vi "WS102x FPGA Multi DUT Reliability Ver2.0.vi"() -> ()   [LabVIEW 2017]
uses:
  Type Def/Test Sequences.ctl
  WS_VCAP Driver 039/Source/WSVCAP Shell/Type Defs/WSVCAP SHL FPGA Enum.ctl
  <vilib>/userdefined/High Color/nirio_resource_hc.ctl
  WS_VCAP Driver 039/Source/WSVCAP Shell/Type Defs/WSVCAP SHL I2C DUT Mask Mode Enum.ctl
  <vilib>/Utility/error.llb/whitespace.ctl
  <vilib>/Utility/file.llb/Read Delimited Spreadsheet (DBL).vi
panel:
  out "Die Y":string[](array[string])
  out "Die X":string[](array[string])
  in  "Main":T1(tab)
  in  "Clock Rate Meas(Hz)":dbl=1000000.0 format="%.1p Hz"
  in  "CAPDAC Value":u8=128 format="0x%02x"
  in  "DUT Mask Mode (All)":T2=enum."All"
  in  "SN Brd B":string[](array[string])=["1", "2", "3", "4", "5", "6", "7", "8", "9", "10", "11", "12", "13", "14", "15", "16", "17", "18", "19", "20", "21", "22", "23", "24", "25", "26", "27", "28", "29", "30", "31", "32"]
  in  "SN Brd A":string[](array[string])=["1", "2", "3", "4", "5", "6", "7", "8", "9", "10", "11", "12", "13", "14", "15", "16", "17", "18", "19", "20", "21", "22", "23", "24", "25", "26", "27", "28", "29", "30", "31", "32"]
  in  "Info Brd B":T3={"Lot #"="1K3CB", "Wafer #"="9", "Board"="B", "Comment"="CYC 25C 44V", "File Name"="CYC_1K3CB_9_WO_25C_44V_25DC_Brd2B_190417_1", "Data File Path Control"=path "C:/WS102x 32 DUT Data"}
  in  "Info Brd A":T3={"Lot #"="3127C", "Wafer #"="11", "Board"="A", "Comment"="CYC 25C 44V", "File Name"="CYC_3127C_11_BC-C_25C_44V_8KHz_50DC_Brd7A_201215_1", "Data File Path Control"=path "C:/WS102x 32 DUT Data"}
  in  "Test Program":string="WS102x FPGA Multi DUT Reliability Ver2.0"
  in  "Calibration AD":bool
  in  "Initialize ADI":bool
  in  "Data Brd B?":bool
  in  "Data Brd A?":bool=TRUE
  in  "Setup Test":T4(tab)
  in  "Manual Command":string
  in  "Verify Beams":bool
  in  "Manual Setting":i32(ring) items=["CP OFF", "CP ON", "OTP OFF", "CP 24V", "CP 26V", "CP 28V", "CP 30V", "CP 31V", "CP 32V", "CP 33V", "CP 34V", "CP 35V", "CP 36V", "CP 37V", "CP 38V", "CP 39V", "CP 40V", "CP 41V", "CP 42V", "CP 43V", "CP 44V", "CP 45V", "CP 46V", "CP 47V", "CP 48V", "CP 49V", "CP 50V", "CP 51V", "CP 52V", "CP 53V", "CP 54V", "CP 56V", "CP 58V", "CP 60V", "CP 62V"]
  in  "CP Measurement":i32(ring)=20 items=["CP OFF", "CP ON", "OTP OFF", "CP 24V", "CP 26V", "CP 28V", "CP 30V", "CP 31V", "CP 32V", "CP 33V", "CP 34V", "CP 35V", "CP 36V", "CP 37V", "CP 38V", "CP 39V", "CP 40V", "CP 41V", "CP 42V", "CP 43V", "CP 44V", "CP 45V", "CP 46V", "CP 47V", "CP 48V", "CP 49V", "CP 50V", "CP 51V", "CP 52V", "CP 53V", "CP 54V", "CP 56V", "CP 58V", "CP 60V", "CP 62V"]
  in  "Select CP VPI":i32(ring)=16 items=["CP OFF", "CP ON", "OTP OFF", "CP 24V", "CP 26V", "CP 28V", "CP 30V", "CP 31V", "CP 32V", "CP 33V", "CP 34V", "CP 35V", "CP 36V", "CP 37V", "CP 38V", "CP 39V", "CP 40V", "CP 41V", "CP 42V", "CP 43V", "CP 44V", "CP 45V", "CP 46V", "CP 47V", "CP 48V", "CP 49V", "CP 50V", "CP 51V", "CP 52V", "CP 53V", "CP 54V", "CP 56V", "CP 58V", "CP 60V", "CP 62V"]
  in  "Select CP Stress":i32(ring)=20 items=["CP OFF", "CP ON", "OTP OFF", "CP 24V", "CP 26V", "CP 28V", "CP 30V", "CP 31V", "CP 32V", "CP 33V", "CP 34V", "CP 35V", "CP 36V", "CP 37V", "CP 38V", "CP 39V", "CP 40V", "CP 41V", "CP 42V", "CP 43V", "CP 44V", "CP 45V", "CP 46V", "CP 47V", "CP 48V", "CP 49V", "CP 50V", "CP 51V", "CP 52V", "CP 53V", "CP 54V", "CP 56V", "CP 58V", "CP 60V", "CP 62V"]
  in  "VDD":dbl=3.3 format="%.2g"
  in  "CP Setting":bool
  in  "Delay Setting":T5(ring)
  in  "HD Cmd":string="0701027F7F"
  in  "Cycle DC %":string="50"
  in  "Set Delay Speed":dbl[](array[numeric])=[5.4e-05, 5.4e-05] min=0.0 max=0.5 format="%#.0p s"
  in  "Cycling Bit":string[](array[string])=["0701027F7F", "0701020000"]
  out "Stress DC(%)":string
  in  "HD Beams":string="ALL Beams"
  in  "Test Condition Setting":T6={"Freq (KHz)"="8", "ACV (V)"="0", "AC Freq (Hz)"="0", "Temp (C)"="25", "DCV (V)"=0.0, "CYC RP (x1000)"=10000, "HD RP (Min)"=60, "RPM Delay (s)"=60, "Select VCmin"=2} {"Select VCmin" items=["FBs", "TBs", "ALL"]}
  out "Test Run Selected":T7
  in  "Test Run Setting":T8={"OTP ?  "=FALSE, "STRESS ?  "=TRUE, "VPI ?  "=TRUE, "OPEN STATE VCMIN ?  "=FALSE, "CLOSE STATE VCMIN ?  "=TRUE, "RPM (Verify Socket) ?  "=FALSE, "HS CHK?"=FALSE}
  out "Data Board B":string[][](array[string])
  in  "Stop":bool
  out "Current Time":string
  out "Current Date":string
  in  "Start Date":string
  in  "Start Time":string
  in  "Select Measurement":i32(ring) items=["Temperature", "Humidity", "TH1", "TH2"]
  out "Temp (C)":string
  out "RH(%)":string
  out "Test Sequences":T9
  out "Error Out":errorcluster
  in  "Error In":errorcluster
  in  "Start":bool
  out "Data Board A":string[][](array[string])
  out "AD7747 Value Brd B":string[][](table)=[["Device", "Status", "Cap (pF)", "SN"], ["DUT 01", "", "", "01"], ["DUT 02", "", "", "02"], ["DUT 03", "", "", "03"], ["DUT 04", "", "", "04"], ["DUT 05", "", "", "05"], ["DUT 06", "", "", "06"], ["DUT 07", "", "", "07"], ["DUT 08", "", "", "08"], ["DUT 09", "", "", "09"], ["DUT 10", "", "", "10"], ["DUT 11", "", "", "11"], ["DUT 12", "", "", "12"], ["DUT 13", "", "", "13"], ["DUT 14", "", "", "14"], ["DUT 15", "", "", "15"], ["DUT 16", "", "", "16"], ["DUT 17", "", "", "17"], ["DUT 18", "", "", "18"], ["DUT 19", "", "", "19"], ["DUT 20", "", "", "20"], ["DUT 21", "", "", "21"], ["DUT 22", "", "", "22"], ["DUT 23", "", "", "23"], ["DUT 24", "", "", "24"], ["DUT 25", "", "", "25"], ["DUT 26", "", "", "26"], ["DUT 27", "", "", "27"], ["DUT 28", "", "", "28"], ["DUT 29", "", "", "29"], ["DUT 30", "", "", "30"], ["DUT 31", "", "", "31"], ["DUT 32", "", "", "32"]]
  out "AD7747 Value Brd A":string[][](table)=[["Device", "Status", "Cap (pF)", "SN"], ["DUT 01", "", "", "01"], ["DUT 02", "", "", "02"], ["DUT 03", "", "", "03"], ["DUT 04", "", "", "04"], ["DUT 05", "", "", "05"], ["DUT 06", "", "", "06"], ["DUT 07", "", "", "07"], ["DUT 08", "", "", "08"], ["DUT 09", "", "", "09"], ["DUT 10", "", "", "10"], ["DUT 11", "", "", "11"], ["DUT 12", "", "", "12"], ["DUT 13", "", "", "13"], ["DUT 14", "", "", "14"], ["DUT 15", "", "", "15"], ["DUT 16", "", "", "16"], ["DUT 17", "", "", "17"], ["DUT 18", "", "", "18"], ["DUT 19", "", "", "19"], ["DUT 20", "", "", "20"], ["DUT 21", "", "", "21"], ["DUT 22", "", "", "22"], ["DUT 23", "", "", "23"], ["DUT 24", "", "", "24"], ["DUT 25", "", "", "25"], ["DUT 26", "", "", "26"], ["DUT 27", "", "", "27"], ["DUT 28", "", "", "28"], ["DUT 29", "", "", "29"], ["DUT 30", "", "", "30"], ["DUT 31", "", "", "31"], ["DUT 32", "", "", "32"]]
  in  "Instruments":T11={"KE2400"="GPIB0::3::INSTR", "KE2000"="GPIB0::9::INSTR", "Agilent P/S"="GPIB0::5::INSTR", "Temperature Sensor"="", "FPGA"=enum."RIO0"}
  out "Activity Log":string
  out "FPGA Resource":T12
  out "Online":bool
  out "Simulate FPGA":bool
  in  "RFFE Slave Address":u8=7 caption="Slave Address" format="0x%02x"
  in  "Clock Rate Cycle(Hz)":dbl=5000000.0 format="%.1p Hz"
  out "Error Status":string
  out "IDD Measurement(uA)":string[](array[string])
  out "Cycle Count":u64=2 min=1 max=4 step=1
  out "Status":string
  out "Last Run Time":string
  out "Last Run Date":string
  out "T0_Brd B Delta C%":string[](array[string])
  out "T0_Brd A Delta C%":string[](array[string])
  in  "Abort Stress":bool
  out "TTF Completed":u64
  in  "Set TTF":u64=50000000000
  out "Brd B_VPI Cap (fF)":string[][](table)
  out "Brd B_Beam Cap (fF)":string[][](table)
  out "Brd A_VPI Cap (fF)":string[][](table)
  out "Brd A_Beam Cap (fF)":string[][](table)
  out "Verify CP Stress":string[](array[string])
  out "Brd B Pass/Fail?":bool[](array[boolean])
  out "Brd A Pass/Fail?":bool[](array[boolean])
  out "Verify DC Speed":dbl[](array[numeric]) format="%#.0p s"
  out "Verify Bits to Cycle":string[](array[string])
  out "Brd A Delta C%":string[](array[string])
  out "Brd B Delta C%":string[](array[string])
  out "Brd B_OS_V3 (fF)":string[][](table)
  out "Brd B_OS_V2 (fF)":string[][](table)
  out "Brd B_OS_V1 (fF)":string[][](table)
  in  "OS_Voltage(V)":dbl[](array[numeric])=[-10.0, 0.0, 10.0]
  out "Brd A_OS_V3 (fF)":string[][](table)
  out "Brd A_OS_V2 (fF)":string[][](table)
  out "Brd A_OS_V1 (fF)":string[][](table)
  out "VPI Brd B Delta C%":string[](array[string])
  out "VPI Brd A Delta C%":string[](array[string])
  out "Cmin BrdB":string[](array[string])
  out "Cmin BrdA":string[](array[string])
  out "RB for HD Stress":string[][](array[string])
  out "Brd B_CS_V3 (fF)":string[][](table)
  out "Brd B_CS_V2 (fF)":string[][](table)
  out "Brd B_CS_V1 (fF)":string[][](table)
  out "Brd A_CS_V3 (fF)":string[][](table)
  out "Brd A_CS_V2 (fF)":string[][](table)
  out "Brd A_CS_V1 (fF)":string[][](table)
  in  "CS_Voltage(V)":dbl[](array[numeric])=[-3.0, 0.0, 3.0]
  out "CMin BrdA (fF)":dbl[](array[numeric])
  out "CMin BrdB (fF)":dbl[](array[numeric])
  out "RB Die Y\nBrd B":string[](array[string])
  out "RB Die X\nBrd B":string[](array[string])
  out "RB Die Y\nBrd A":string[](array[string])
  out "Brd B_CS VCmin":string[][](table)
  out "Brd A_CS VCmin":string[][](table)
  out "Brd B_CS VCmin_T0":string[][](table)
  out "Brd A_CS VCmin_T0":string[][](table)
  out "RB Die X\nBrd A":string[](array[string])
  in  "RB Die Location?":bool=TRUE
  in  "Col CMin":i32=29
  out "Board B":dbl[][](graph)
  out "Board A":dbl[][](graph)
  in  "Plot":T13(ring)
  # "Company: WiSpry Inc Powered by AAC Technologies\n20 Fairbanks Suite 198, Irvine CA 92618\n\nCreated Date:  11-2-2021\nTP:  WS1021 32 DUT Board, Reliability Ver2.0\nFPGA Modular:  WS_VCAP_Driver 039"
  # "WS1021 FPGA 32 DUT Reliability Version Updated note:\n\n1. Ver1.0 :  Original version to run HD only (1-24-2019)\n2. Ver1.5 :  Delay Setting; Added CN, CMax (Total) and Cmin2 (12/15/2020), Minerva1"
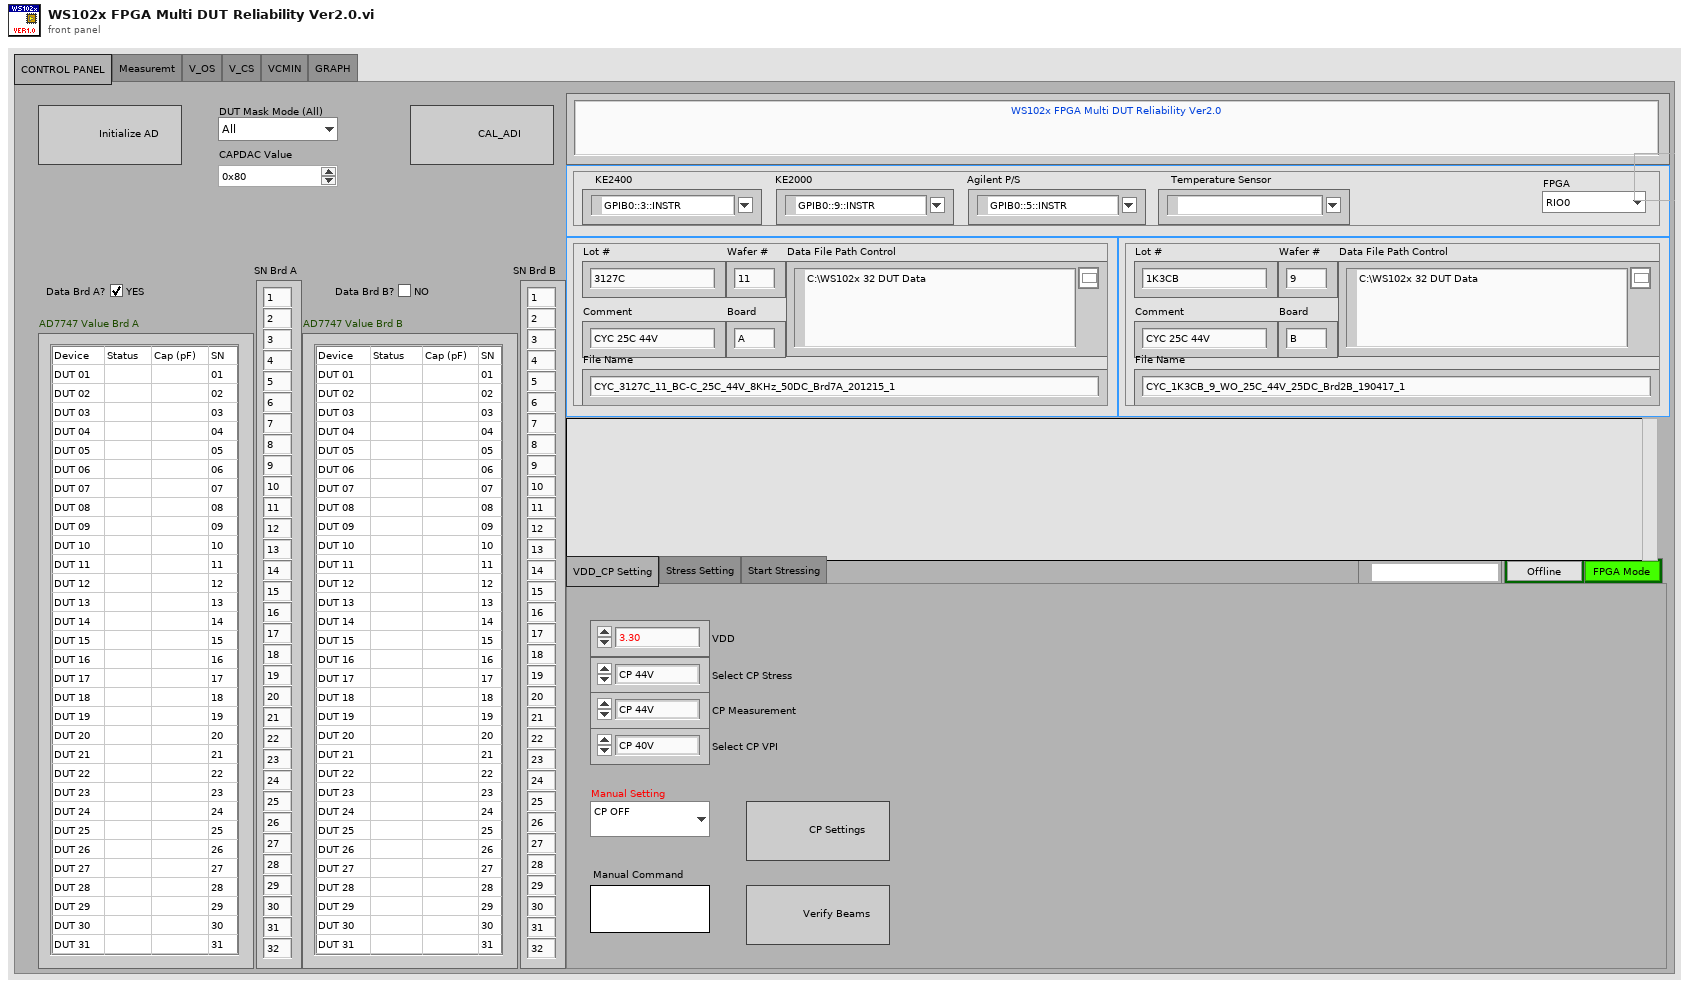
[diagram p1: front panel]
types:
  T1 = enum32{"CONTROL PANEL", "Measuremt", "V_OS", "V_CS", "VCMIN", "GRAPH"}
  T2 = typedef "WSVCAP SHL I2C DUT Mask Mode Enum.ctl" = enum16{"Custom", "All"}
  T3 = cluster{"Lot #":string, "Wafer #":string, "Board":string, "Comment":string, "File Name":string, "Data File Path Control":path}
  T4 = enum32{"VDD_CP Setting", "Stress Setting", "Start Stressing"}
  T5 = enum16{"Default (2.5us)", "0us", "4.8us", "5.26us"}
  T6 = cluster{"Freq (KHz)":string, "ACV (V)":string, "AC Freq (Hz)":string, "Temp (C)":string, "DCV (V)":dbl, "CYC RP (x1000)":u64, "HD RP (Min)":u64, "RPM Delay (s)":u64, "Select VCmin":u16}
  T7 = cluster{"OTP":bool, "CYC/HD":bool, "VPI":bool, "OSV":bool, "CSV":bool, "RPM":bool, "HS CHK":bool}
  T8 = cluster{"OTP ?  ":bool, "STRESS ?  ":bool, "VPI ?  ":bool, "OPEN STATE VCMIN ?  ":bool, "CLOSE STATE VCMIN ?  ":bool, "RPM (Verify Socket) ?  ":bool, "HS CHK?":bool}
  T9 = typedef "Test Sequences.ctl" = enum16{"VDD", "CP Setting", "HS CHK", "Stress", "I_Measure", "Cap_Measure", "VPI", "Open State VCmin", "Close State VCmiin", "Save Data", "Exit"}
  T10 = typedef "WSVCAP SHL FPGA Enum.ctl" = enum16{"RIO0", "RIO1"}
  T11 = cluster{"KE2400":refnum<visa-resource-name>, "KE2000":refnum<visa-resource-name>, "Agilent P/S":refnum<visa-resource-name>, "Temperature Sensor":refnum<visa-resource-name>, "FPGA":T10}
  T12 = typedef "nirio_resource_hc.ctl" = tag
  T13 = enum16{"ALL DUTs", "DUT 01", "DUT 02", "DUT 03", "DUT 04", "DUT 05", "DUT 06", "DUT 07", "DUT 08", "DUT 09", "DUT 10", "DUT 11", "DUT 12", "DUT 13", "DUT 14", "DUT 15", "DUT 16", "DUT 17", "DUT 18", "DUT 19", "DUT 20", "DUT 21", "DUT 22", "DUT 23", "DUT 24", "DUT 25", "DUT 26", "DUT 27", "DUT 28", "DUT 29", "DUT 30", "DUT 31", "DUT 32"}
  T14 = enum16{"Idle...", "Voltage 1", "Voltage 2", "Voltage 3"}
  T15 = typedef "WSVCAP SHL Core System Cluster.ctl" = cluster{"Settings":T16, "FPGA Resource":tag, "Online":bool, "I2C Wait Ticks":u32, "SPI Wait Ticks":u32, "RFFE Wait Ticks":u32, "FPGA VI Reference (FPGA Mode)":T17, "FPGA VI Reference (Sim Mode)":refnum<vi>}
  T16 = typedef "WSVCAP SHL I2C Settings Cluster.ctl" = cluster{"I2C Slave Address":u8, "I2C Clock Rate (Hz)":dbl, "SPI Clock Rate (Hz)":dbl, "RFFE Slave Address":u8, "RFFE Clock Rate (Hz)":dbl, "Simulate FPGA":bool, "C1 Cap DAC Default":u8, "C2 Cap DAC Default":u8, "C3 Cap DAC Default":u8, "C4 Cap DAC Default":u8}
  T17 = typedef "WSVCAP SHL FPGA Ref.ctl" = refnum<k20>
  T18 = enum16{"Idle...", "Voltage 1", "Voltage 2", "Voltage 3"}[]
  T19 = typedef "whitespace.ctl" = u16
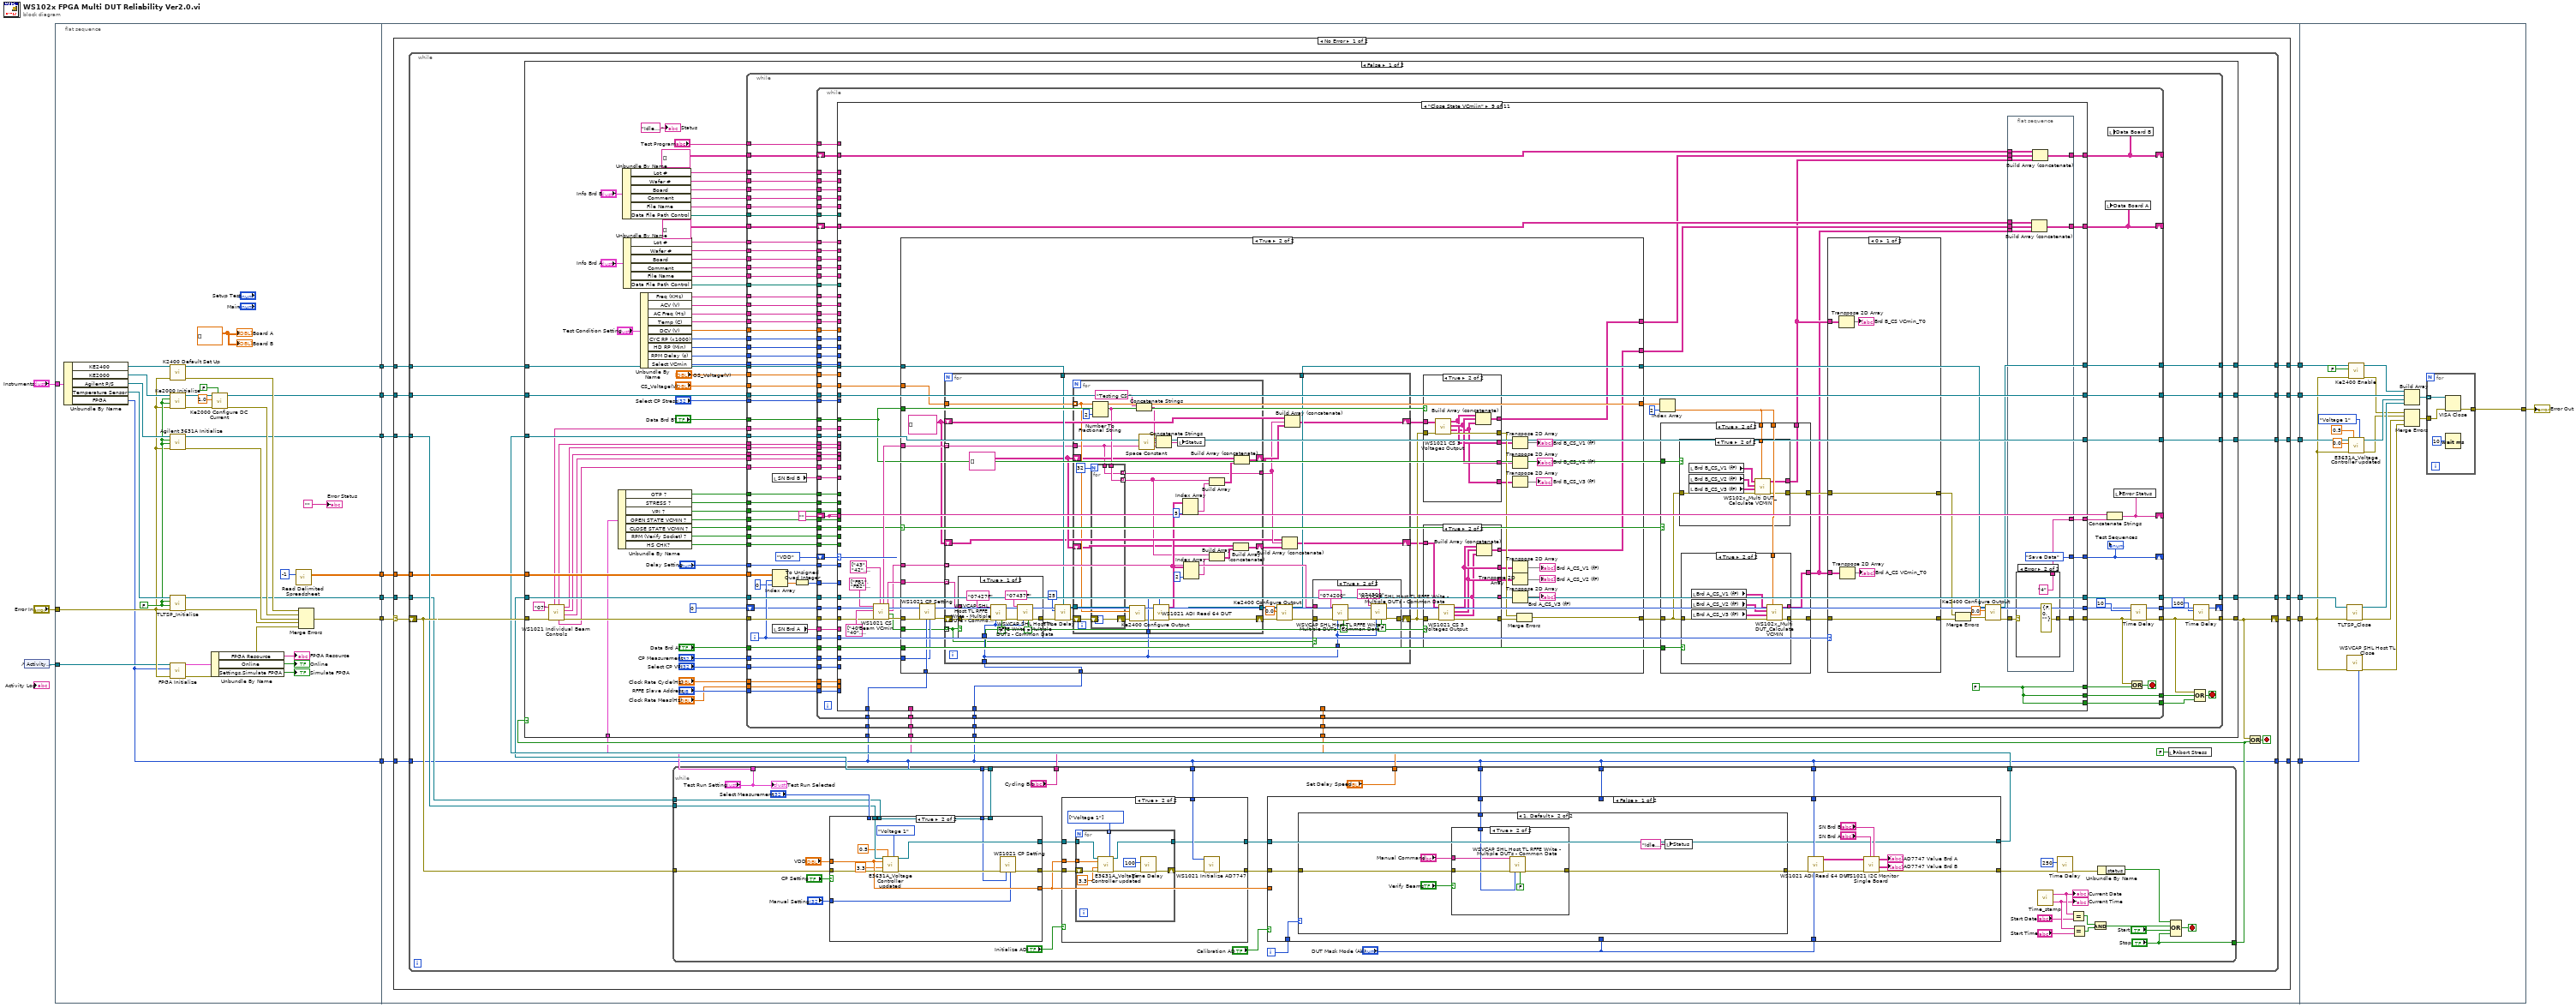
[diagram p0: block diagram]
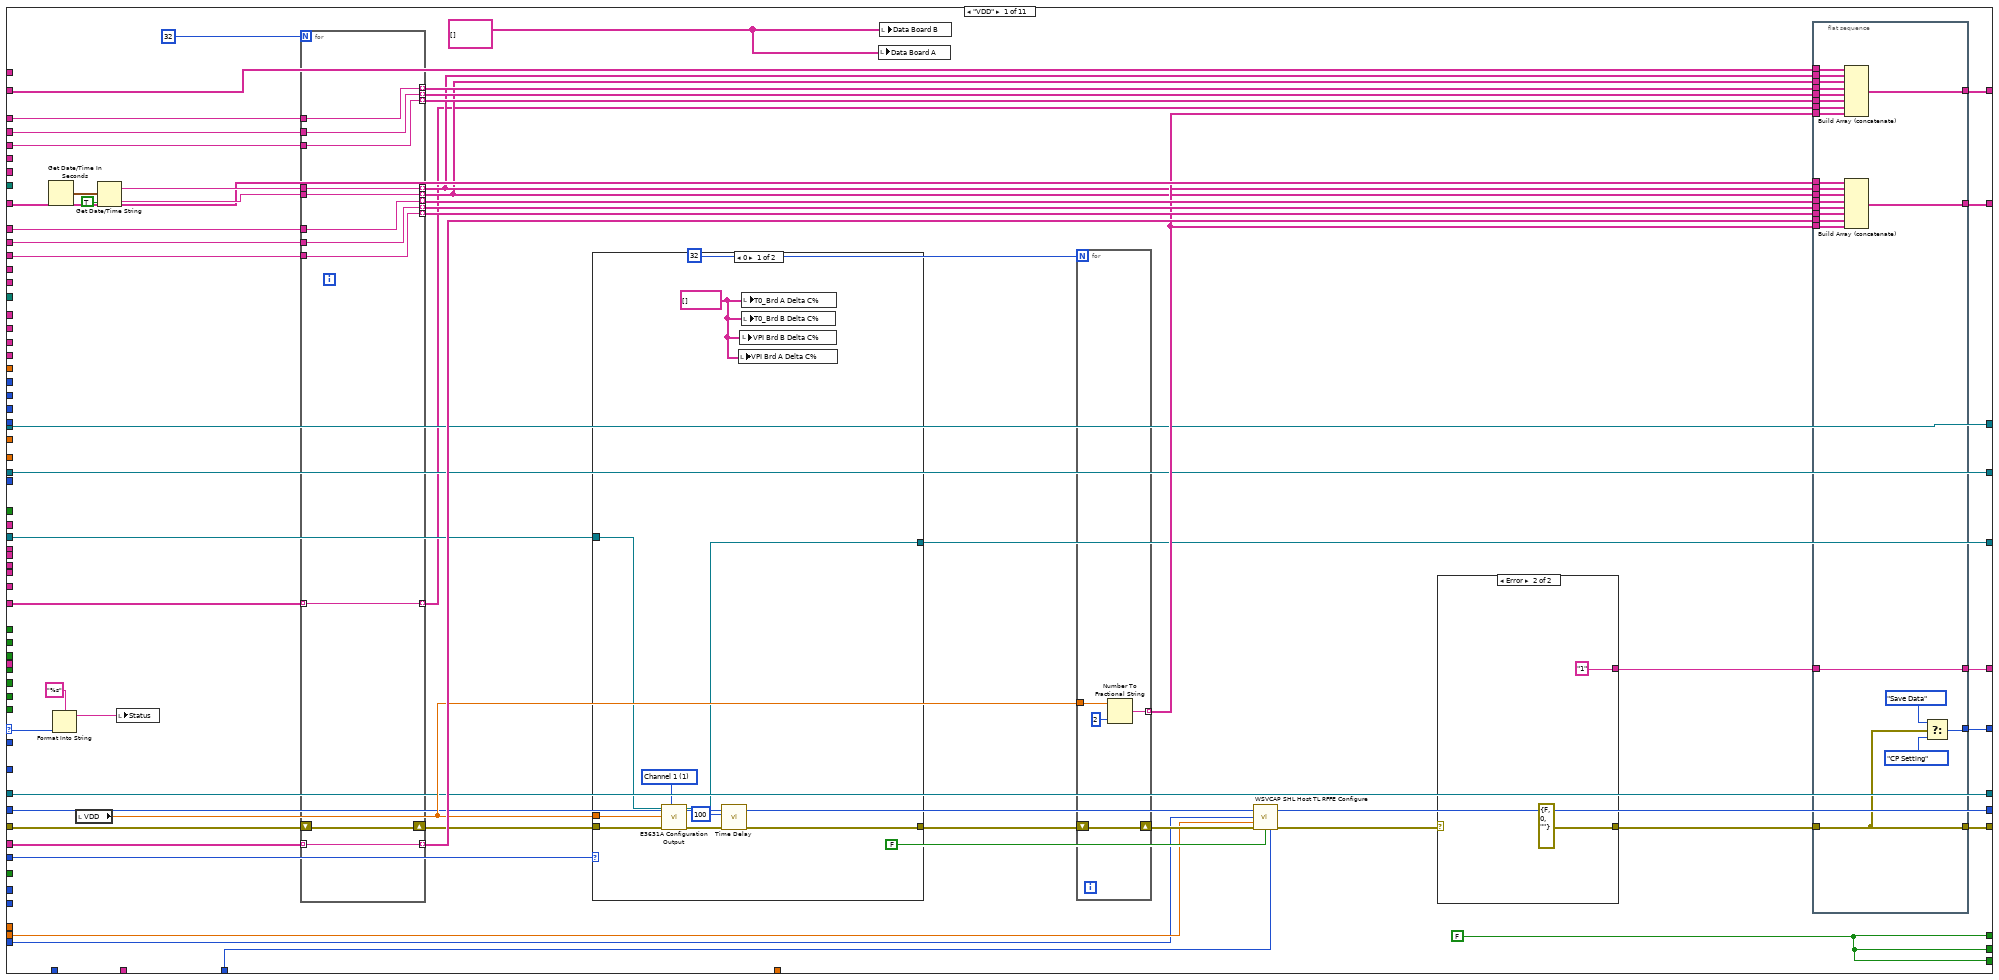
[diagram p2: hidden frame]
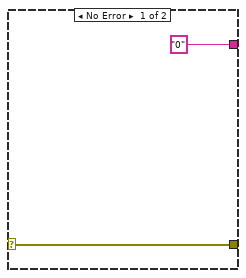
[diagram p3: hidden frame]
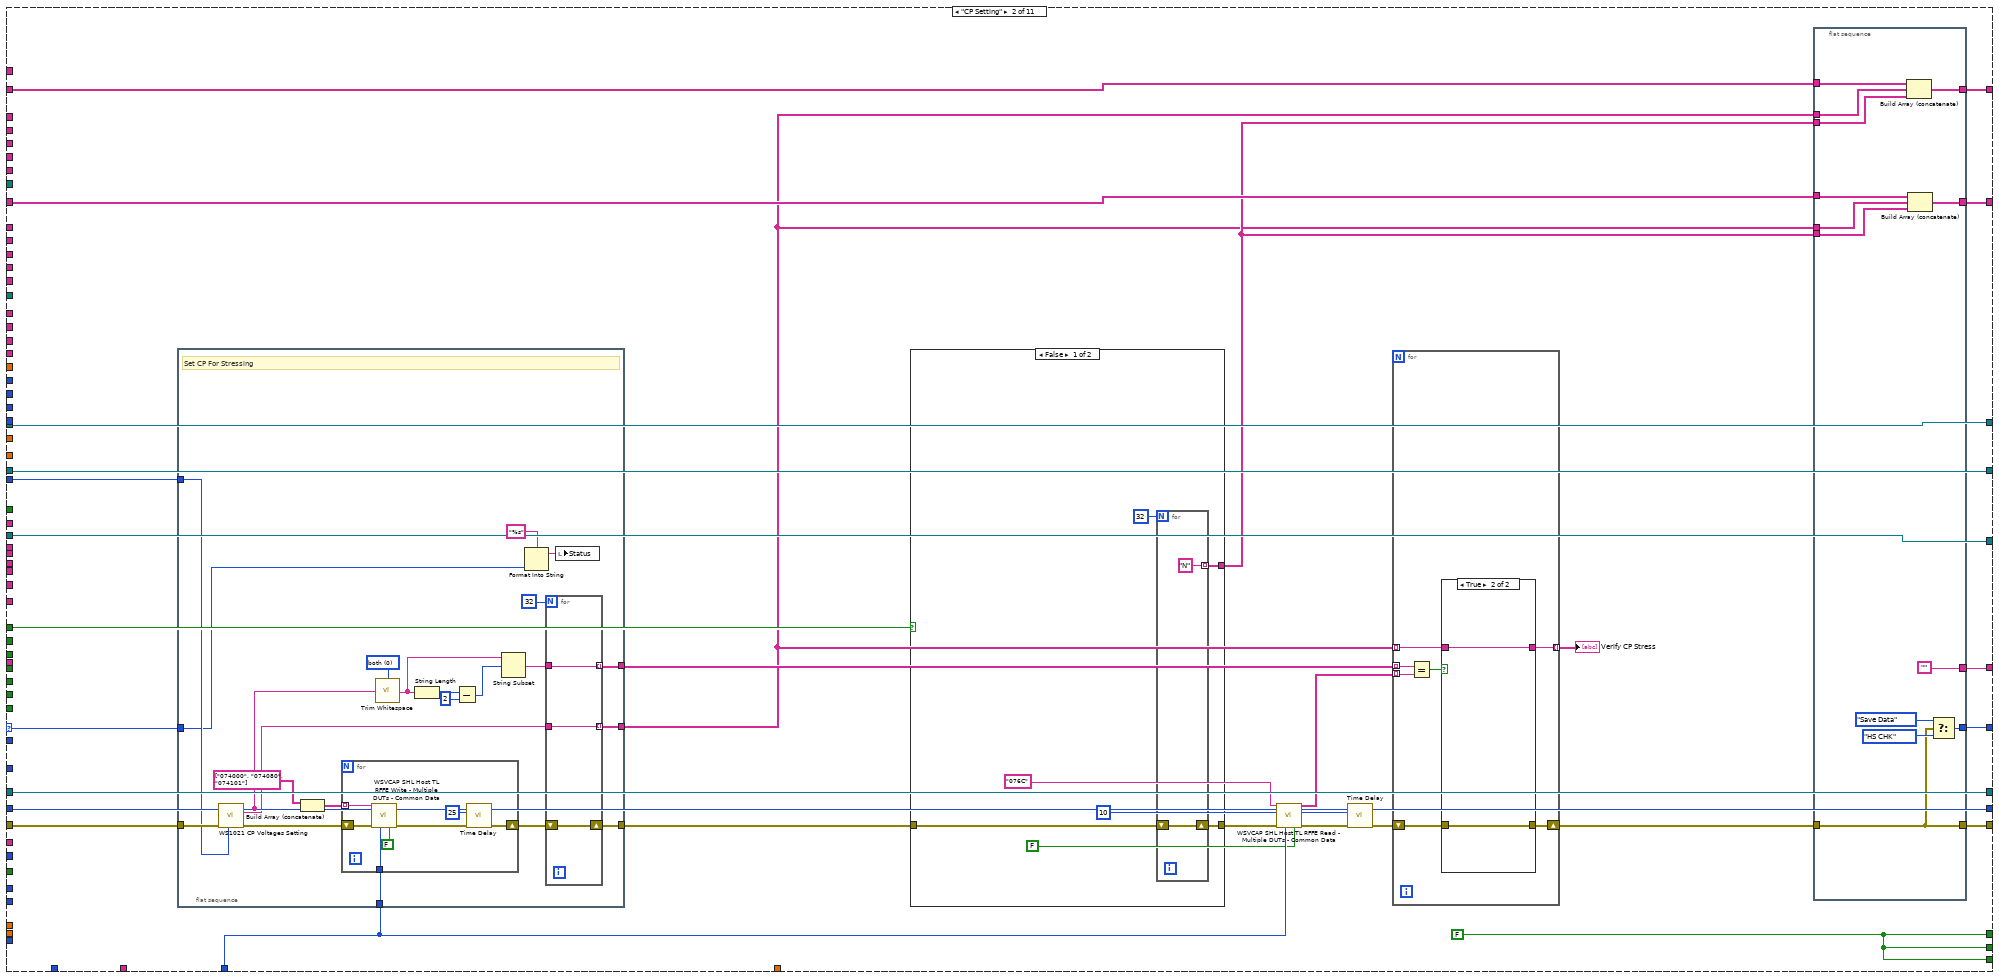
[diagram p5: hidden frame]
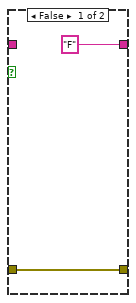
[diagram p6: hidden frame]
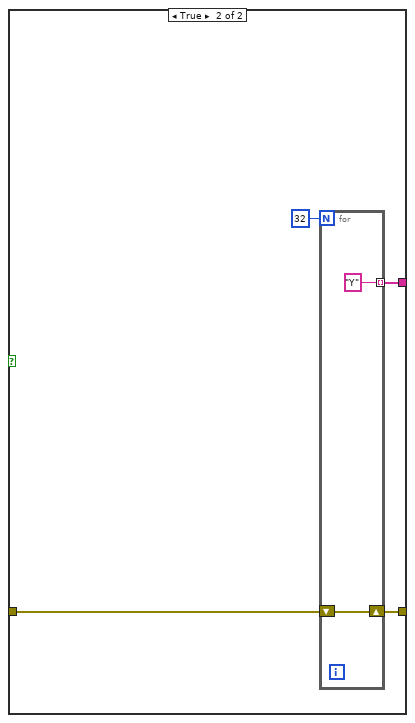
[diagram p7: hidden frame]
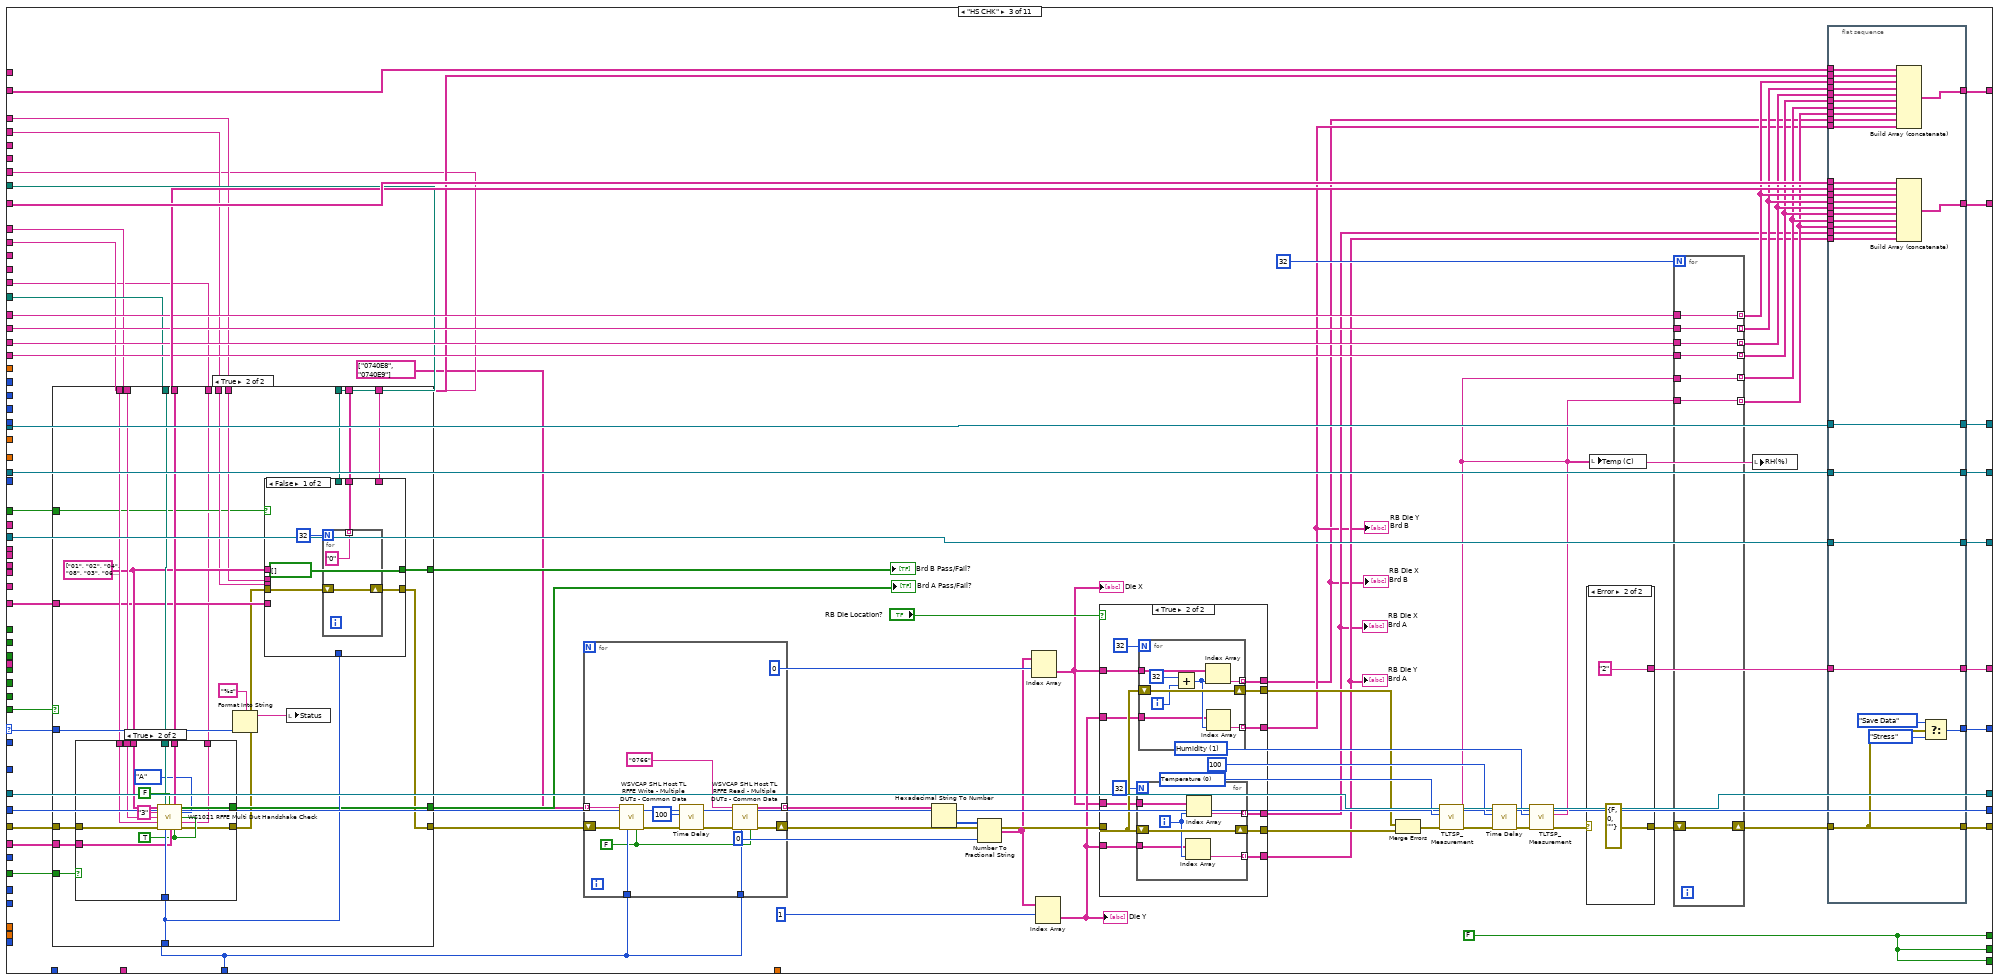
[diagram p8: hidden frame]
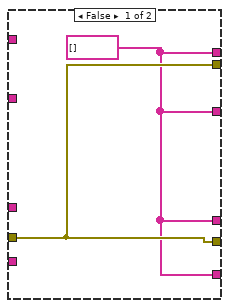
[diagram p9: hidden frame]
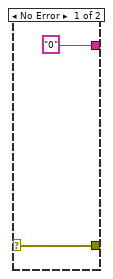
[diagram p10: hidden frame]
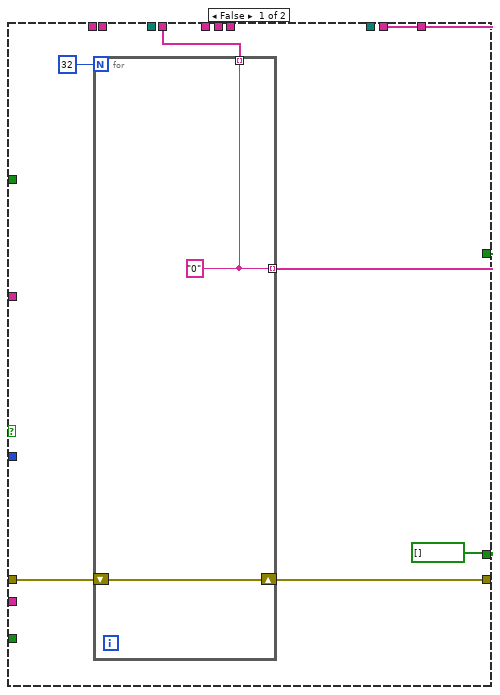
[diagram p11: hidden frame]
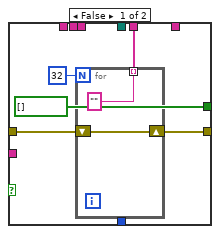
[diagram p12: hidden frame]
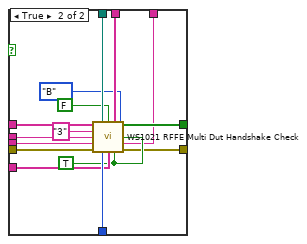
[diagram p13: hidden frame]
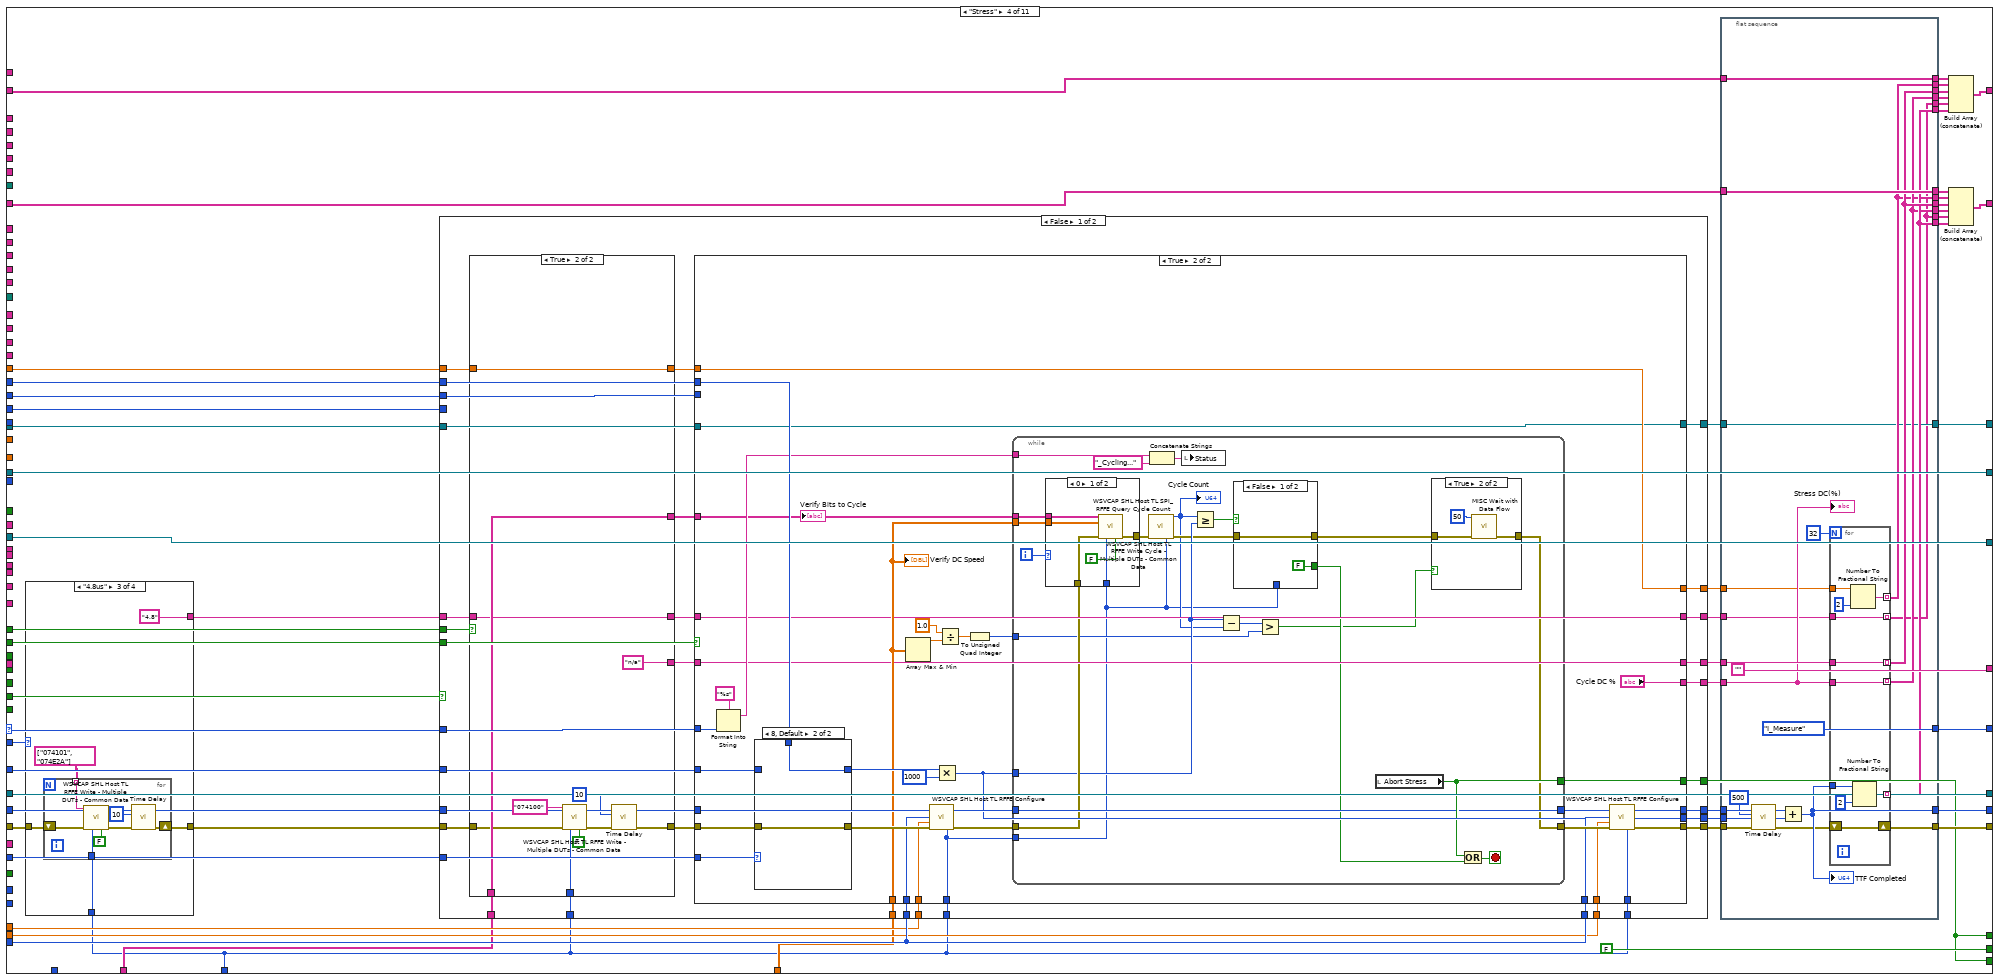
[diagram p14: hidden frame]
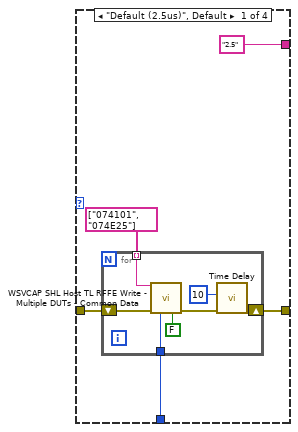
[diagram p15: hidden frame]
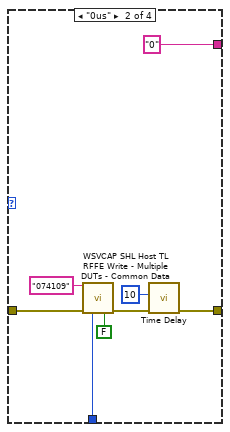
[diagram p16: hidden frame]
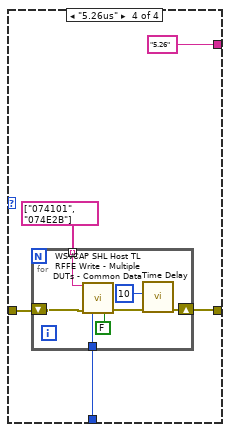
[diagram p17: hidden frame]
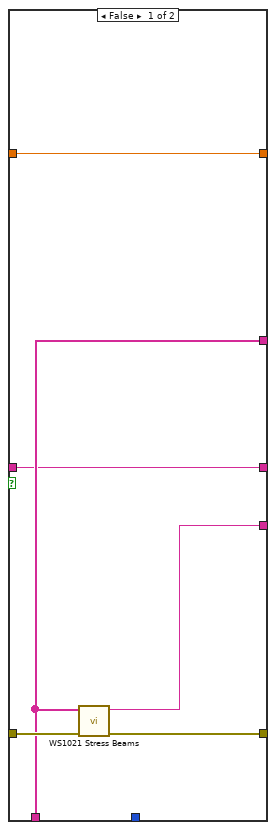
[diagram p18: hidden frame]
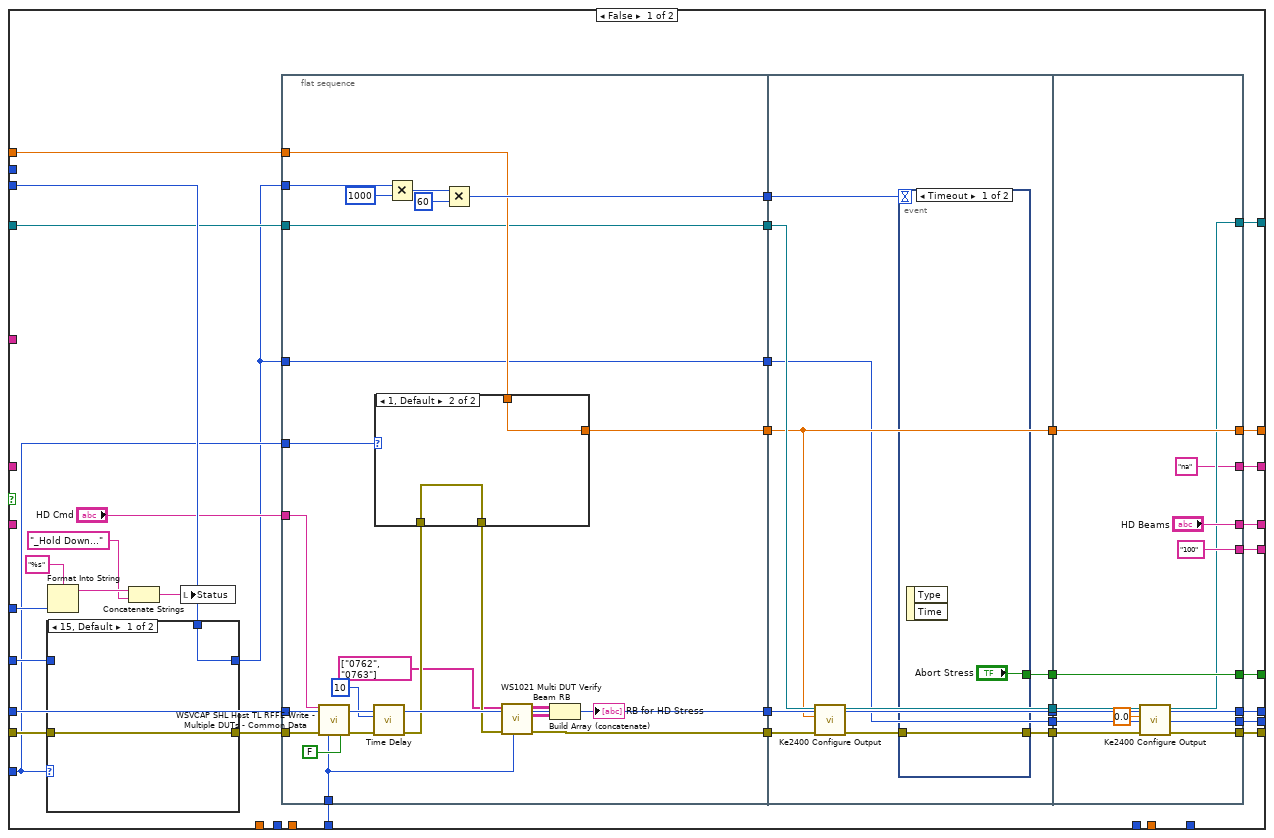
[diagram p19: hidden frame]
diagram:
  n1 = control-ref of="Activity Log"() -> (w3:refnum<vi>)
  n2 = flat-sequence {
    tunnel: [w35] -> w17
    tunnel: "Instruments" -> [w48]
    tunnel: "Error In" -> [w26]
    tunnel: [w32] -> w12
    tunnel: [w31] -> w11
    tunnel: [w30] -> w10
    tunnel: [w29] -> w9
    tunnel: [w27] -> w4
    tunnel: w3 -> [w24]
    tunnel: [w19] -> w2
    tunnel: w17 -> [w61]
    tunnel: [w60] -> w16
    tunnel: w12 -> [w59]
    tunnel: w11 -> [w58]
    tunnel: w10 -> [w57]
    tunnel: w9 -> [w56]
    tunnel: [w55] -> w8
    tunnel: [w54] -> w7
    tunnel: [w53] -> w6
    tunnel: [w52] -> w5
    tunnel: w4 -> [w51]
    tunnel: w2 -> [w50]
    tunnel: [w49] -> w1
    tunnel: w16 -> [w2354]
    tunnel: [w2355] -> w15
    tunnel: w8 -> [w2370]
    tunnel: w7 -> [w2366]
    tunnel: w6 -> [w2363]
    tunnel: w5 -> [w2371]
    tunnel: w1 -> [w2353]
    frame #0 {
      w42 = FALSE ("Reset")
      w47 = dbl[][] [] ("Board 1")
      n3 = Unbundle By Name(w48) -> ("KE2400"=w46:refnum<visa-resource-name>, "KE2000"=w45:refnum<visa-resource-name>, "Agilent P/S"=w44:refnum<visa-resource-name>, "Temperature Sensor"=w43:refnum<visa-resource-name>, "FPGA"=w19:T10)
      n4 = call "K2400 Default Set Up.vi"("Error In"=w26, "Ke2400 In"=w46) -> ("Error Out"=w39:errorcluster, "Ke2400 Out"=w32:refnum<visa-resource-name>)  [unwired: 8 in]
      n5 = call "Ke2000 Initialize.vi"("error in (no error)"=w26, "Default Setting"=w42, "Reset"=w42, "VISA resource name"=w45) -> ("error out"=w40:errorcluster, "VISA resource name out"=w41:refnum<visa-resource-name>)  [unwired: 6 in]
      n6 = call "Agilent 3631A Initialize.vi"("error in (no error)"=w26, "Default"=w42, "Reset"=w42, "VISA resource name"=w44) -> ("error out"=w37:errorcluster, "VISA resource name out"=w30:refnum<visa-resource-name>)  [unwired: 6 in]
      n7 = call "TLTSP_Initialize.vi"("error in (no error)"=w26, "Query ID?"=w42, "Reset"=w42, "VISA In"=w43) -> ("error out"=w36:errorcluster, "VISA Out"=w29:refnum<visa-resource-name>)  [unwired: 5 in, 1 out]
      n8 = call "FPGA Initialize.vi"("Error In"=w26, "FPGA"=w19, "Active Log"=w24) -> ("Error Out"=w25:errorcluster, "System Out"=w23:T15)  [unwired: 7 in]
      n9 = Unbundle By Name(w23) -> ("FPGA Resource"=→"FPGA Resource":tag, "Online"=→"Online":bool, "Settings.Simulate FPGA"=→"Simulate FPGA":bool)
      n10 = call "Ke2000 Configure DC Current.vi"("Auto Range? (T: Auto)"=FALSE, "error in"=w40, "Custom Range (0 A)"=1.0, "VISA resource name"=w41) -> ("error out"=w38:errorcluster, "VISA resource name out"=w31:refnum<visa-resource-name>)  [unwired: 6 in]
      n11 = call-poly <vilib>:"Read Delimited Spreadsheet.vi"("number of rows (all:-1)"=-1) -> ("all rows"=w27:dbl[][])  [unwired: 9 in, 5 out]
      n12 = Merge Errors(w39, w38, w37, w36, w25) -> (w35:errorcluster)
      "Board B" <- w47
      "Board A" <- w47
      "Error Status" <- ""
    }
    frame #1 {
      n13 = case shown="No Error" w61 {
        selector: w61 -> [w73 w2348]
        tunnel: [w74 w2347] -> w60
        tunnel: w59 -> [w72 w2346]
        tunnel: w58 -> [w71 w2345]
        tunnel: w57 -> [w70 w2344]
        tunnel: w56 -> [w69 w2343]
        tunnel: [w68 w2344] -> w55
        tunnel: [w67 w2346] -> w54
        tunnel: [w66 w2345] -> w53
        tunnel: [w65 w2343] -> w52
        tunnel: w51 -> [w64 _]
        tunnel: w50 -> [w63 w2342]
        tunnel: [w62 w2342] -> w49
        frame No Error {
          n14 = while {
            shift-right: [w92] -> w74
            shift-left: w73 -> [w94]
            tunnel: w72 -> [w90]
            tunnel: w71 -> [w89]
            tunnel: w70 -> [w88]
            tunnel: w69 -> [w82]
            tunnel: [w87] -> w68
            tunnel: [w86] -> w67
            tunnel: [w85] -> w66
            tunnel: [w84] -> w65
            tunnel: w64 -> [w83]
            tunnel: w63 -> [w75]
            tunnel: [w75] -> w62
            stop <- w93 stop-if-true
            n15 = while {
              tunnel: w94 -> [w2227]
              tunnel: ["Stop"] -> w91
              tunnel: w82 -> [w2209]
              tunnel: w88 -> [w2208]
              tunnel: w75 -> [w2197]
              tunnel: [w2199] -> w81
              tunnel: [w2198] -> w80
              tunnel: w75 -> [w2196]
              tunnel: w75 -> [w2195]
              tunnel: w75 -> [w2194]
              tunnel: ["Set Delay Speed"] -> w79
              tunnel: ["Cycling Bit"] -> w78
              tunnel: ["Test Run Setting"] -> w77
              tunnel: w75 -> [w2189]
              i -> [w2203]
              stop <- w2226 stop-if-true
              n16 = case shown="True" "CP Setting" {
                tunnel: w2227 -> [w2328 w2341]
                tunnel: [w2329 w2335] -> w2211
                tunnel: "VDD" -> [w2316 w2336]
                tunnel: "Select Measurement" -> [w2323 _]
                tunnel: w2209 -> [w2320 w2338]
                tunnel: w2208 -> [w2318 w2340]
                tunnel: [w2319 w2338] -> w2198
                tunnel: [w2318 w2339] -> w2205
                tunnel: [w2316 w2336] -> w2200
                tunnel: w2197 -> [_ w2333]
                tunnel: "Manual Setting" -> [_ w2332]
                frame False {
                  w2317 = 1 items=["Temperature", "Humidity", "TH1", "TH2"] ("Select Measurement")
                  n17 = call "TLTSP_Measurement.vi"("error in (no error)"=w2328, "Select Measurement"=w2323, "VISA resource name"=w2320) -> ("error out"=w2325:errorcluster, "Output"=→"Temp (C)":string, "VISA resource name out"=w2327:refnum<visa-resource-name>)  [unwired: 6 in]
                  n18 = call "Time Delay.vi"("Error In"=w2325, "Delay(ms)"=u32 100) -> ("Error Out"=w2326:errorcluster)  [unwired: 9 in]
                  n19 = call "TLTSP_Measurement.vi"("error in (no error)"=w2326, "Select Measurement"=w2317, "VISA resource name"=w2327) -> ("error out"=w2329:errorcluster, "Output"=→"RH(%)":string, "VISA resource name out"=w2319:refnum<visa-resource-name>)  [unwired: 6 in]
                }
                frame True {
                  n20 = call "E3631A_Voltage Controller updated.vi"("VISA resource name"=w2340, "I_VDD(A)"=0.5, "Channel Controller"=T14."Voltage 1", "Voltage 1"=w2336, "Voltage 2"=3.3, "error in (no error)"=w2341) -> ("VISA resource name out"=w2339:refnum<visa-resource-name>, "error out"=w2334:errorcluster)  [unwired: 8 in]
                  n21 = call "WS1021 CP Setting.vi"("Manual Setting"=w2332, "FPGA"=w2333, "Error In"=w2334) -> ("Error Out"=w2335:errorcluster)  [unwired: 7 in, 1 out]
                }
              }
              n22 = case shown="True" "Initialize ADI" {
                tunnel: w2211 -> [w2298 w2306]
                tunnel: [w2298 w2301] -> w2210
                tunnel: w2205 -> [w2297 w2305]
                tunnel: w2200 -> [_ w2304]
                tunnel: w2196 -> [_ w2300]
                tunnel: [w2297 w2299] -> w2201
                frame False {
                }
                frame True {
                  w2303 = T18 [enum."Voltage 1"] items=["Idle...", "Voltage 1", "Voltage 2", "Voltage 3"]
                  n23 = for {
                    tunnel: w2305 -> [w2313]
                    tunnel: w2304 -> [w2312]
                    tunnel: w2303 -> [w2311] mode=indexing
                    shift-right: [w2309] -> w2302
                    shift-left: w2306 -> [w2315]
                    tunnel: [w2307] -> w2299
                    n24 = call "E3631A_Voltage Controller updated.vi"("VISA resource name"=w2313, "Channel Controller"=w2311, "Voltage 1"=w2312, "Voltage 2"=3.3, "error in (no error)"=w2315) -> ("VISA resource name out"=w2307:refnum<visa-resource-name>, "error out"=w2310:errorcluster)  [unwired: 9 in]
                    n25 = call "Time Delay.vi"("Error In"=w2310, "Delay(ms)"=u32 100) -> ("Error Out"=w2309:errorcluster)  [unwired: 9 in]
                  }
                  n26 = call "WS1021 Initialize AD7747.vi"("Error In"=w2302, "FPGA"=w2300) -> ("Error Out"=w2301:errorcluster)  [unwired: 9 in]
                }
              }
              n27 = case shown="False" "Calibration AD" {
                tunnel: w2210 -> [w2233 w2274]
                tunnel: [w2238 w2269] -> w2204
                tunnel: w2194 -> [w2235 _]
                tunnel: w2203 -> [w2234 _]
                tunnel: w2195 -> [_ w2272]
                tunnel: "DUT Mask Mode (All)" -> [w2231 _]
                tunnel: "DUT Mask Mode (All)" -> [_ w2271]
                tunnel: w2201 -> [w2230 w2268]
                tunnel: w2200 -> [_ w2267]
                tunnel: [w2230 w2264] -> w2199
                tunnel: w2189 -> [w2229 _]
                frame False {
                  n28 = case shown="1, Default" w2234 {
                    tunnel: w2233 -> [w2251 w2256]
                    tunnel: [w2251 w2255] -> w2232
                    tunnel: w2229 -> [_ w2253]
                    frame 0 {
                      w2243 = string[] [] ("Cmin BrdB")
                      w2244 = dbl[] [] ("CMin BrdA")
                      w2246 = string[][] [] ("Brd B_CS VCmin_T0")
                      w2247 = string[][] [] ("Brd B_OS_V3 (fF)")
                      w2245 = string[] [] ("Brd B Delta C%")
                      w2248 = string[][] [] ("Brd B_Beam Cap (fF)")
                      w2249 = string[][] [] ("Data Board A")
                      w2250 = dbl[][] [] ("Board B")
                      n29 = local write "RB Die X\nBrd A"(w2243) -> ()
                      n30 = local write "RB Die Y\nBrd A"(w2243) -> ()
                      n31 = local write "RB Die Y\nBrd B"(w2243) -> ()
                      n32 = local write "RB Die X\nBrd B"(w2243) -> ()
                      n33 = local write "Cmin BrdA"(w2243) -> ()
                      n34 = local write "Cmin BrdB"(w2243) -> ()
                      n35 = local write "Brd A_CS VCmin_T0"(w2246) -> ()
                      n36 = local write "Brd B_CS VCmin_T0"(w2246) -> ()
                      n37 = local write "Brd A_CS VCmin"(w2246) -> ()
                      n38 = local write "Brd A_CS_V1 (fF)"(w2246) -> ()
                      n39 = local write "Brd A_CS_V2 (fF)"(w2246) -> ()
                      n40 = local write "Brd A_CS_V3 (fF)"(w2246) -> ()
                      n41 = local write "Brd B_CS VCmin"(w2246) -> ()
                      n42 = local write "Brd B_CS_V1 (fF)"(w2246) -> ()
                      n43 = local write "Brd B_CS_V2 (fF)"(w2246) -> ()
                      n44 = local write "Brd B_CS_V3 (fF)"(w2246) -> ()
                      n45 = local write "Brd B_OS_V3 (fF)"(w2247) -> ()
                      n46 = local write "Brd B_OS_V2 (fF)"(w2247) -> ()
                      n47 = local write "Brd B_OS_V1 (fF)"(w2247) -> ()
                      n48 = local write "Brd A_OS_V3 (fF)"(w2247) -> ()
                      n49 = local write "Brd A_OS_V1 (fF)"(w2247) -> ()
                      n50 = local write "Brd A_OS_V2 (fF)"(w2247) -> ()
                      n51 = local write "Brd B_Beam Cap (fF)"(w2248) -> ()
                      n52 = local write "Brd A_Beam Cap (fF)"(w2248) -> ()
                      n53 = local write "Brd B_VPI Cap (fF)"(w2248) -> ()
                      n54 = local write "Brd A_VPI Cap (fF)"(w2248) -> ()
                      n55 = local write "Brd B Delta C%"(w2245) -> ()
                      n56 = local write "Brd A Delta C%"(w2245) -> ()
                      n57 = local write "VPI Brd A Delta C%"(w2245) -> ()
                      n58 = local write "VPI Brd B Delta C%"(w2245) -> ()
                      n59 = local write "IDD Measurement(uA)"(w2245) -> ()
                      n60 = local write "CMin BrdA (fF)"(w2244) -> ()
                      n61 = local write "CMin BrdB (fF)"(w2244) -> ()
                      n62 = local write "Data Board A"(w2249) -> ()
                      n63 = local write "Data Board B"(w2249) -> ()
                      n64 = local write "Board B"(w2250) -> ()
                      n65 = local write "Board A"(w2250) -> ()
                    }
                    frame 1, Default {
                      n66 = case shown="True" "Verify Beams" {
                        tunnel: w2256 -> [w2258 w2263]
                        tunnel: [w2258 w2262] -> w2255
                        tunnel: w2253 -> [_ w2261]
                        tunnel: "Manual Command" -> [_ w2259]
                        frame False {
                        }
                        frame True {
                          n67 = call "WSVCAP SHL Host TL RFFE Write - Multiple DUTs - Common Data.vi"("Data Out"=w2259, "error in"=w2263, "FPGA"=w2261, "Log (T)"=FALSE) -> ("error out"=w2262:errorcluster)  [unwired: 11 in]
                        }
                      }
                      n68 = local write "Status"("Idle...." ("Status")) -> ()
                    }
                  }
                  n69 = call "WS1021 ADI Read 64 DUT.vi"("DUT Mask Mode (All)"=w2231, "FPGA"=w2235, "Error In"=w2232) -> ("Error Out"=w2237:errorcluster, "AD7747 Values"=w2236:string[][])  [unwired: 7 in]
                  n70 = call "WS1021 I2C Monitor Single Board.vi"("SN Brd B"="SN Brd B", "SN Brd A"="SN Brd A", "Error In"=w2237, "AD7747 Values"=w2236) -> ("Error Out"=w2238:errorcluster, "I2C Board B"=→"AD7747 Value Brd B":string[][], "I2C Board A"=→"AD7747 Value Brd A":string[][])  [unwired: 5 in]
                }
                frame True {
                  n71 = flat-sequence {
                    tunnel: w2274 -> [w2280]
                    tunnel: [w2279] -> w2273
                    tunnel: w2268 -> [w2278]
                    tunnel: w2267 -> [w2277]
                    tunnel: [w2275] -> w2266
                    tunnel: w2273 -> [w2290]
                    tunnel: w2272 -> [w2284]
                    tunnel: w2271 -> [w2285]
                    tunnel: [w2283] -> w2270
                    tunnel: w2266 -> [w2282]
                    tunnel: [w2282] -> w2265
                    tunnel: w2270 -> [w2296]
                    tunnel: [w2295] -> w2269
                    tunnel: w2265 -> [w2294]
                    tunnel: [w2291] -> w2264
                    frame #0 {
                      # "Set Voltage"
                      n72 = call "E3631A_Voltage Controller updated.vi"("VISA resource name"=w2278, "Channel Controller"=T14."Voltage 1", "Voltage 1"=w2277, "error in (no error)"=w2280) -> ("VISA resource name out"=w2275:refnum<visa-resource-name>, "error out"=w2279:errorcluster)  [unwired: 10 in]
                      n73 = One Button Dialog(message="Please verify all DUTs are empty...") -> ()  [unwired: 1 in, 1 out]
                    }
                    frame #1 {
                      # "Set ADI"
                      n74 = call "WS1021 ADI CAPDAC Setting.vi"("DUT Mask Mode (All)"=w2285, "FPGA"=w2284, "Error In"=w2290, "CAPDAC Value"="CAPDAC Value") -> ("Error Out"=w2288:errorcluster)  [unwired: 7 in]
                      n75 = call "WS1021 ADI OFFSET CAL.vi"("DUT Mask Mode (All)"=w2285, "FPGA"=w2284, "Error In"=w2288) -> ("Error Out"=w2287:errorcluster)  [unwired: 8 in]
                      n76 = call "Time Delay.vi"("Error In"=w2287, "Delay(ms)"=u32 100) -> ("Error Out"=w2283:errorcluster)  [unwired: 9 in]
                    }
                    frame #2 {
                      # "Set Voltage"
                      n77 = call "E3631A_Voltage Controller updated.vi"("VISA resource name"=w2294, "Channel Controller"=T14."Voltage 1", "Voltage 1"=0.0, "error in (no error)"=w2296) -> ("VISA resource name out"=w2291:refnum<visa-resource-name>, "error out"=w2295:errorcluster)  [unwired: 10 in]
                    }
                  }
                }
              }
              n78 = call "Time_stamp.vi"() -> ("date/time string"=w2223:string, "date string"=w2224:string)  [unwired: 2 in]
              "Current Time" <- w2223
              "Current Date" <- w2224
              n79 = call "Time Delay.vi"("Error In"=w2204, "Delay(ms)"=u32 250) -> ("Error Out"=w2207:errorcluster)  [unwired: 9 in]
              n80 = Equal?(x=w2224, y="Start Date") -> (x = y?=w2220:bool)
              n81 = Equal?(x=w2223, y="Start Time") -> (x = y?=w2219:bool)
              n82 = And(x=w2220, y=w2219) -> (x .and. y?=w2218:bool)
              n83 = Unbundle By Name(w2207) -> ("status"=w2225:bool)
              n84 = Compound Arithmetic op=OR(w2225, w2218, "Start", "Stop") -> (w2226:bool)
              "Test Run Selected" <- "Test Run Setting"
            }
            n85 = case shown="False" w91 {
              tunnel: w94 -> [w121 w2188]
              tunnel: [w165 w2188] -> w92
              tunnel: w90 -> [w150 w2187]
              tunnel: w89 -> [w146 w2186]
              tunnel: w81 -> [w149 w2185]
              tunnel: w80 -> [w144 w2184]
              tunnel: [w148 w2185] -> w87
              tunnel: [w147 w2187] -> w86
              tunnel: [w145 w2186] -> w85
              tunnel: [w143 w2184] -> w84
              tunnel: w83 -> [w123 _]
              tunnel: w75 -> [w105 _]
              tunnel: w75 -> [w102 _]
              tunnel: w79 -> [w98 _]
              tunnel: w78 -> [w97 _]
              tunnel: w77 -> [w96 _]
              frame False {
                n86 = call "WS1021 Individual Beam Controls.vi"("Error In"=w121, "USID"="07") -> ("Error Out"=w120:errorcluster, "Reg 2 Cmd"=w114:string[], "Reg 3 Cmd"=w115:string[], "Reg 2 Name"=w116:string[], "VPI_Cmd"=w113:string[], "Reg 3 Name"=w117:string[], "VPI_Name"=w118:string[])  [unwired: 3 in]
                n87 = Unbundle By Name(w96) -> ("OTP ?"=w156:bool, "STRESS ?"=w155:bool, "VPI ?"=w154:bool, "OPEN STATE VCMIN ?"=w153:bool, "CLOSE STATE VCMIN ?"=w152:bool, "RPM (Verify Socket) ?"=w151:bool, "HS CHK?"=w133:bool)
                n88 = Unbundle By Name("Info Brd B") -> ("Lot #"=w140:string, "Wafer #"=w139:string, "Board"=w138:string, "Comment"=w137:string, "File Name"=w136:string, "Data File Path Control"=w135:path)
                n89 = Unbundle By Name("Info Brd A") -> ("Lot #"=w162:string, "Wafer #"=w161:string, "Board"=w160:string, "Comment"=w159:string, "File Name"=w158:string, "Data File Path Control"=w157:path)
                n90 = Unbundle By Name("Test Condition Setting") -> ("Freq (KHz)"=w131:string, "ACV (V)"=w130:string, "AC Freq (Hz)"=w129:string, "Temp (C)"=w128:string, "DCV (V)"=w127:dbl, "CYC RP (x1000)"=w126:u64, "HD RP (Min)"=w125:u64, "RPM Delay (s)"=w124:u64, "Select VCmin"=w106:u16)
                n91 = while {
                  tunnel: w120 -> [w243]
                  tunnel: [w173] -> w165
                  tunnel: w156 -> [w241]
                  tunnel: w155 -> [w240]
                  tunnel: w154 -> [w239]
                  tunnel: w153 -> [w238]
                  tunnel: w152 -> [w237]
                  tunnel: w151 -> [w236]
                  tunnel: w162 -> [w235]
                  tunnel: w161 -> [w234]
                  tunnel: w160 -> [w233]
                  tunnel: w159 -> [w232]
                  tunnel: w158 -> [w231]
                  tunnel: "Test Program" -> [w230]
                  tunnel: w131 -> [w229]
                  tunnel: w130 -> [w228]
                  tunnel: w129 -> [w227]
                  tunnel: w128 -> [w226]
                  tunnel: w126 -> [w225]
                  tunnel: w124 -> [w224]
                  tunnel: w157 -> [w223]
                  tunnel: w150 -> [w222]
                  tunnel: w149 -> [w221]
                  tunnel: [w220] -> w148
                  tunnel: [w219] -> w147
                  tunnel: w146 -> [w218]
                  tunnel: [w217] -> w145
                  tunnel: w144 -> [w216]
                  tunnel: [w215] -> w143
                  tunnel: string[][] [] -> [w214]
                  tunnel: w140 -> [w213]
                  tunnel: w139 -> [w212]
                  tunnel: w138 -> [w211]
                  tunnel: w137 -> [w210]
                  tunnel: w136 -> [w209]
                  tunnel: w135 -> [w208]
                  tunnel: string[][] [] -> [w207]
                  tunnel: w133 -> [w206]
                  tunnel: w127 -> [w205]
                  tunnel: w125 -> [w204]
                  tunnel: w123 -> [w203]
                  shift-right: [w199] -> _
                  shift-left: u64 0 -> [w200]
                  tunnel: w118 -> [w196]
                  tunnel: w117 -> [w195]
                  tunnel: w116 -> [w194]
                  tunnel: w115 -> [w193]
                  tunnel: w114 -> [w192]
                  tunnel: w113 -> [w191]
                  tunnel: "Select CP Stress" -> [w190]
                  tunnel: "Data Brd B?" -> [w189]
                  tunnel: "Data Brd A?" -> [w188]
                  tunnel: "OS_Voltage(V)" -> [w187]
                  tunnel: "CS_Voltage(V)" -> [w186]
                  tunnel: w106 -> [w185]
                  tunnel: w105 -> [w184]
                  tunnel: "CP Measurement" -> [w183]
                  tunnel: "Select CP VPI" -> [w182]
                  tunnel: w102 -> [w181]
                  tunnel: "Clock Rate Cycle(Hz)" -> [w178]
                  tunnel: "RFFE Slave Address" -> [w177]
                  tunnel: "Clock Rate Meas(Hz)" -> [w176]
                  tunnel: w98 -> [w175]
                  tunnel: w97 -> [w174]
                  tunnel: "Delay Setting" -> [w166]
                  i -> [w202]
                  stop <- w171 stop-if-true
                  # "Read Points"
                  n92 = local read "SN Brd B"() -> (w179:string[])
                  n93 = Index Array(array=w203, index (row)=w202, index (col)=0 ("disabled index (col)")) -> (element=w197:dbl)
                  n94 = local read "SN Brd A"() -> (w180:string[])
                  n95 = To Unsigned Quad Integer(1:w197) -> (0:w198:u64)
                  n96 = while {
                    tunnel: w243 -> [w324]
                    tunnel: [w301] -> w170
                    shift-right: [w309] -> _
                    shift-left: Test_Sequences."VDD" ("Test Sequences") -> [w323]
                    tunnel: w241 -> [w322]
                    tunnel: w240 -> [w321]
                    tunnel: w239 -> [w320]
                    tunnel: w238 -> [w319]
                    tunnel: w237 -> [w318]
                    tunnel: w236 -> [w317]
                    tunnel: w235 -> [w316]
                    tunnel: w234 -> [w315]
                    tunnel: w233 -> [w314]
                    tunnel: w232 -> [w313]
                    tunnel: w231 -> [w312]
                    tunnel: w223 -> [w311]
                    tunnel: w230 -> [w310]
                    tunnel: w229 -> [w308]
                    tunnel: w228 -> [w307]
                    tunnel: w227 -> [w306]
                    tunnel: w226 -> [w305]
                    tunnel: w225 -> [w304]
                    tunnel: w204 -> [w303]
                    tunnel: w224 -> [w302]
                    tunnel: w222 -> [w299]
                    tunnel: w221 -> [w298]
                    tunnel: [w297] -> w220
                    tunnel: [w296] -> w219
                    tunnel: w218 -> [w295]
                    tunnel: [w294] -> w217
                    tunnel: w216 -> [w293]
                    tunnel: [w292] -> w215
                    tunnel: [w249] -> w169
                    tunnel: w202 -> [w288]
                    shift-right: [w250] -> _
                    shift-left: w214 -> [w287]
                    tunnel: w213 -> [w286]
                    tunnel: w212 -> [w285]
                    tunnel: w211 -> [w284]
                    tunnel: w210 -> [w283]
                    tunnel: w209 -> [w282]
                    tunnel: w208 -> [w281]
                    shift-right: [w251] -> _
                    shift-left: w207 -> [w280]
                    tunnel: w206 -> [w279]
                    tunnel: w205 -> [w278]
                    tunnel: w198 -> [w277]
                    tunnel: w200 -> [w276]
                    tunnel: [w275] -> w199
                    tunnel: w196 -> [w274]
                    tunnel: w195 -> [w273]
                    tunnel: w194 -> [w272]
                    tunnel: w193 -> [w271]
                    tunnel: w192 -> [w270]
                    tunnel: w191 -> [w269]
                    tunnel: w190 -> [w268]
                    tunnel: w189 -> [w267]
                    tunnel: w188 -> [w266]
                    tunnel: w187 -> [w265]
                    tunnel: w186 -> [w264]
                    tunnel: w185 -> [w263]
                    tunnel: w184 -> [w262]
                    tunnel: w183 -> [w261]
                    tunnel: w182 -> [w260]
                    tunnel: w181 -> [w259]
                    tunnel: w180 -> [w258]
                    tunnel: w179 -> [w257]
                    tunnel: w178 -> [w256]
                    tunnel: w177 -> [w255]
                    tunnel: w176 -> [w254]
                    tunnel: w175 -> [w253]
                    tunnel: w174 -> [w252]
                    tunnel: [w248] -> w168
                    shift-right: [w246] -> _
                    shift-left: "" -> [w245]
                    tunnel: w166 -> [w244]
                    stop <- w291 stop-if-true
                    # "Measurement"
                    n97 = case shown="\"Close State VCmiin\"" w323 {
                      selector: w323 -> [w341 w447 w573 w798 _ _ _ _ _ _ _]
                      tunnel: w324 -> [w370 w461 w598 w777 w1181 w1318 w1454 w1592 w1728 w2020 w2121]
                      tunnel: [w380 w464 w610 w823 w1190 w1353 w1460 w1599 w1745 w2032 w2098] -> w289
                      tunnel: [w379 w463 w611 w824 w1191 w1354 w1459 w1598 w1746 w2031 _] -> w309
                      tunnel: w322 -> [_ w462 _ w819 _ _ _ _ _ _ _]
                      tunnel: w321 -> [_ _ _ w820 _ _ _ _ _ _ _]
                      tunnel: w320 -> [_ _ _ _ _ _ w1450 _ _ _ _]
                      tunnel: w319 -> [_ _ _ _ _ _ _ w1593 _ _ _]
                      tunnel: w318 -> [_ _ _ _ _ _ _ _ w1711 _ _]
                      tunnel: w317 -> [_ _ _ w822 _ _ _ _ _ _ _]
                      tunnel: w316 -> [w372 _ w571 _ _ _ _ _ _ _ w2116]
                      tunnel: w315 -> [w371 _ w570 _ _ _ _ _ _ _ w2115]
                      tunnel: w314 -> [w358 _ _ _ _ _ _ _ _ _ _]
                      tunnel: w313 -> [_ _ _ _ _ _ _ _ _ w2014 _]
                      tunnel: w312 -> [_ _ w553 _ _ _ _ _ _ w2005 w2114]
                      tunnel: w311 -> [_ _ w572 _ _ _ _ _ _ w2011 w2096]
                      tunnel: w310 -> [_ _ _ _ _ _ _ _ _ w2017 _]
                      tunnel: w308 -> [_ _ w592 _ _ _ _ _ _ _ _]
                      tunnel: w307 -> [_ _ w593 _ _ _ _ _ _ _ _]
                      tunnel: w306 -> [_ _ w594 _ _ _ _ _ _ _ _]
                      tunnel: w305 -> [_ _ w595 _ _ _ _ _ _ _ _]
                      tunnel: w304 -> [_ _ _ w800 _ _ _ _ _ _ _]
                      tunnel: w303 -> [_ _ _ w811 _ _ _ _ _ _ _]
                      tunnel: w302 -> [_ _ _ w817 _ _ _ _ _ _ _]
                      tunnel: w299 -> [w344 w454 w605 w789 w1189 w1352 w1457 w1591 w1740 w2030 w2113]
                      tunnel: w298 -> [w353 w452 w601 w815 w1184 w1350 w1455 w1595 w1743 w2028 w2112]
                      tunnel: [w346 w452 w600 w815 w1184 w1350 w1455 w1595 w1743 w2028 w2111] -> w297
                      tunnel: [w344 w454 w604 w787 w1189 w1352 w1457 w1584 w1736 w2030 w2110] -> w296
                      tunnel: w295 -> [w345 w453 w603 w816 w1179 w1351 w1456 w1596 w1744 w2029 w2109]
                      tunnel: [w345 w453 w602 w816 w1178 w1351 w1456 w1596 w1744 w2029 w2109] -> w294
                      tunnel: w293 -> [w343 w451 w585 w814 w1183 w1348 w1458 w1594 w1742 w2027 w2108]
                      tunnel: [w343 w451 w580 w814 w1183 w1348 w1458 w1594 w1742 w2027 w2108] -> w292
                      tunnel: [w335 w435 w563 w780 w1164 w1311 w1431 w1564 w1712 w2003 TRUE ("true")] -> w290
                      tunnel: w288 -> [w355 _ _ w818 _ w1323 _ _ w1724 _ _]
                      tunnel: w287 -> [w373 w456 w607 w812 w1185 w1339 w1447 w1588 w1732 w1995 _]
                      tunnel: w286 -> [w366 _ w567 _ _ _ _ _ _ _ w2095]
                      tunnel: w285 -> [w365 _ w566 _ _ _ _ _ _ _ w2094]
                      tunnel: w284 -> [w364 _ _ _ _ _ _ _ _ _ _]
                      tunnel: w283 -> [_ _ _ _ _ _ _ _ _ w2016 _]
                      tunnel: w282 -> [_ _ w554 _ _ _ _ _ _ w2004 w2092]
                      tunnel: w281 -> [_ _ w569 _ _ _ _ _ _ w2012 _]
                      tunnel: w280 -> [w363 w458 w609 w813 w1188 w1341 w1448 w1589 w1734 w1994 _]
                      tunnel: [w360 w457 w608 w804 w1187 w1340 w1449 w1586 w1733 _ _] -> w251
                      tunnel: [w359 w455 w606 w803 w1186 w1338 w1446 w1587 w1731 _ _] -> w250
                      tunnel: w279 -> [_ _ w599 _ _ _ _ _ _ _ _]
                      tunnel: w278 -> [_ _ _ w797 _ _ _ _ _ _ _]
                      tunnel: w277 -> [_ _ _ w801 _ _ _ _ _ _ _]
                      tunnel: w276 -> [w342 w450 w574 w810 w1182 w1349 w1451 w1597 w1741 w2026 _]
                      tunnel: [w342 w450 w574 w807 w1182 w1349 w1451 w1597 w1741 w2026 w2106] -> w275
                      tunnel: w274 -> [_ _ _ _ _ _ w1453 _ _ w2006 _]
                      tunnel: w273 -> [_ _ _ _ _ w1344 _ _ _ w2008 _]
                      tunnel: w272 -> [_ _ _ _ _ w1343 _ _ _ w2007 _]
                      tunnel: w271 -> [_ _ _ _ _ w1347 _ _ _ _ _]
                      tunnel: w270 -> [_ _ _ _ _ w1346 _ _ _ _ _]
                      tunnel: w269 -> [_ _ _ _ _ _ w1452 _ _ _ _]
                      tunnel: w268 -> [_ w448 _ _ _ _ _ _ _ _ _]
                      tunnel: w267 -> [_ _ w560 _ w1160 w1309 w1423 w1557 w1705 w1991 w2097]
                      tunnel: w266 -> [_ _ w559 _ w1158 w1308 w1424 w1556 w1704 w1992 w2101]
                      tunnel: w265 -> [_ _ _ _ _ _ _ w1590 _ _ _]
                      tunnel: w264 -> [_ _ _ _ _ _ _ _ w1739 _ _]
                      tunnel: w263 -> [_ _ _ _ _ _ _ _ _ _ _]
                      tunnel: w262 -> [w329 w446 w545 w775 w1172 w1312 w1421 w1565 w1707 _ _]
                      tunnel: w261 -> [_ _ _ _ _ w1313 w1422 _ w1708 _ _]
                      tunnel: w260 -> [_ _ _ _ _ _ w1444 _ _ _ _]
                      tunnel: w259 -> [_ _ _ _ _ w1314 w1445 _ w1709 _ _]
                      tunnel: w258 -> [w336 _ w564 _ _ _ _ _ _ _ _]
                      tunnel: w257 -> [w338 _ w565 _ _ _ _ _ _ _ _]
                      tunnel: w256 -> [_ _ _ w785 _ _ _ _ _ _ _]
                      tunnel: w255 -> [w330 _ _ w786 _ _ _ _ _ _ _]
                      tunnel: w254 -> [w331 _ _ w784 _ _ _ _ _ _ _]
                      tunnel: w253 -> [_ _ _ w783 _ _ _ _ _ _ _]
                      tunnel: w252 -> [_ _ _ w782 _ _ _ _ _ _ _]
                      tunnel: [w335 w435 w563 FALSE ("true") w1164 w1311 w1431 w1564 w1712 w2003 w2104] -> w249
                      tunnel: [w335 w435 w563 w780 w1164 w1311 w1431 w1564 w1712 w2003 FALSE ("true")] -> w248
                      tunnel: [w325 w434 w555 "" w1163 w1310 w1426 w1559 w1706 w1990 ""] -> w247
                      tunnel: w245 -> [_ _ _ _ _ _ _ _ _ _ w2093]
                      tunnel: w244 -> [_ _ _ w778 _ _ _ _ _ _ _]
                      frame "VDD" {
                        w334 = string[][] [] ("Data Board B")
                        w335 = FALSE ("true")
                        n98 = Get Date/Time In Seconds() -> (seconds since 1Jan1904=w377:timestamp)
                        n99 = Format Into String(format string="%s", w341) -> (resulting string=w339:string)  [unwired: 2 in, 1 out]
                        n100 = local read "VDD"() -> (w352:dbl)
                        n101 = Get Date/Time String(seconds (now)=w377, want seconds? (F)=TRUE) -> (date string=w375:string, time string=w374:string)  [unwired: 1 in]
                        n102 = local write "Status"(w339) -> ()
                        n103 = for {
                          N: 32 -> [_]
                          tunnel: w375 -> [w410]
                          tunnel: w374 -> [w409]
                          tunnel: [w410] -> w348 mode=indexing
                          tunnel: [w409] -> w347 mode=indexing
                          tunnel: w372 -> [w407]
                          tunnel: w371 -> [w406]
                          shift-right: [w408] -> w354
                          shift-left: w370 -> [w408]
                          tunnel: [w400] -> w367 mode=indexing
                          tunnel: [w407] -> w369 mode=indexing
                          tunnel: [w406] -> w368 mode=indexing
                          tunnel: w366 -> [w405]
                          tunnel: [w405] -> w362 mode=indexing
                          tunnel: w365 -> [w404]
                          tunnel: [w404] -> w361 mode=indexing
                          tunnel: [w403] -> w356 mode=indexing
                          tunnel: w364 -> [w403]
                          tunnel: [w402] -> w357 mode=indexing
                          tunnel: w358 -> [w402]
                          tunnel: w338 -> [w401] mode=indexing
                          tunnel: [w401] -> w337 mode=indexing
                          tunnel: w336 -> [w400] mode=indexing
                        }
                        n104 = case shown="0" w355 {
                          tunnel: w354 -> [w397 w398]
                          tunnel: [w389 w398] -> w349
                          tunnel: w352 -> [w393 _]
                          tunnel: w353 -> [w392 w399]
                          tunnel: [w391 w399] -> w346
                          frame 0 {
                            w390 = string[] [] ("Brd A Delta C%")
                            w394 = 1 items=["Channel 1"=1, "Channel 2"=2, "Channel 3"=3] ("Channel (1: Channel 1)")
                            n105 = call "E3631A Configuration Output.vi"("Channel (1: Channel 1)"=w394, "error in (no error)"=w397, "Voltage Level (0.0 V)"=w393, "VISA resource name"=w392) -> ("error out"=w396:errorcluster, "VISA resource name out"=w391:refnum<visa-resource-name>)  [unwired: 6 in]
                            n106 = call "Time Delay.vi"("Error In"=w396, "Delay(ms)"=u32 100) -> ("Error Out"=w389:errorcluster)  [unwired: 9 in]
                            n107 = local write "VPI Brd A Delta C%"(w390) -> ()
                            n108 = local write "VPI Brd B Delta C%"(w390) -> ()
                            n109 = local write "T0_Brd A Delta C%"(w390) -> ()
                            n110 = local write "T0_Brd B Delta C%"(w390) -> ()
                          }
                          frame 1, Default {
                          }
                        }
                        n111 = local write "Data Board A"(w334) -> ()
                        n112 = local write "Data Board B"(w334) -> ()
                        n113 = for {
                          N: 32 -> [_]
                          tunnel: w352 -> [w388]
                          tunnel: [w386] -> w350 mode=indexing
                          shift-right: [w385] -> w332
                          shift-left: w349 -> [w385]
                          n114 = Number To Fractional String(number=w388, precision (6)=i16 2) -> (F-format string=w386:string)  [unwired: 2 in]
                        }
                        n115 = call "WSVCAP SHL Host TL RFFE Configure.vi"("RFFE Slave Address"=w330, "Clock Rate (Hz)"=w331, "error in"=w332, "Log (T)"=FALSE, "FPGA"=w329) -> ("error out"=w328:errorcluster)  [unwired: 9 in, 1 out]
                        n116 = case shown="Error" w328 {
                          selector: w328 -> [w382 _]
                          tunnel: [w382 errorcluster {"status"=FALSE, "code"=0, "source"=""} ("Error Out")] -> w327
                          tunnel: ["0" "1"] -> w326
                          frame No Error {
                          }
                          frame Error {
                          }
                        }
                        n117 = flat-sequence {
                          tunnel: w327 -> [w431]
                          tunnel: [w431] -> w380
                          tunnel: [w430] -> w379
                          tunnel: w373 -> [w429]
                          tunnel: w348 -> [w425]
                          tunnel: w347 -> [w424]
                          tunnel: w369 -> [w428]
                          tunnel: w368 -> [w427]
                          tunnel: w367 -> [w419]
                          tunnel: w363 -> [w426]
                          tunnel: w362 -> [w423]
                          tunnel: w361 -> [w422]
                          tunnel: w337 -> [w417]
                          tunnel: [w421] -> w360
                          tunnel: [w420] -> w359
                          tunnel: w357 -> [w418]
                          tunnel: w356 -> [w416]
                          tunnel: w350 -> [w415]
                          tunnel: w350 -> [w414]
                          tunnel: w348 -> [w413]
                          tunnel: w347 -> [w412]
                          tunnel: w326 -> [w411]
                          tunnel: [w411] -> w325
                          frame #0 {
                            n118 = Build Array (concatenate)(w426, w413, w412, w423, w422, w416, w417, w414) -> (w421:string[][])
                            n119 = Build Array (concatenate)(w429, w425, w424, w428, w427, w418, w419, w415) -> (w420:string[][])
                            n120 = Select(t=Test_Sequences."Save Data" ("Test Sequences"), s=w431, f=Test_Sequences."CP Setting" ("Test Sequences")) -> (s? t:f=w430:T9)
                          }
                        }
                      }
                      frame "CP Setting" {
                        w435 = FALSE ("true")
                        n121 = flat-sequence {
                          tunnel: w461 -> [w507]
                          tunnel: [w509] -> w460
                          tunnel: [w505] -> w438
                          tunnel: w448 -> [w506]
                          tunnel: w447 -> [w504]
                          tunnel: w446 -> [w498]
                          tunnel: [w491] -> w440
                          frame #0 {
                            w497 = T19 0 items=["both", "start of string", "end of string"] ("location (both)")
                            # "Set CP For Stressing"
                            n122 = call "WS1021 CP Voltages Setting.vi"("Select CPV"=w506, "Error In"=w507) -> ("Error Out"=w501:errorcluster, "CP Select"=w499:string, "Cmd Send out"=w489:string)  [unwired: 4 in, 3 out]
                            n123 = Build Array (concatenate)(string[] ["074000", "074080", "074101"], w489) -> (w488:string[])
                            n124 = for {
                              tunnel: w498 -> [w515]
                              shift-right: [w514] -> w500
                              shift-left: w501 -> [w516]
                              tunnel: w488 -> [w510] mode=indexing
                              n125 = call "WSVCAP SHL Host TL RFFE Write - Multiple DUTs - Common Data.vi"("Data Out"=w510, "error in"=w516, "FPGA"=w515, "Log (T)"=FALSE) -> ("error out"=w513:errorcluster)  [unwired: 11 in]
                              n126 = call "Time Delay.vi"("Error In"=w513, "Delay(ms)"=u32 25) -> ("Error Out"=w514:errorcluster)  [unwired: 9 in]
                            }
                            n127 = call <vilib>:"Trim Whitespace.vi"("string"=w489, "location (both)"=w497) -> ("trimmed string"=w493:string)
                            n128 = String Length(string=w493) -> (length=w496:i32)
                            n129 = Subtract(x=w496, y=2) -> (x-y=w494:i32)
                            n130 = String Subset(string=w493, offset (0)=w494) -> (substring=w492:string)  [unwired: 1 in]
                            n131 = Format Into String(format string="%s", w504) -> (resulting string=w502:string)  [unwired: 2 in, 1 out]
                            n132 = for {
                              N: 32 -> [_]
                              shift-right: [w519] -> w509
                              shift-left: w500 -> [w519]
                              tunnel: w499 -> [w518]
                              tunnel: [w518] -> w505 mode=indexing
                              tunnel: w492 -> [w517]
                              tunnel: [w517] -> w491 mode=indexing
                            }
                            n133 = local write "Status"(w502) -> ()
                          }
                        }
                        n134 = case shown="False" w462 {
                          tunnel: w460 -> [w479 w485]
                          tunnel: [w478 w484] -> w459
                          tunnel: [w476 w483] -> w449
                          frame False {
                            # "CP CYC, NO OTP"
                            n135 = for {
                              N: 32 -> [_]
                              shift-right: [w481] -> w478
                              shift-left: w479 -> [w481]
                              tunnel: ["N"] -> w476 mode=indexing
                            }
                          }
                          frame True {
                            # "CP CYC, OTP"
                            n136 = for {
                              N: 32 -> [_]
                              shift-right: [w487] -> w484
                              shift-left: w485 -> [w487]
                              tunnel: ["Y"] -> w483 mode=indexing
                            }
                          }
                        }
                        n137 = call "WSVCAP SHL Host TL RFFE Read - Multiple DUTs - Common Data.vi"("Data Out"="076C", "error in"=w459, "FPGA"=w446, "Log (T)"=FALSE) -> ("RFFE Data In"=w439:string[], "error out"=w444:errorcluster)  [unwired: 10 in]
                        n138 = call "Time Delay.vi"("Error In"=w444, "Delay(ms)"=u32 10) -> ("Error Out"=w441:errorcluster)  [unwired: 9 in]
                        n139 = for {
                          tunnel: w440 -> [w471] mode=indexing
                          tunnel: w439 -> [w470] mode=indexing
                          shift-right: [w467] -> w436
                          shift-left: w441 -> [w468]
                          tunnel: w438 -> [w466] mode=indexing
                          tunnel: [w465] -> w437 mode=indexing
                          n140 = Equal?(x=w471, y=w470) -> (x = y?=w469:bool)
                          n141 = case shown="True" w469 {
                            tunnel: w468 -> [w472 w475]
                            tunnel: [w472 w475] -> w467
                            tunnel: w466 -> [_ w474]
                            tunnel: ["F" ("CP Select") w474] -> w465
                            frame False {
                            }
                            frame True {
                            }
                          }
                        }
                        "Verify CP Stress" <- w437
                        n142 = flat-sequence {
                          tunnel: w436 -> [w530]
                          tunnel: [w530] -> w464
                          tunnel: [w529] -> w463
                          tunnel: w458 -> [w528]
                          tunnel: [w527] -> w457
                          tunnel: w456 -> [w526]
                          tunnel: [w525] -> w455
                          tunnel: w438 -> [w524]
                          tunnel: w438 -> [w523]
                          tunnel: w449 -> [w521]
                          tunnel: w449 -> [w522]
                          tunnel: [""] -> w434
                          frame #0 {
                            n143 = Build Array (concatenate)(w528, w523, w522) -> (w527:string[][])
                            n144 = Build Array (concatenate)(w526, w524, w521) -> (w525:string[][])
                            n145 = Select(t=Test_Sequences."Save Data" ("Test Sequences"), s=w530, f=Test_Sequences."HS CHK" ("Test Sequences")) -> (s? t:f=w529:T9)
                          }
                        }
                      }
                      frame "HS CHK" {
                        w582 = 1 items=["Temperature", "Humidity", "TH1", "TH2"] ("Select Measurement")
                        w583 = 0 items=["Temperature", "Humidity", "TH1", "TH2"] ("Select Measurement")
                        w563 = FALSE ("true")
                        n146 = case shown="True" w599 {
                          tunnel: w598 -> [w667 w687]
                          tunnel: [w666 w676] -> w552
                          tunnel: [w665 w691] -> w597
                          tunnel: w573 -> [_ w694]
                          tunnel: w572 -> [_ w690]
                          tunnel: w571 -> [_ w689]
                          tunnel: w570 -> [_ w688]
                          tunnel: w545 -> [_ w681]
                          tunnel: w569 -> [_ w686]
                          tunnel: [w664 w685] -> w568
                          tunnel: w567 -> [_ w683]
                          tunnel: w566 -> [_ w682]
                          tunnel: w565 -> [_ w680]
                          tunnel: w564 -> [_ w679]
                          tunnel: [w663 w678] -> w562
                          tunnel: [w663 w675] -> w561
                          tunnel: w560 -> [_ w674]
                          tunnel: w559 -> [_ w673]
                          tunnel: w554 -> [_ w672]
                          tunnel: w553 -> [_ w671]
                          frame False {
                            w663 = bool[] []
                            n147 = for {
                              N: 32 -> [_]
                              shift-right: [w670] -> w666
                              shift-left: w667 -> [w670]
                              tunnel: [w669] -> w665 mode=indexing
                              tunnel: [w669] -> w664 mode=indexing
                              w669 = "0"
                            }
                          }
                          frame True {
                            w684 = string[] ["01", "02", "04", "08", "03", "06", "0C", "07", "0E", "0F", "07", "03", "00"] ("HS CHK CNTRL")
                            n148 = case shown="True" w673 {
                              tunnel: [w695 w716] -> w691
                              tunnel: w690 -> [_ w714]
                              tunnel: w689 -> [_ w712]
                              tunnel: w688 -> [_ w711]
                              tunnel: w687 -> [w699 w710]
                              tunnel: w684 -> [_ w709]
                              tunnel: w681 -> [_ w708]
                              tunnel: w679 -> [_ w707]
                              tunnel: [bool[] [] ("Pass/Fail?") w706] -> w678
                              tunnel: [w698 w703] -> w677
                              tunnel: w671 -> [_ w702]
                              frame False {
                                n149 = for {
                                N: 32 -> [_]
                                shift-right: [w701] -> w698
                                shift-left: w699 -> [w701]
                                tunnel: [""] -> w695 mode=indexing
                                }
                              }
                              frame True {
                                w705 = TRUE ("Start")
                                n150 = call "WS1021 RFFE Multi Dut Handshake Check.vi"("HS CHK CNTRL"=w709, "TMN DC\\CAP Data Log File Path"=w714, "Debug?"=FALSE, "Set Register"="3", "Select Brd"=enum16{"A", "B"}."A", "Lot#"=w712, "Stop Button"=w705, "Wafer #"=w711, "File Name"=w702, "Error In"=w710, "FPGA"=w708, "SN#"=w707, "Start"=w705) -> ("Status"=w716:string[], "Pass/Fail?"=w706:bool[], "Error Out"=w703:errorcluster)
                              }
                            }
                            n151 = Format Into String(format string="%s", w694) -> (resulting string=w692:string)  [unwired: 2 in, 1 out]
                            n152 = case shown="False" w674 {
                              tunnel: w686 -> [_ w738]
                              tunnel: [w717 w737] -> w685
                              tunnel: w684 -> [_ w736]
                              tunnel: w683 -> [_ w734]
                              tunnel: w682 -> [_ w733]
                              tunnel: w681 -> [_ w732]
                              tunnel: w680 -> [_ w731]
                              tunnel: w677 -> [w721 w727]
                              tunnel: [w720 w726] -> w676
                              tunnel: [bool[] [] ("Pass/Fail?") w725] -> w675
                              tunnel: w672 -> [_ w724]
                              frame False {
                                n153 = for {
                                N: 32 -> [_]
                                shift-right: [w723] -> w720
                                shift-left: w721 -> [w723]
                                tunnel: ["0"] -> w717 mode=indexing
                                }
                              }
                              frame True {
                                w729 = TRUE ("Start")
                                n154 = call "WS1021 RFFE Multi Dut Handshake Check.vi"("HS CHK CNTRL"=w736, "TMN DC\\CAP Data Log File Path"=w738, "Debug?"=FALSE, "Set Register"="3", "Select Brd"=enum16{"A", "B"}."B", "Lot#"=w734, "Stop Button"=w729, "Wafer #"=w733, "File Name"=w724, "Error In"=w727, "FPGA"=w732, "SN#"=w731, "Start"=w729) -> ("Status"=w737:string[], "Pass/Fail?"=w725:bool[], "Error Out"=w726:errorcluster)
                              }
                            }
                            n155 = local write "Status"(w692) -> ()
                          }
                        }
                        "Brd A Pass/Fail?" <- w562
                        "Brd B Pass/Fail?" <- w561
                        n156 = for {
                          shift-right: [w617] -> w551
                          shift-left: w552 -> [w622]
                          tunnel: w545 -> [w619]
                          tunnel: string[] ["0740E8", "0740E9"] -> [w618] mode=indexing
                          tunnel: w545 -> [w614]
                          tunnel: [w613] -> w544 mode=indexing
                          w615 = FALSE ("Log (T)")
                          n157 = call "WSVCAP SHL Host TL RFFE Write - Multiple DUTs - Common Data.vi"("Data Out"=w618, "error in"=w622, "FPGA"=w619, "Log (T)"=w615) -> ("error out"=w621:errorcluster)  [unwired: 11 in]
                          n158 = call "Time Delay.vi"("Error In"=w621, "Delay(ms)"=u32 100) -> ("Error Out"=w612:errorcluster)  [unwired: 9 in]
                          n159 = call "WSVCAP SHL Host TL RFFE Read - Multiple DUTs - Common Data.vi"("Data Out"="0766", "error in"=w612, "FPGA"=w614, "Log (T)"=w615) -> ("RFFE Data In"=w613:string[], "error out"=w617:errorcluster)  [unwired: 10 in]
                        }
                        n160 = Hexadecimal String To Number(string=w544) -> (number=w543:u32[][])  [unwired: 2 in, 1 out]
                        n161 = Number To Fractional String(number=w543, precision (6)=i16 0) -> (F-format string=w539:string[][])  [unwired: 2 in]
                        n162 = Index Array(array=w539, index (row)=0) -> (element=w537:string[])  [unwired: 1 in]
                        "Die X" <- w537
                        n163 = Index Array(array=w539, index (row)=1) -> (element=w538:string[])  [unwired: 1 in]
                        "Die Y" <- w538
                        n164 = case shown="True" "RB Die Location?" {
                          tunnel: w551 -> [w624 w637]
                          tunnel: w537 -> [_ w636]
                          tunnel: [w624 w635] -> w549
                          tunnel: [w624 w634] -> w548
                          tunnel: [w623 w633] -> w533
                          tunnel: [w623 w632] -> w535
                          tunnel: w538 -> [_ w629]
                          tunnel: [w623 w628] -> w534
                          tunnel: w538 -> [_ w627]
                          tunnel: w537 -> [_ w626]
                          tunnel: [w623 w625] -> w536
                          frame False {
                            w623 = string[] []
                          }
                          frame True {
                            n165 = for {
                              N: 32 -> [_]
                              tunnel: w626 -> [w648]
                              tunnel: [w651] -> w632 mode=indexing
                              shift-right: [w650] -> w634
                              shift-left: w637 -> [w650]
                              tunnel: w627 -> [w647]
                              tunnel: [w646] -> w625 mode=indexing
                              i -> [w649]
                              n166 = Index Array(array=w647, index=w649) -> (element=w646:string)
                              n167 = Index Array(array=w648, index=w649) -> (element=w651:string)
                            }
                            n168 = for {
                              N: 32 -> [_]
                              tunnel: w636 -> [w645]
                              tunnel: [w644] -> w633 mode=indexing
                              shift-right: [w643] -> w635
                              shift-left: w637 -> [w643]
                              tunnel: w629 -> [w639]
                              tunnel: [w638] -> w628 mode=indexing
                              i -> [w642]
                              n169 = Add(x=32, y=w642) -> (x+y=w640:i32)
                              n170 = Index Array(array=w645, index=w640) -> (element=w644:string)
                              n171 = Index Array(array=w639, index=w640) -> (element=w638:string)
                            }
                          }
                        }
                        "RB Die Y\nBrd A" <- w536
                        "RB Die X\nBrd A" <- w535
                        "RB Die X\nBrd B" <- w533
                        "RB Die Y\nBrd B" <- w534
                        n172 = Merge Errors(w549, w548) -> (w550:errorcluster)
                        n173 = call "TLTSP_Measurement.vi"("error in (no error)"=w550, "Select Measurement"=w583, "VISA resource name"=w585) -> ("error out"=w579:errorcluster, "Output"=w575:string, "VISA resource name out"=w584:refnum<visa-resource-name>)  [unwired: 6 in]
                        n174 = call "Time Delay.vi"("Error In"=w579, "Delay(ms)"=u32 100) -> ("Error Out"=w578:errorcluster)  [unwired: 9 in]
                        n175 = call "TLTSP_Measurement.vi"("error in (no error)"=w578, "Select Measurement"=w582, "VISA resource name"=w584) -> ("error out"=w558:errorcluster, "Output"=w576:string, "VISA resource name out"=w580:refnum<visa-resource-name>)  [unwired: 6 in]
                        n176 = case shown="Error" w558 {
                          selector: w558 -> [w653 _]
                          tunnel: [w653 errorcluster {"status"=FALSE, "code"=0, "source"=""} ("error IO")] -> w557
                          tunnel: ["0" "2"] -> w556
                          frame No Error {
                          }
                          frame Error {
                          }
                        }
                        n177 = local write "Temp (C)"(w575) -> ()
                        n178 = for {
                          N: 32 -> [_]
                          shift-right: [w662] -> w596
                          shift-left: w557 -> [w662]
                          tunnel: w595 -> [w661]
                          tunnel: w594 -> [w659]
                          tunnel: w593 -> [w660]
                          tunnel: w592 -> [w658]
                          tunnel: [w661] -> w587 mode=indexing
                          tunnel: [w660] -> w589 mode=indexing
                          tunnel: [w659] -> w588 mode=indexing
                          tunnel: [w658] -> w590 mode=indexing
                          tunnel: [w657] -> w586 mode=indexing
                          tunnel: w575 -> [w657]
                          tunnel: [w656] -> w581 mode=indexing
                          tunnel: w576 -> [w656]
                        }
                        n179 = local write "RH(%)"(w576) -> ()
                        n180 = flat-sequence {
                          tunnel: w596 -> [w766]
                          tunnel: [w766] -> w610
                          tunnel: [w765] -> w611
                          tunnel: w609 -> [w764]
                          tunnel: [w763] -> w608
                          tunnel: w607 -> [w762]
                          tunnel: [w761] -> w606
                          tunnel: w605 -> [w760]
                          tunnel: [w760] -> w604
                          tunnel: w603 -> [w759]
                          tunnel: [w759] -> w602
                          tunnel: w601 -> [w758]
                          tunnel: [w758] -> w600
                          tunnel: w597 -> [w757]
                          tunnel: w568 -> [w756]
                          tunnel: w590 -> [w755]
                          tunnel: w590 -> [w754]
                          tunnel: w589 -> [w748]
                          tunnel: w589 -> [w753]
                          tunnel: w588 -> [w752]
                          tunnel: w588 -> [w751]
                          tunnel: w587 -> [w750]
                          tunnel: w587 -> [w749]
                          tunnel: w586 -> [w747]
                          tunnel: w586 -> [w746]
                          tunnel: w581 -> [w745]
                          tunnel: w581 -> [w744]
                          tunnel: w556 -> [w743]
                          tunnel: [w743] -> w555
                          tunnel: w536 -> [w741]
                          tunnel: w534 -> [w739]
                          tunnel: w535 -> [w742]
                          tunnel: w533 -> [w740]
                          frame #0 {
                            n181 = Build Array (concatenate)(w764, w756, w755, w748, w752, w750, w747, w745, w740, w739) -> (w763:string[][])
                            n182 = Build Array (concatenate)(w762, w757, w754, w753, w751, w749, w746, w744, w742, w741) -> (w761:string[][])
                            n183 = Select(t=Test_Sequences."Save Data" ("Test Sequences"), s=w766, f=Test_Sequences."Stress" ("Test Sequences")) -> (s? t:f=w765:T9)
                          }
                        }
                      }
                      frame "Stress" {
                        n184 = case shown="\"4.8us\"" w778 {
                          tunnel: w777 -> [w829 w844 w848 w861]
                          tunnel: [w827 w840 w847 w859] -> w776
                          tunnel: w775 -> [w828 w843 w845 w860]
                          tunnel: ["2.5" ("Beams") "0" ("Beams") "4.8" ("Beams") "5.26" ("Beams")] -> w774
                          frame "Default (2.5us)", Default {
                            n185 = for {
                              tunnel: w828 -> [w835]
                              shift-right: [w833] -> w827
                              shift-left: w829 -> [w836]
                              tunnel: string[] ["074101", "074E25"] -> [w830] mode=indexing
                              n186 = call "WSVCAP SHL Host TL RFFE Write - Multiple DUTs - Common Data.vi"("Data Out"=w830, "error in"=w836, "FPGA"=w835, "Log (T)"=FALSE) -> ("error out"=w832:errorcluster)  [unwired: 11 in]
                              n187 = call "Time Delay.vi"("Error In"=w832, "Delay(ms)"=u32 10) -> ("Error Out"=w833:errorcluster)  [unwired: 9 in]
                            }
                          }
                          frame "0us" {
                            n188 = call "WSVCAP SHL Host TL RFFE Write - Multiple DUTs - Common Data.vi"("Data Out"="074109", "error in"=w844, "FPGA"=w843, "Log (T)"=FALSE) -> ("error out"=w839:errorcluster)  [unwired: 11 in]
                            n189 = call "Time Delay.vi"("Error In"=w839, "Delay(ms)"=u32 10) -> ("Error Out"=w840:errorcluster)  [unwired: 9 in]
                          }
                          frame "4.8us" {
                            n190 = for {
                              tunnel: w845 -> [w855]
                              shift-right: [w854] -> w847
                              shift-left: w848 -> [w856]
                              tunnel: string[] ["074101", "074E2A"] -> [w850] mode=indexing
                              n191 = call "WSVCAP SHL Host TL RFFE Write - Multiple DUTs - Common Data.vi"("Data Out"=w850, "error in"=w856, "FPGA"=w855, "Log (T)"=FALSE) -> ("error out"=w853:errorcluster)  [unwired: 11 in]
                              n192 = call "Time Delay.vi"("Error In"=w853, "Delay(ms)"=u32 10) -> ("Error Out"=w854:errorcluster)  [unwired: 9 in]
                            }
                          }
                          frame "5.26us" {
                            n193 = for {
                              tunnel: w860 -> [w867]
                              shift-right: [w866] -> w859
                              shift-left: w861 -> [w868]
                              tunnel: string[] ["074101", "074E2B"] -> [w862] mode=indexing
                              n194 = call "WSVCAP SHL Host TL RFFE Write - Multiple DUTs - Common Data.vi"("Data Out"=w862, "error in"=w868, "FPGA"=w867, "Log (T)"=FALSE) -> ("error out"=w865:errorcluster)  [unwired: 11 in]
                              n195 = call "Time Delay.vi"("Error In"=w865, "Delay(ms)"=u32 10) -> ("Error Out"=w866:errorcluster)  [unwired: 9 in]
                            }
                          }
                        }
                        n196 = case shown="False" w822 {
                          tunnel: w776 -> [w901 w1105]
                          tunnel: [w903 w1102] -> w821
                          tunnel: w820 -> [w902 _]
                          tunnel: w819 -> [w899 _]
                          tunnel: [w898 FALSE ("Abort Stress")] -> w780
                          tunnel: w818 -> [w895 w1106]
                          tunnel: w817 -> [_ w1104]
                          tunnel: w811 -> [w897 _]
                          tunnel: w810 -> [w893 w1101]
                          tunnel: [w892 w1101] -> w809
                          tunnel: [w891 u64 1] -> w808
                          tunnel: [w896 "RPM"] -> w806
                          tunnel: w801 -> [w894 _]
                          tunnel: w800 -> [w890 _]
                          tunnel: [w889 "na" ("Cycle DC %")] -> w799
                          tunnel: w798 -> [w888 _]
                          tunnel: w775 -> [w887 _]
                          tunnel: w797 -> [w886 w1097]
                          tunnel: [w884 w1097] -> w796
                          tunnel: w789 -> [w883 w1096]
                          tunnel: [w882 w1096] -> w788
                          tunnel: w785 -> [w881 _]
                          tunnel: w786 -> [w880 _]
                          tunnel: w786 -> [w879 _]
                          tunnel: w775 -> [w878 _]
                          tunnel: w784 -> [w877 _]
                          tunnel: w783 -> [w876 _]
                          tunnel: w782 -> [w875 _]
                          tunnel: w775 -> [w872 _]
                          tunnel: w774 -> [w871 _]
                          tunnel: [w869 "na" ("Beams")] -> w773
                          frame False {
                            # "Stress"
                            n197 = case shown="True" w899 {
                              tunnel: w901 -> [w908 w917]
                              tunnel: [w907 w915] -> w900
                              tunnel: w886 -> [w909 w920]
                              tunnel: [w909 w920] -> w885
                              tunnel: w875 -> [w906 w919]
                              tunnel: [w906 w919] -> w874
                              tunnel: [w905 "n/a" ("Beams")] -> w873
                              tunnel: w872 -> [_ w916]
                              tunnel: w871 -> [w904 w910]
                              tunnel: [w904 w910] -> w870
                              frame False {
                                # "Beams"
                                n198 = call "WS1021 Stress Beams.vi"("error in (no error)"=w908, "Cycling Bit"=w906) -> ("error out"=w907:errorcluster, "Beams"=w905:string)  [unwired: 7 in, 1 out]
                              }
                              frame True {
                                # "OTP"
                                n199 = call "WSVCAP SHL Host TL RFFE Write - Multiple DUTs - Common Data.vi"("Data Out"="074100", "error in"=w917, "FPGA"=w916, "Log (T)"=FALSE) -> ("error out"=w913:errorcluster)  [unwired: 11 in]
                                n200 = call "Time Delay.vi"("Error In"=w913, "Delay(ms)"=u32 10) -> ("Error Out"=w915:errorcluster)  [unwired: 9 in]
                              }
                            }
                            n201 = case shown="True" w902 {
                              tunnel: w900 -> [w953 w1046]
                              tunnel: [w946 w1032] -> w903
                              tunnel: [w957 w1049] -> w898
                              tunnel: w897 -> [w951 _]
                              tunnel: [w954 w1018] -> w896
                              tunnel: w895 -> [w932 w1045]
                              tunnel: w894 -> [w952 w1043]
                              tunnel: w893 -> [w943 w1048]
                              tunnel: [w940 w1047] -> w892
                              tunnel: [w944 w1021] -> w891
                              tunnel: w890 -> [_ w1044]
                              tunnel: [w939 "Cycle DC %"] -> w889
                              tunnel: w888 -> [w938 w1042]
                              tunnel: w887 -> [w933 w1028]
                              tunnel: w885 -> [w931 w1039]
                              tunnel: [w928 w1039] -> w884
                              tunnel: w883 -> [w927 w1038]
                              tunnel: [w924 w1038] -> w882
                              tunnel: w881 -> [_ w1036]
                              tunnel: w880 -> [_ w1035]
                              tunnel: w879 -> [_ w1031]
                              tunnel: w878 -> [_ w1030]
                              tunnel: w877 -> [_ w1029]
                              tunnel: w876 -> [_ w1019]
                              tunnel: w874 -> [_ w1020]
                              tunnel: w873 -> [_ w1018]
                              tunnel: w870 -> [_ w1016]
                              tunnel: [w921 w1016] -> w869
                              frame False {
                                # "HD"
                                n202 = case shown="15, Default" w932 {
                                tunnel: w953 -> [w959 w961]
                                tunnel: [w959 w961] -> w949
                                tunnel: w952 -> [_ w960]
                                tunnel: [w958 w960] -> w923
                                tunnel: w951 -> [w958 _]
                                frame 15, Default {
                                }
                                frame 0..14 {
                                }
                                }
                                n203 = Format Into String(format string="%s", w938) -> (resulting string=w936:string)  [unwired: 2 in, 1 out]
                                n204 = Concatenate Strings(w936, "_Hold Down..." ("string")) -> (w934:string)
                                n205 = local write "Status"(w934) -> ()
                                n206 = flat-sequence {
                                tunnel: w923 -> [w985]
                                tunnel: [w981] -> w955
                                tunnel: "HD Cmd" -> [w978]
                                tunnel: w949 -> [w979]
                                tunnel: [w966] -> w948
                                tunnel: w943 -> [w980]
                                tunnel: [w980] -> w942
                                tunnel: w933 -> [w967]
                                tunnel: w932 -> [w974]
                                tunnel: w931 -> [w973]
                                tunnel: [w972] -> w930
                                tunnel: w927 -> [w970]
                                tunnel: [w970] -> w926
                                tunnel: w923 -> [w969]
                                tunnel: [w969] -> w922
                                tunnel: [w999] -> w956
                                tunnel: w955 -> [w997]
                                tunnel: w948 -> [w995]
                                tunnel: [w998] -> w947
                                tunnel: [w990] -> w945
                                tunnel: w942 -> [w996]
                                tunnel: [w996] -> w941
                                tunnel: w930 -> [w991]
                                tunnel: [w991] -> w929
                                tunnel: w926 -> [w993]
                                tunnel: [w992] -> w925
                                tunnel: w922 -> [w990]
                                tunnel: [w1015] -> w957
                                tunnel: w956 -> [w1015]
                                tunnel: ["HD Beams"] -> w954
                                tunnel: w947 -> [w1009]
                                tunnel: [w1008] -> w946
                                tunnel: w945 -> [w1014]
                                tunnel: [w1014] -> w944
                                tunnel: w941 -> [w1013]
                                tunnel: [w1013] -> w940
                                tunnel: ["100"] -> w939
                                tunnel: w929 -> [w1010]
                                tunnel: [w1010] -> w928
                                tunnel: w925 -> [w1007]
                                tunnel: [w1006] -> w924
                                tunnel: ["na"] -> w921
                                frame #0 {
                                n207 = call "WSVCAP SHL Host TL RFFE Write - Multiple DUTs - Common Data.vi"("Data Out"=w978, "error in"=w979, "FPGA"=w967, "Log (T)"=FALSE) -> ("error out"=w976:errorcluster)  [unwired: 11 in]
                                n208 = call "Time Delay.vi"("Error In"=w976, "Delay(ms)"=u32 10) -> ("Error Out"=w971:errorcluster)  [unwired: 9 in]
                                n209 = case shown="1, Default" w974 {
                                tunnel: w973 -> [_ w989]
                                tunnel: [0.0 ("DCV (V)") w989] -> w972
                                tunnel: w971 -> [w987 w988]
                                tunnel: [w987 w988] -> w968
                                frame 0 {
                                }
                                frame 1, Default {
                                }
                                }
                                n210 = Multiply(x=w985, y=u64 1000) -> (x*y=w983:u64)
                                n211 = Multiply(x=w983, y=u64 60) -> (x*y=w981:u64)
                                n212 = call "WS1021 Multi DUT Verify Beam RB.vi"("FPGA"=w967, "Error In"=w968, "Register RB"=string[] ["0762", "0763"]) -> ("Error Out"=w966:errorcluster, "Board B"=w963:string[][], "Board A"=w964:string[][])  [unwired: 6 in]
                                n213 = Build Array (concatenate)(w964, w963) -> (→"RB for HD Stress":string[][])
                                }
                                frame #1 {
                                n214 = call "Ke2400 Configure Output.vi"("error in (no error)"=w995, "Output Level (0)"=w991, "VISA resource name"=w993) -> ("error out"=w994:errorcluster, "VISA resource name out"=w992:refnum<visa-resource-name>)  [unwired: 7 in]
                                n215 = event shown="[0] Timeout" {
                                selector: _ -> [_ _]
                                dyn-events: _ -> [_ _]
                                timeout: w997 -> [_ _]
                                tunnel: ["Abort Stress" TRUE ("Abort Stress")] -> w999
                                tunnel: w994 -> [w1001 w1003]
                                tunnel: [w1001 w1003] -> w998
                                event Timeout {
                                n216 = event-data() -> ()  [unwired: 1 in, 2 out]
                                }
                                event "Abort Stress": Value Change {
                                n217 = event-data() -> ()  [unwired: 1 in, 2 out]
                                }
                                }
                                }
                                frame #2 {
                                n218 = call "Ke2400 Configure Output.vi"("error in (no error)"=w1009, "Output Level (0)"=0.0, "VISA resource name"=w1007) -> ("error out"=w1008:errorcluster, "VISA resource name out"=w1006:refnum<visa-resource-name>)  [unwired: 7 in]
                                }
                                }
                              }
                              frame True {
                                # "Cycling"
                                n219 = Format Into String(format string="%s", w1042) -> (resulting string=w1040:string)  [unwired: 2 in, 1 out]
                                n220 = case shown="8, Default" w1045 {
                                tunnel: w1046 -> [w1051 w1053]
                                tunnel: [w1051 w1053] -> w1037
                                tunnel: w1044 -> [_ w1052]
                                tunnel: [w1050 w1052] -> w1023
                                tunnel: w1043 -> [w1050 _]
                                frame 0..7 {
                                }
                                frame 8, Default {
                                }
                                }
                                n221 = Array Max & Min(array=w1019) -> (max value=w1027:dbl)  [unwired: 3 out]
                                n222 = call "WSVCAP SHL Host TL RFFE Configure.vi"("RFFE Slave Address"=w1035, "Clock Rate (Hz)"=w1036, "error in"=w1037, "FPGA"=w1028) -> ("error out"=w1034:errorcluster)  [unwired: 10 in, 1 out]
                                n223 = Multiply(x=w1023, y=u64 1000) -> (x*y=w1021:u64)
                                n224 = Divide(x=1.0, y=w1027) -> (x/y=w1025:dbl)
                                n225 = To Unsigned Quad Integer(1:w1025) -> (0:w1024:u64)
                                n226 = while {
                                tunnel: w1034 -> [w1068]
                                tunnel: [w1074] -> w1049
                                tunnel: [w1058] -> w1033
                                tunnel: w1048 -> [w1073]
                                tunnel: [w1073] -> w1047
                                tunnel: w1040 -> [w1071]
                                tunnel: w1020 -> [w1067]
                                tunnel: w1019 -> [w1066]
                                tunnel: w1028 -> [w1054]
                                tunnel: w1024 -> [w1061]
                                tunnel: w1021 -> [w1063]
                                i -> [w1069]
                                stop <- w1075 stop-if-true
                                n227 = case shown="0" w1069 {
                                tunnel: w1068 -> [w1091 w1093]
                                tunnel: w1067 -> [w1088 _]
                                tunnel: w1066 -> [w1087 _]
                                tunnel: w1054 -> [w1090 _]
                                tunnel: [w1092 w1093] -> w1057
                                frame 0 {
                                n228 = call "WSVCAP SHL Host TL RFFE Write Cycle - Multiple DUTs - Common Data.vi"("Data Out (Cycle Commands)"=w1088, "Post Command Delay"=w1087, "error in"=w1091, "FPGA"=w1090, "Log (T)"=FALSE) -> ("error out"=w1092:errorcluster)  [unwired: 10 in]
                                }
                                frame 1, Default {
                                }
                                }
                                n229 = call "WSVCAP SHL Host TL SPI_RFFE Query Cycle Count.vi"("error in"=w1057, "FPGA"=w1054) -> ("Cycle Count"=w1055:u64, "error out"=w1056:errorcluster)  [unwired: 12 in]
                                "Cycle Count" <- w1055
                                n230 = Concatenate Strings(w1071, "_Cycling..." ("string")) -> (w1072:string)
                                n231 = local write "Status"(w1072) -> ()
                                n232 = Greater Or Equal?(x=w1055, y=w1063) -> (x >= y?=w1065:bool)
                                n233 = Subtract(x=w1063, y=w1055) -> (x-y=w1062:u64)
                                n234 = case shown="False" w1065 {
                                tunnel: w1056 -> [w1080 w1084]
                                tunnel: w1054 -> [_ w1083]
                                tunnel: [FALSE TRUE] -> w1064
                                tunnel: [w1080 w1085] -> w1059
                                frame False {
                                }
                                frame True {
                                n235 = call "WSVCAP SHL Host TL RFFE Stop Write Cycle.vi"("error in"=w1084, "FPGA"=w1083, "Log (T)"=FALSE) -> ("error out"=w1085:errorcluster)  [unwired: 12 in]
                                }
                                }
                                n236 = Greater?(x=w1062, y=w1061) -> (0:w1060:bool)
                                n237 = local read "Abort Stress"() -> (w1074:bool)
                                n238 = case shown="True" w1060 {
                                tunnel: w1059 -> [w1076 w1079]
                                tunnel: [w1076 w1078] -> w1058
                                frame False {
                                }
                                frame True {
                                n239 = call "MISC Wait with Data Flow.vi"("Error In (no error)"=w1079, "Wait Time (500ms)"=u32 50) -> ("Error Out"=w1078:errorcluster)  [unwired: 7 in, 2 out]
                                }
                                }
                                n240 = Or(x=w1074, y=w1064) -> (x .or. y?=w1075:bool)
                                }
                                n241 = call "WSVCAP SHL Host TL RFFE Configure.vi"("RFFE Slave Address"=w1031, "Clock Rate (Hz)"=w1029, "error in"=w1033, "FPGA"=w1030) -> ("error out"=w1032:errorcluster)  [unwired: 10 in, 1 out]
                                "Verify Bits to Cycle" <- w1020
                                "Verify DC Speed" <- w1019
                              }
                            }
                          }
                          frame True {
                            # "Verify Socket"
                            n242 = To Unsigned Long Integer(number=w1104) -> (unsigned 32bit integer=w1103:u32)
                            n243 = case shown="1, Default" w1106 {
                              tunnel: w1105 -> [w1108 w1113]
                              tunnel: [w1108 w1112] -> w1102
                              tunnel: w1103 -> [_ w1111]
                              frame 0 {
                              }
                              frame 1, Default {
                                n244 = Multiply(x=w1111, y=u32 1000) -> (x*y=w1110:u32)
                                n245 = call "Time Delay.vi"("Error In"=w1113, "Delay(ms)"=w1110) -> ("Error Out"=w1112:errorcluster)  [unwired: 9 in]
                              }
                            }
                            n246 = local write "Status"("RPM to Verify Socket..." ("Status")) -> ()
                          }
                        }
                        n247 = flat-sequence {
                          tunnel: w821 -> [w1118]
                          tunnel: [w1132] -> w823
                          tunnel: [Test_Sequences."I_Measure" ("Test Sequences")] -> w824
                          tunnel: w813 -> [w1128]
                          tunnel: w812 -> [w1126]
                          tunnel: w809 -> [w1134]
                          tunnel: w808 -> [w1133]
                          tunnel: [w1127] -> w807
                          tunnel: w806 -> [w1129]
                          tunnel: [w1128] -> w805
                          tunnel: [w1125] -> w791
                          tunnel: [w1124] -> w772
                          tunnel: [w1126] -> w802
                          tunnel: [w1125] -> w794
                          tunnel: [w1124] -> w771
                          tunnel: w799 -> [w1123]
                          tunnel: [w1122] -> w795
                          tunnel: [w1122] -> w792
                          tunnel: w796 -> [w1121]
                          tunnel: [w1120] -> w793
                          tunnel: [w1120] -> w790
                          tunnel: w788 -> [w1119]
                          tunnel: [w1119] -> w787
                          tunnel: w773 -> [w1115]
                          tunnel: [w1114] -> w770
                          tunnel: [w1114] -> w769
                          frame #0 {
                            n248 = call "Time Delay.vi"("Error In"=w1118, "Delay(ms)"=u32 500) -> ("Error Out"=w1117:errorcluster)  [unwired: 9 in]
                            n249 = Add(x=w1134, y=w1133) -> (x+y=w1127:u64)
                            "TTF Completed" <- w1127
                            n250 = for {
                              N: 32 -> [_]
                              shift-right: [w1144] -> w1132
                              shift-left: w1117 -> [w1144]
                              tunnel: w1127 -> [w1143]
                              tunnel: [w1141] -> w1124 mode=indexing
                              tunnel: w1129 -> [w1140]
                              tunnel: [w1140] -> w1125 mode=indexing
                              tunnel: [w1139] -> w1122 mode=indexing
                              tunnel: w1123 -> [w1139]
                              tunnel: w1121 -> [w1138]
                              tunnel: [w1137] -> w1120 mode=indexing
                              tunnel: w1115 -> [w1135]
                              tunnel: [w1135] -> w1114 mode=indexing
                              n251 = Number To Fractional String(number=w1138, precision (6)=i16 2) -> (F-format string=w1137:string)  [unwired: 2 in]
                              n252 = Number To Fractional String(number=w1143, precision (6)=i16 2) -> (F-format string=w1141:string)  [unwired: 2 in]
                            }
                            "Stress DC(%)" <- w1123
                          }
                        }
                        n253 = Build Array (concatenate)(w805, w790, w791, w792, w769, w772) -> (w804:string[][])
                        n254 = Build Array (concatenate)(w802, w793, w794, w795, w770, w771) -> (w803:string[][])
                      }
                      frame "I_Measure" {
                        w1164 = FALSE ("true")
                        n255 = stacked-sequence {
                          seq-local: [w1225 _ _] -> [_ w1258 _]
                          seq-local: [w1214 _ _] -> [_ w1241 _]
                          seq-local: [_ w1251 _] -> [_ _ w1279]
                          seq-local: [_ w1256 _] -> [_ _ w1282]
                          tunnel: w1181 -> [w1223 _ _]
                          tunnel: u32 100 ("Delay(ms)") -> [w1228 w1254 w1283]
                          tunnel: w1179 -> [w1226 _ _]
                          tunnel: [w1224 _ _] -> w1171
                          tunnel: [_ w1257 _] -> w1170
                          tunnel: [_ _ w1281] -> w1178
                          tunnel: [_ _ w1275] -> w1167
                          tunnel: [_ _ w1280] -> w1169
                          tunnel: w1172 -> [w1219 w1238 w1274]
                          tunnel: [_ _ w1270] -> w1159
                          tunnel: [_ _ w1269] -> w1157
                          tunnel: [_ w1246 _] -> w1148
                          tunnel: [_ w1245 _] -> w1147
                          tunnel: [w1212 _ _] -> w1150
                          tunnel: [w1211 _ _] -> w1149
                          tunnel: [_ w1230 _] -> w1145
                          tunnel: [_ w1229 _] -> w1146
                          frame #0 {
                            # "IDD Stdby"
                            n256 = call "WSVCAP SHL Host TL RFFE Write - Multiple DUTs - Common Data.vi"("Data Out"="074000", "error in"=w1223, "FPGA"=w1219, "Log (T)"=FALSE) -> ("error out"=w1222:errorcluster)  [unwired: 11 in]
                            n257 = call "Time Delay.vi"("Error In"=w1222, "Delay(ms)"=w1228) -> ("Error Out"=w1227:errorcluster)  [unwired: 9 in]
                            n258 = call "Ke2000 Single Reading.vi"("error in (no error)"=w1227, "VISA resource name"=w1226) -> ("error out"=w1210:errorcluster, "VISA resource name out"=w1225:refnum<visa-resource-name>, "uA"=w1224:string)  [unwired: 5 in, 2 out]
                            n259 = call "Time Delay.vi"("Error In"=w1210, "Delay(ms)"=u32 10) -> ("Error Out"=w1209:errorcluster)  [unwired: 9 in]
                            n260 = call "WS1021 ADI Read 64 DUT.vi"("FPGA"=w1219, "Error In"=w1209) -> ("Error Out"=w1215:errorcluster, "AD7747 Values"=w1218:string[][])  [unwired: 8 in]
                            n261 = Index Array(array=w1218, index (col)=2 ("disabled index (col)")) -> (element=w1212:string[])  [unwired: 1 in]
                            n262 = Index Array(array=w1218, index (col)=5 ("disabled index (col)")) -> (element=w1211:string[])  [unwired: 1 in]
                            n263 = call "Time Delay.vi"("Error In"=w1215, "Delay(ms)"=u32 10) -> ("Error Out"=w1214:errorcluster)  [unwired: 9 in]
                          }
                          frame #1 {
                            # "IDD ALL ON"
                            n264 = call "WSVCAP SHL Host TL RFFE Write - Multiple DUTs - Common Data.vi"("Data Out"="074080", "error in"=w1241, "FPGA"=w1238, "Log (T)"=FALSE) -> ("error out"=w1236:errorcluster)  [unwired: 11 in]
                            n265 = call "Time Delay.vi"("Error In"=w1236, "Delay(ms)"=u32 10) -> ("Error Out"=w1237:errorcluster)  [unwired: 9 in]
                            n266 = call "WS1021 ADI Read 64 DUT.vi"("FPGA"=w1238, "Error In"=w1237) -> ("Error Out"=w1239:errorcluster, "AD7747 Values"=w1231:string[][])  [unwired: 8 in]
                            n267 = for {
                              tunnel: w1238 -> [w1263]
                              shift-right: [w1260] -> w1253
                              shift-left: w1239 -> [w1264]
                              tunnel: string[] ["074101", "0701027F7F"] -> [w1262] mode=indexing
                              tunnel: w1254 -> [w1259]
                              n268 = call "WSVCAP SHL Host TL RFFE Write - Multiple DUTs - Common Data.vi"("Data Out"=w1262, "error in"=w1264, "FPGA"=w1263, "Log (T)"=FALSE) -> ("error out"=w1261:errorcluster)  [unwired: 11 in]
                              n269 = call "Time Delay.vi"("Error In"=w1261, "Delay(ms)"=w1259) -> ("Error Out"=w1260:errorcluster)  [unwired: 9 in]
                            }
                            n270 = Index Array(array=w1231, index (col)=2 ("disabled index (col)")) -> (element=w1229:string[])  [unwired: 1 in]
                            n271 = Index Array(array=w1231, index (col)=5 ("disabled index (col)")) -> (element=w1230:string[])  [unwired: 1 in]
                            n272 = call "Ke2000 Single Reading.vi"("error in (no error)"=w1253, "VISA resource name"=w1258) -> ("error out"=w1243:errorcluster, "VISA resource name out"=w1256:refnum<visa-resource-name>, "uA"=w1257:string)  [unwired: 5 in, 2 out]
                            n273 = call "Time Delay.vi"("Error In"=w1243, "Delay(ms)"=u32 10) -> ("Error Out"=w1244:errorcluster)  [unwired: 9 in]
                            n274 = call "WS1021 ADI Read 64 DUT.vi"("FPGA"=w1238, "Error In"=w1244) -> ("Error Out"=w1252:errorcluster, "AD7747 Values"=w1248:string[][])  [unwired: 8 in]
                            n275 = call "Time Delay.vi"("Error In"=w1252, "Delay(ms)"=u32 10) -> ("Error Out"=w1251:errorcluster)  [unwired: 9 in]
                            n276 = Index Array(array=w1248, index (col)=2 ("disabled index (col)")) -> (element=w1246:string[])  [unwired: 1 in]
                            n277 = Index Array(array=w1248, index (col)=5 ("disabled index (col)")) -> (element=w1245:string[])  [unwired: 1 in]
                          }
                          frame #2 {
                            # "IDD ALL OFF"
                            n278 = call "WSVCAP SHL Host TL RFFE Write - Multiple DUTs - Common Data.vi"("Data Out"="0701020000", "error in"=w1279, "FPGA"=w1274, "Log (T)"=FALSE) -> ("error out"=w1278:errorcluster)  [unwired: 11 in]
                            n279 = call "Time Delay.vi"("Error In"=w1278, "Delay(ms)"=w1283) -> ("Error Out"=w1284:errorcluster)  [unwired: 9 in]
                            n280 = call "Ke2000 Single Reading.vi"("error in (no error)"=w1284, "VISA resource name"=w1282) -> ("error out"=w1268:errorcluster, "VISA resource name out"=w1281:refnum<visa-resource-name>, "uA"=w1280:string)  [unwired: 5 in, 2 out]
                            n281 = call "Time Delay.vi"("Error In"=w1268, "Delay(ms)"=u32 10) -> ("Error Out"=w1267:errorcluster)  [unwired: 9 in]
                            n282 = call "WS1021 ADI Read 64 DUT.vi"("FPGA"=w1274, "Error In"=w1267) -> ("Error Out"=w1275:errorcluster, "AD7747 Values"=w1272:string[][])  [unwired: 8 in]
                            n283 = Index Array(array=w1272, index (col)=5 ("disabled index (col)")) -> (element=w1270:string[])  [unwired: 1 in]
                            n284 = Index Array(array=w1272, index (col)=2 ("disabled index (col)")) -> (element=w1269:string[])  [unwired: 1 in]
                          }
                        }
                        n285 = local write "Status"("Measure IDD..." ("Status")) -> ()
                        n286 = Build Array(w1171, w1170, w1169) -> (→"IDD Measurement(uA)":string[])
                        n287 = for {
                          N: 32 -> [_]
                          tunnel: w1171 -> [w1207]
                          tunnel: [w1207] -> w1176 mode=indexing
                          tunnel: w1170 -> [w1206]
                          tunnel: [w1206] -> w1175 mode=indexing
                          tunnel: w1169 -> [w1205]
                          tunnel: [w1205] -> w1174 mode=indexing
                          shift-right: [w1204] -> w1156
                          shift-left: w1167 -> [w1204]
                        }
                        n288 = case shown="True" w1160 {
                          tunnel: w1159 -> [_ w1199]
                          tunnel: [string[] [] ("AD7747 Values") w1199] -> w1151
                          tunnel: w1156 -> [w1196 w1198]
                          tunnel: [w1196 w1198] -> w1154
                          frame False {
                          }
                          frame True {
                          }
                        }
                        "Cmin BrdB" <- w1151
                        n289 = case shown="True" w1158 {
                          tunnel: w1157 -> [_ w1195]
                          tunnel: [string[] [] ("AD7747 Values") w1195] -> w1152
                          tunnel: w1156 -> [w1193 w1194]
                          tunnel: [w1193 w1194] -> w1153
                          frame False {
                          }
                          frame True {
                          }
                        }
                        "Cmin BrdA" <- w1152
                        n290 = Fract/Exp String To Number(string=w1152) -> (number=→"CMin BrdA (fF)":dbl[])  [unwired: 3 in, 1 out]
                        n291 = Fract/Exp String To Number(string=w1151) -> (number=→"CMin BrdB (fF)":dbl[])  [unwired: 3 in, 1 out]
                        n292 = Merge Errors(w1154, w1153) -> (w1155:errorcluster)
                        n293 = case shown="Error" w1155 {
                          selector: w1155 -> [w1200 _]
                          tunnel: ["0" "3"] -> w1161
                          tunnel: [w1200 errorcluster {"status"=FALSE, "code"=0, "source"=""} ("Error Out")] -> w1162
                          frame No Error {
                          }
                          frame Error {
                          }
                        }
                        n294 = flat-sequence {
                          tunnel: w1162 -> [w1305]
                          tunnel: [w1305] -> w1190
                          tunnel: [w1304] -> w1191
                          tunnel: w1188 -> [w1303]
                          tunnel: [w1302] -> w1187
                          tunnel: [w1301] -> w1186
                          tunnel: w1185 -> [w1300]
                          tunnel: w1176 -> [w1299]
                          tunnel: w1176 -> [w1298]
                          tunnel: w1175 -> [w1286]
                          tunnel: w1175 -> [w1292]
                          tunnel: w1174 -> [w1288]
                          tunnel: w1174 -> [w1294]
                          tunnel: w1159 -> [w1289]
                          tunnel: w1157 -> [w1295]
                          tunnel: w1161 -> [w1297]
                          tunnel: [w1297] -> w1163
                          tunnel: w1150 -> [w1291]
                          tunnel: w1149 -> [w1296]
                          tunnel: w1148 -> [w1293]
                          tunnel: w1147 -> [w1287]
                          tunnel: w1146 -> [w1290]
                          tunnel: w1145 -> [w1285]
                          frame #0 {
                            n295 = Build Array (concatenate)(w1303, w1299, w1296, w1285, w1286, w1287, w1288, w1289) -> (w1302:string[][])
                            n296 = Build Array (concatenate)(w1300, w1298, w1291, w1290, w1292, w1293, w1294, w1295) -> (w1301:string[][])
                            n297 = Select(t=Test_Sequences."Save Data" ("Test Sequences"), s=w1305, f=Test_Sequences."Cap_Measure" ("Test Sequences")) -> (s? t:f=w1304:T9)
                          }
                        }
                      }
                      frame "Cap_Measure" {
                        w1311 = FALSE ("true")
                        n298 = Build Array (concatenate)(w1344, w1343) -> (w1342:string[])
                        n299 = Build Array (concatenate)(w1347, w1346) -> (w1345:string[])
                        n300 = call "WS1021 CP Setting.vi"("Manual Setting"=w1313, "FPGA"=w1314, "Error In"=w1318) -> ("Error Out"=w1316:errorcluster)  [unwired: 7 in, 1 out]
                        n301 = call "Time Delay.vi"("Error In"=w1316, "Delay(ms)"=u32 50) -> ("Error Out"=w1317:errorcluster)  [unwired: 9 in]
                        n302 = for {
                          shift-right: [w1386] -> w1337
                          shift-left: w1317 -> [w1397]
                          tunnel: w1345 -> [w1396] mode=indexing
                          tunnel: w1342 -> [w1401] mode=indexing
                          tunnel: [w1389] -> w1333 mode=indexing
                          tunnel: [w1398] -> w1335 mode=indexing
                          tunnel: w1312 -> [w1395]
                          tunnel: w1312 -> [w1388]
                          n303 = call "WSVCAP SHL Host TL RFFE Write - Multiple DUTs - Common Data.vi"("Data Out"=w1396, "error in"=w1397, "FPGA"=w1395, "Log (T)"=FALSE) -> ("error out"=w1393:errorcluster)  [unwired: 11 in]
                          n304 = Concatenate Strings("Measure " ("string"), w1401) -> (w1399:string)
                          n305 = local write "Status"(w1399) -> ()
                          n306 = call "WS1021 ADI Read 64 DUT.vi"("FPGA"=w1388, "Error In"=w1393) -> ("Error Out"=w1387:errorcluster, "AD7747 Values"=w1390:string[][])  [unwired: 8 in]
                          n307 = Index Array(array=w1390, index (col)=5 ("disabled index (col)")) -> (element=w1398:string[])  [unwired: 1 in]
                          n308 = Index Array(array=w1390, index (col)=2 ("disabled index (col)")) -> (element=w1389:string[])  [unwired: 1 in]
                          n309 = call "Time Delay.vi"("Error In"=w1387, "Delay(ms)"=u32 10) -> ("Error Out"=w1386:errorcluster)  [unwired: 9 in]
                        }
                        n310 = case shown="True" w1309 {
                          tunnel: w1337 -> [w1367 w1376]
                          tunnel: w1335 -> [_ w1375]
                          tunnel: [string[][] [] w1374] -> w1334
                          tunnel: [_ w1373] -> w1331
                          tunnel: [_ w1372] -> w1329
                          tunnel: [_ w1371] -> w1327
                          tunnel: [_ w1370] -> w1325
                          tunnel: [w1367 w1369] -> w1322
                          frame False {
                          }
                          frame True {
                            n311 = Transpose 2D Array(2D array=w1375) -> (transposed array=w1374:string[][])
                            n312 = local read "CMin BrdB (fF)"() -> (w1368:dbl[])
                            n313 = call "WS1021 Calc DCAP_RTZ_Percentage.vi"("Cmin(fF)"=w1368, "Error In"=w1376, "Input"=w1374) -> ("Error Out"=w1369:errorcluster, "% Total Delta C(fF)"=w1371:string[], "Total Delta C(fF)"=w1372:string[], "% Beam Delta C(fF)"=w1373:string[][], "Delta Cap(fF)"=w1370:string[][])  [unwired: 3 in, 1 out]
                          }
                        }
                        "Brd B_Beam Cap (fF)" <- w1334
                        n314 = case shown="True" w1308 {
                          tunnel: w1337 -> [w1356 w1365]
                          tunnel: w1333 -> [_ w1364]
                          tunnel: [string[][] [] w1363] -> w1332
                          tunnel: [_ w1362] -> w1330
                          tunnel: [_ w1361] -> w1328
                          tunnel: [_ w1360] -> w1326
                          tunnel: [_ w1359] -> w1324
                          tunnel: [w1356 w1358] -> w1320
                          frame False {
                          }
                          frame True {
                            n315 = Transpose 2D Array(2D array=w1364) -> (transposed array=w1363:string[][])
                            n316 = local read "CMin BrdA (fF)"() -> (w1357:dbl[])
                            n317 = call "WS1021 Calc DCAP_RTZ_Percentage.vi"("Cmin(fF)"=w1357, "Error In"=w1365, "Input"=w1363) -> ("Error Out"=w1358:errorcluster, "% Total Delta C(fF)"=w1360:string[], "Total Delta C(fF)"=w1361:string[], "% Beam Delta C(fF)"=w1362:string[][], "Delta Cap(fF)"=w1359:string[][])  [unwired: 3 in, 1 out]
                          }
                        }
                        "Brd A_Beam Cap (fF)" <- w1332
                        n318 = case shown="1, Default" w1323 {
                          tunnel: w1327 -> [w1380 w1382]
                          tunnel: w1326 -> [w1379 w1381]
                          tunnel: w1322 -> [w1378 w1384]
                          tunnel: [w1378 w1384] -> w1321
                          tunnel: w1320 -> [w1377 w1383]
                          tunnel: [w1377 w1383] -> w1319
                          frame 0 {
                            "T0_Brd A Delta C%" <- w1379
                            "T0_Brd B Delta C%" <- w1380
                          }
                          frame 1, Default {
                            "Brd B Delta C%" <- w1382
                            "Brd A Delta C%" <- w1381
                          }
                        }
                        n319 = Merge Errors(w1321, w1319) -> (w1336:errorcluster)
                        n320 = flat-sequence {
                          tunnel: w1336 -> [w1418]
                          tunnel: [w1418] -> w1353
                          tunnel: [w1417] -> w1354
                          tunnel: w1341 -> [w1413]
                          tunnel: [w1416] -> w1340
                          tunnel: w1339 -> [w1410]
                          tunnel: [w1415] -> w1338
                          tunnel: w1333 -> [w1409]
                          tunnel: w1335 -> [w1412]
                          tunnel: w1331 -> [w1414]
                          tunnel: w1330 -> [w1407]
                          tunnel: w1329 -> [w1406]
                          tunnel: w1328 -> [w1404]
                          tunnel: w1327 -> [w1405]
                          tunnel: w1326 -> [w1403]
                          tunnel: w1325 -> [w1411]
                          tunnel: w1324 -> [w1408]
                          tunnel: [""] -> w1310
                          frame #0 {
                            n321 = Build Array (concatenate)(w1413, w1412, w1411, w1414, w1406, w1405) -> (w1416:string[][])
                            n322 = Build Array (concatenate)(w1410, w1409, w1408, w1407, w1404, w1403) -> (w1415:string[][])
                            n323 = Select(t=Test_Sequences."Save Data" ("Test Sequences"), s=w1418, f=Test_Sequences."VPI" ("Test Sequences")) -> (s? t:f=w1417:T9)
                          }
                        }
                      }
                      frame "VPI" {
                        w1431 = FALSE ("true")
                        n324 = case shown="True" w1450 {
                          tunnel: w1454 -> [w1486 w1514]
                          tunnel: w1453 -> [w1489 w1516]
                          tunnel: w1452 -> [_ w1515]
                          tunnel: [w1490 w1501] -> w1443
                          tunnel: w1445 -> [_ w1513]
                          tunnel: w1444 -> [_ w1512]
                          tunnel: w1421 -> [_ w1509]
                          tunnel: [w1488 w1508] -> w1430
                          tunnel: [w1487 w1507] -> w1429
                          tunnel: [w1483 w1503] -> w1425
                          tunnel: w1422 -> [_ _]
                          frame False {
                            n325 = for {
                              N: 32 -> [_]
                              shift-right: [w1492] -> w1485
                              shift-left: w1486 -> [w1492]
                              tunnel: [""] -> w1483 mode=indexing
                            }
                            n326 = for {
                              tunnel: w1489 -> [w1496] mode=indexing
                              tunnel: [w1495] -> w1488 mode=indexing
                              shift-right: [w1497] -> w1490
                              shift-left: w1485 -> [w1498]
                              tunnel: [w1493] -> w1487 mode=indexing
                              n327 = for {
                                N: 32 -> [_]
                                shift-right: [w1500] -> w1497
                                shift-left: w1498 -> [w1500]
                                tunnel: w1496 -> [_]
                                tunnel: [w1499] -> w1495 mode=indexing
                                tunnel: [w1499] -> w1493 mode=indexing
                                w1499 = ""
                              }
                            }
                          }
                          frame True {
                            n328 = call "WS1021 CP Setting.vi"("Manual Setting"=w1512, "FPGA"=w1513, "Error In"=w1514) -> ("Error Out"=w1506:errorcluster, "CP Select"=w1504:string)  [unwired: 7 in]
                            n329 = for {
                              N: 32 -> [_]
                              shift-right: [w1518] -> w1505
                              shift-left: w1506 -> [w1518]
                              tunnel: w1504 -> [w1517]
                              tunnel: [w1517] -> w1503 mode=indexing
                            }
                            n330 = call "Time Delay.vi"("Error In"=w1505, "Delay(ms)"=u32 50) -> ("Error Out"=w1510:errorcluster)  [unwired: 9 in]
                            n331 = for {
                              shift-right: [w1521] -> w1501
                              shift-left: w1510 -> [w1529]
                              tunnel: w1516 -> [w1534] mode=indexing
                              tunnel: w1515 -> [w1527] mode=indexing
                              tunnel: w1509 -> [w1528]
                              tunnel: [w1523] -> w1508 mode=indexing
                              tunnel: [w1522] -> w1507 mode=indexing
                              n332 = call "WSVCAP SHL Host TL RFFE Write - Multiple DUTs - Common Data.vi"("Data Out"=w1527, "error in"=w1529, "FPGA"=w1528, "Log (T)"=FALSE) -> ("error out"=w1531:errorcluster)  [unwired: 11 in]
                              n333 = call "WS1021 ADI Read 64 DUT.vi"("FPGA"=w1528, "Error In"=w1531) -> ("Error Out"=w1520:errorcluster, "AD7747 Values"=w1526:string[][])  [unwired: 8 in]
                              n334 = Concatenate Strings("Measure VPI " ("string"), w1534) -> (w1532:string)
                              n335 = local write "Status"(w1532) -> ()
                              n336 = Index Array(array=w1526, index (col)=5 ("disabled index (col)")) -> (element=w1523:string[])  [unwired: 1 in]
                              n337 = Index Array(array=w1526, index (col)=2 ("disabled index (col)")) -> (element=w1522:string[])  [unwired: 1 in]
                              n338 = call "Time Delay.vi"("Error In"=w1520, "Delay(ms)"=u32 10) -> ("Error Out"=w1521:errorcluster)  [unwired: 9 in]
                            }
                          }
                        }
                        n339 = case shown="True" w1423 {
                          tunnel: w1443 -> [w1474 w1482]
                          tunnel: [w1474 w1481] -> w1441
                          tunnel: [_ w1480] -> w1439
                          tunnel: [_ w1479] -> w1438
                          tunnel: [_ w1478] -> w1437
                          tunnel: [string[] [] ("VPI % Delta C") w1477] -> w1436
                          tunnel: w1430 -> [_ w1476]
                          tunnel: [string[][] [] w1475] -> w1427
                          frame False {
                          }
                          frame True {
                            n340 = Transpose 2D Array(2D array=w1476) -> (transposed array=w1475:string[][])
                            n341 = call "WS1021 Multi DUT VPI DeltaC.vi"("Error In"=w1482, "VPI Input"=w1475) -> ("Error Out"=w1481:errorcluster, "VPI % Delta C"=w1477:string[], "VPI Total Delta C (fF)"=w1478:string[], "VPI Delta C R2 (fF)"=w1479:string[], "VPI Delta C R3 (fF)"=w1480:string[])  [unwired: 5 in]
                          }
                        }
                        "VPI Brd B Delta C%" <- w1436
                        "Brd B_VPI Cap (fF)" <- w1427
                        n342 = case shown="True" w1424 {
                          tunnel: w1443 -> [w1463 w1471]
                          tunnel: [w1463 w1470] -> w1440
                          tunnel: [_ w1469] -> w1435
                          tunnel: [_ w1468] -> w1434
                          tunnel: [_ w1467] -> w1433
                          tunnel: [string[] [] ("VPI % Delta C") w1466] -> w1432
                          tunnel: w1429 -> [_ w1465]
                          tunnel: [string[][] [] w1464] -> w1428
                          frame False {
                          }
                          frame True {
                            n343 = Transpose 2D Array(2D array=w1465) -> (transposed array=w1464:string[][])
                            n344 = call "WS1021 Multi DUT VPI DeltaC.vi"("Error In"=w1471, "VPI Input"=w1464) -> ("Error Out"=w1470:errorcluster, "VPI % Delta C"=w1466:string[], "VPI Total Delta C (fF)"=w1467:string[], "VPI Delta C R2 (fF)"=w1468:string[], "VPI Delta C R3 (fF)"=w1469:string[])  [unwired: 5 in]
                          }
                        }
                        "VPI Brd A Delta C%" <- w1432
                        "Brd A_VPI Cap (fF)" <- w1428
                        n345 = Merge Errors(w1441, w1440) -> (w1442:errorcluster)
                        n346 = flat-sequence {
                          tunnel: w1442 -> [w1553]
                          tunnel: [w1553] -> w1460
                          tunnel: [w1552] -> w1459
                          tunnel: [w1551] -> w1449
                          tunnel: w1448 -> [w1550]
                          tunnel: w1447 -> [w1549]
                          tunnel: [w1548] -> w1446
                          tunnel: w1430 -> [w1542]
                          tunnel: w1429 -> [w1536]
                          tunnel: w1439 -> [w1543]
                          tunnel: w1438 -> [w1544]
                          tunnel: w1437 -> [w1545]
                          tunnel: w1436 -> [w1546]
                          tunnel: w1435 -> [w1538]
                          tunnel: w1434 -> [w1539]
                          tunnel: w1433 -> [w1540]
                          tunnel: w1432 -> [w1541]
                          tunnel: [""] -> w1426
                          tunnel: w1425 -> [w1537]
                          tunnel: w1425 -> [w1535]
                          frame #0 {
                            n347 = Build Array (concatenate)(w1550, w1537, w1542, w1543, w1544, w1545, w1546) -> (w1551:string[][])
                            n348 = Build Array (concatenate)(w1549, w1535, w1536, w1538, w1539, w1540, w1541) -> (w1548:string[][])
                            n349 = Select(t=Test_Sequences."Save Data" ("Test Sequences"), s=w1553, f=Test_Sequences."Open State VCmin" ("Test Sequences")) -> (s? t:f=w1552:T9)
                          }
                        }
                      }
                      frame "Open State VCmin" {
                        w1564 = FALSE ("true")
                        n350 = case shown="True" w1593 {
                          tunnel: w1592 -> [w1634 w1655]
                          tunnel: w1591 -> [w1630 w1654]
                          tunnel: w1590 -> [w1632 w1653]
                          tunnel: [w1633 w1652] -> w1582
                          tunnel: [w1631 w1651] -> w1568
                          tunnel: [w1630 w1650] -> w1585
                          tunnel: [w1629 w1649] -> w1567
                          tunnel: [w1628 w1648] -> w1566
                          tunnel: w1565 -> [_ w1647]
                          frame False {
                            n351 = for {
                              shift-right: [w1640] -> w1633
                              shift-left: w1634 -> [w1641]
                              tunnel: w1632 -> [w1643] mode=indexing
                              tunnel: [w1637] -> w1631 mode=indexing
                              tunnel: [w1636] -> w1629 mode=indexing
                              tunnel: [w1635] -> w1628 mode=indexing
                              n352 = Number To Fractional String(number=w1643, precision (6)=i16 2) -> (F-format string=w1638:string)  [unwired: 2 in]
                              n353 = for {
                                N: 32 -> [_]
                                shift-right: [w1646] -> w1640
                                shift-left: w1641 -> [w1646]
                                tunnel: w1638 -> [w1645]
                                tunnel: [w1645] -> w1637 mode=indexing
                                tunnel: [w1644] -> w1636 mode=indexing
                                tunnel: [w1644] -> w1635 mode=indexing
                                w1644 = ""
                              }
                            }
                          }
                          frame True {
                            n354 = for {
                              tunnel: w1654 -> [w1681]
                              tunnel: w1653 -> [w1679] mode=indexing
                              tunnel: [w1667] -> w1651 mode=indexing
                              shift-right: [w1663] -> w1652
                              shift-left: w1655 -> [w1682]
                              tunnel: [w1666] -> w1650
                              tunnel: [w1660] -> w1649 mode=indexing
                              tunnel: [w1659] -> w1648 mode=indexing
                              tunnel: w1647 -> [w1656]
                              n355 = call "Ke2400 Configure Output.vi"("error in (no error)"=w1682, "Compliance  Level (0.1)"=0.1, "Output Level (0)"=w1679, "VISA resource name"=w1681) -> ("error out"=w1675:errorcluster, "VISA resource name out"=w1674:refnum<visa-resource-name>)  [unwired: 6 in]
                              n356 = Number To Fractional String(number=w1679, precision (6)=i16 2) -> (F-format string=w1669:string)  [unwired: 2 in]
                              n357 = Concatenate Strings("Testing OS " ("string"), w1669) -> (w1676:string)
                              n358 = call "Ke2400 Enable.vi"("error in (no error)"=w1675, "ON/OFF"=TRUE, "VISA In"=w1674) -> ("error out"=w1672:errorcluster, "VISA Out"=w1666:refnum<visa-resource-name>)  [unwired: 7 in]
                              n359 = call "Time Delay.vi"("Error In"=w1672, "Delay(ms)"=u32 10) -> ("Error Out"=w1670:errorcluster)  [unwired: 9 in]
                              n360 = for {
                                N: 32 -> [_]
                                shift-right: [w1684] -> w1665
                                shift-left: w1670 -> [w1684]
                                tunnel: w1669 -> [w1683]
                                tunnel: [w1683] -> w1667 mode=indexing
                              }
                              n361 = local write "Status"(w1676) -> ()
                              n362 = call "WS1021 ADI Read 64 DUT.vi"("FPGA"=w1656, "Error In"=w1665) -> ("Error Out"=w1664:errorcluster, "AD7747 Values"=w1661:string[][])  [unwired: 8 in]
                              n363 = Index Array(array=w1661, index (col)=2 ("disabled index (col)")) -> (element=w1659:string[])  [unwired: 1 in]
                              n364 = Index Array(array=w1661, index (col)=5 ("disabled index (col)")) -> (element=w1660:string[])  [unwired: 1 in]
                              n365 = call "Time Delay.vi"("Error In"=w1664, "Delay(ms)"=u32 50) -> ("Error Out"=w1663:errorcluster)  [unwired: 9 in]
                            }
                          }
                        }
                        n366 = case shown="True" w1557 {
                          tunnel: w1582 -> [w1613 w1623]
                          tunnel: [w1613 w1622] -> w1580
                          tunnel: [_ w1621] -> w1578
                          tunnel: [_ w1620] -> w1577
                          tunnel: [_ w1619] -> w1576
                          tunnel: [w1612 w1618] -> w1571
                          tunnel: [w1612 w1617] -> w1570
                          tunnel: [w1612 w1616] -> w1569
                          tunnel: w1568 -> [_ w1615]
                          tunnel: w1567 -> [_ w1614]
                          frame False {
                            w1612 = string[][] [] ("VSA_V3")
                          }
                          frame True {
                            n367 = call "WS1021 VSA Convert Data.vi"("VSA_Cap(fF)"=w1614, "Voltage(V)"=w1615, "error in (no error)"=w1623) -> ("BT_VSA_V1"=w1621:string[][], "BT_VSA_V2"=w1620:string[][], "BT_VSA_V3"=w1619:string[][], "VSA_V3"=w1618:string[][], "VSA_V1"=w1616:string[][], "VSA_V2"=w1617:string[][], "error out"=w1622:errorcluster)  [unwired: 6 in]
                          }
                        }
                        "Brd B_OS_V1 (fF)" <- w1569
                        "Brd B_OS_V2 (fF)" <- w1570
                        "Brd B_OS_V3 (fF)" <- w1571
                        n368 = case shown="True" w1556 {
                          tunnel: w1582 -> [w1601 w1611]
                          tunnel: [w1601 w1610] -> w1579
                          tunnel: [_ w1609] -> w1575
                          tunnel: [_ w1608] -> w1574
                          tunnel: [_ w1607] -> w1573
                          tunnel: [w1600 w1606] -> w1572
                          tunnel: w1568 -> [_ w1605]
                          tunnel: w1566 -> [_ w1604]
                          tunnel: [w1600 w1603] -> w1563
                          tunnel: [w1600 w1602] -> w1562
                          frame False {
                            w1600 = string[][] [] ("VSA_V3")
                          }
                          frame True {
                            n369 = call "WS1021 VSA Convert Data.vi"("VSA_Cap(fF)"=w1604, "Voltage(V)"=w1605, "error in (no error)"=w1611) -> ("BT_VSA_V1"=w1609:string[][], "BT_VSA_V2"=w1608:string[][], "BT_VSA_V3"=w1607:string[][], "VSA_V3"=w1606:string[][], "VSA_V1"=w1603:string[][], "VSA_V2"=w1602:string[][], "error out"=w1610:errorcluster)  [unwired: 6 in]
                          }
                        }
                        "Brd A_OS_V2 (fF)" <- w1562
                        "Brd A_OS_V3 (fF)" <- w1572
                        "Brd A_OS_V1 (fF)" <- w1563
                        n370 = Merge Errors(w1580, w1579) -> (w1581:errorcluster)
                        n371 = call "Ke2400 Configure Output.vi"("error in (no error)"=w1581, "Output Level (0)"=0.0, "VISA resource name"=w1585) -> ("error out"=w1561:errorcluster, "VISA resource name out"=w1584:refnum<visa-resource-name>)  [unwired: 7 in]
                        n372 = case shown="Error" w1561 {
                          selector: w1561 -> [w1624 _]
                          tunnel: ["0" "4"] -> w1560
                          tunnel: [w1624 errorcluster {"status"=FALSE, "code"=0, "source"=""} ("error IO")] -> w1558
                          frame No Error {
                          }
                          frame Error {
                          }
                        }
                        n373 = flat-sequence {
                          tunnel: w1558 -> [w1697]
                          tunnel: [w1697] -> w1599
                          tunnel: [w1696] -> w1598
                          tunnel: w1589 -> [w1695]
                          tunnel: w1588 -> [w1694]
                          tunnel: [w1693] -> w1587
                          tunnel: [w1692] -> w1586
                          tunnel: w1578 -> [w1691]
                          tunnel: w1577 -> [w1690]
                          tunnel: w1576 -> [w1689]
                          tunnel: w1575 -> [w1688]
                          tunnel: w1574 -> [w1687]
                          tunnel: w1573 -> [w1686]
                          tunnel: w1560 -> [w1685]
                          tunnel: [w1685] -> w1559
                          frame #0 {
                            n374 = Build Array (concatenate)(w1695, w1691, w1690, w1689) -> (w1692:string[][])
                            n375 = Build Array (concatenate)(w1694, w1688, w1687, w1686) -> (w1693:string[][])
                            n376 = Select(t=Test_Sequences."Save Data" ("Test Sequences"), s=w1697, f=Test_Sequences."Close State VCmiin" ("Test Sequences")) -> (s? t:f=w1696:T9)
                          }
                        }
                      }
                      frame "Close State VCmiin" {
                        w1712 = FALSE ("true")
                        n377 = call "WS1021 CS Beam VCmin.vi"("Reg"=string[] ["43", "42", "43", "43", "43", "43", "43", "43", "42", "42", "42", "42", "42", "42", "999"], "Error In"=w1728, "Cmd Bit"=string[] ["40", "40", "20", "01", "02", "04", "08", "10", "01", "02", "04", "08", "10", "20", "999"], "Driver Name"=string[] ["FB1", "FB2", "FB3", "TB1", "TB2", "TB3", "TB4", "TB5", "TB6", "TB7", "TB8", "TB9", "TB10", "TB11", "All"]) -> ("Error Out"=w1727:errorcluster, "All Array"=w1700:bool[], "Beam Cmd OFF"=w1701:string[], "Beam Cmd"=w1725:string[], "CS_Driver Name"=w1726:string[])  [unwired: 3 in]
                        n378 = case shown="True" w1711 {
                          tunnel: w1727 -> [w1808 w1862]
                          tunnel: w1740 -> [w1809 w1868]
                          tunnel: w1739 -> [w1802 w1863]
                          tunnel: [w1807 w1849] -> w1721
                          tunnel: [w1809 w1867] -> w1737
                          tunnel: w1707 -> [_ w1866]
                          tunnel: [w1804 w1842] -> w1723
                          tunnel: [w1803 w1838] -> w1722
                          tunnel: w1726 -> [w1806 w1865]
                          tunnel: w1725 -> [_ w1864]
                          tunnel: [w1802 w1863] -> w1715
                          tunnel: w1709 -> [_ w1860]
                          tunnel: w1708 -> [_ w1859]
                          tunnel: w1705 -> [_ w1858]
                          tunnel: w1704 -> [_ w1857]
                          tunnel: w1701 -> [_ w1856]
                          tunnel: w1700 -> [_ w1834]
                          frame False {
                            w1805 = string[][] []
                            n379 = for {
                              shift-right: [w1814] -> w1807
                              shift-left: w1808 -> [w1823]
                              tunnel: w1802 -> [w1825] mode=indexing
                              tunnel: w1806 -> [w1820]
                              shift-right: [w1819] -> w1804
                              shift-left: w1805 -> [w1818]
                              shift-right: [w1817] -> w1803
                              shift-left: w1805 -> [w1816]
                              n380 = Number To Fractional String(number=w1825, precision (6)=i16 2) -> (F-format string=w1822:string)  [unwired: 2 in]
                              n381 = for {
                                N: 32 -> [_]
                                shift-right: [w1833] -> w1815
                                shift-left: w1823 -> [w1833]
                                tunnel: w1822 -> [w1832]
                                tunnel: [w1832] -> w1813 mode=indexing
                              }
                              n382 = for {
                                tunnel: w1820 -> [_] mode=indexing
                                shift-right: [w1827] -> w1814
                                shift-left: w1815 -> [w1828]
                                tunnel: [w1826] -> w1812 mode=indexing
                                n383 = for {
                                N: 32 -> [_]
                                tunnel: [""] -> w1826 mode=indexing
                                shift-right: [w1830] -> w1827
                                shift-left: w1828 -> [w1830]
                                }
                              }
                              n384 = Build Array (concatenate)(w1813, w1812) -> (w1810:string[][])
                              n385 = Build Array (concatenate)(w1813, w1812) -> (w1811:string[][])
                              n386 = Build Array (concatenate)(w1818, w1810) -> (w1819:string[][])
                              n387 = Build Array (concatenate)(w1816, w1811) -> (w1817:string[][])
                            }
                          }
                          frame True {
                            w1852 = string[][] []
                            n388 = call "WS1021 CP Setting.vi"("Manual Setting"=w1859, "FPGA"=w1860, "Error In"=w1862) -> ("Error Out"=w1861:errorcluster)  [unwired: 7 in, 1 out]
                            n389 = for {
                              tunnel: w1865 -> [w1901] mode=indexing
                              shift-right: [w1897] -> w1855
                              shift-left: w1861 -> [w1913]
                              tunnel: w1864 -> [w1912] mode=indexing
                              tunnel: w1866 -> [w1891]
                              tunnel: w1856 -> [w1911] mode=indexing
                              tunnel: w1863 -> [w1910]
                              tunnel: w1868 -> [w1903]
                              tunnel: [w1906] -> w1867
                              shift-right: [w1899] -> w1851
                              shift-left: w1852 -> [w1900]
                              shift-right: [w1893] -> w1850
                              shift-left: w1852 -> [w1892]
                              tunnel: w1834 -> [w1889] mode=indexing
                              w1896 = string[][] []
                              n390 = case shown="True" w1889 {
                                tunnel: w1913 -> [w1934 w1939]
                                tunnel: w1912 -> [_ w1938]
                                tunnel: w1891 -> [w1931 w1936]
                                tunnel: [w1929 w1935] -> w1890
                                frame True {
                                n391 = call "WSVCAP SHL Host TL RFFE Write - Multiple DUTs - Common Data.vi"("Data Out"="07427F", "error in"=w1934, "FPGA"=w1931, "Log (T)"=FALSE) -> ("error out"=w1930:errorcluster)  [unwired: 11 in]
                                n392 = call "WSVCAP SHL Host TL RFFE Write - Multiple DUTs - Common Data.vi"("Data Out"="07437F", "error in"=w1930, "FPGA"=w1931, "Log (T)"=FALSE) -> ("error out"=w1929:errorcluster)  [unwired: 11 in]
                                }
                                frame False {
                                n393 = call "WSVCAP SHL Host TL RFFE Write - Multiple DUTs - Common Data.vi"("Data Out"=w1938, "error in"=w1939, "FPGA"=w1936, "Log (T)"=FALSE) -> ("error out"=w1935:errorcluster)  [unwired: 11 in]
                                }
                              }
                              n394 = call "Time Delay.vi"("Error In"=w1890, "Delay(ms)"=u32 25) -> ("Error Out"=w1905:errorcluster)  [unwired: 9 in]
                              n395 = for {
                                tunnel: w1891 -> [w1965]
                                tunnel: w1910 -> [w1956] mode=indexing
                                shift-right: [w1964] -> w1909
                                shift-left: w1905 -> [w1954]
                                tunnel: w1903 -> [w1962]
                                tunnel: [w1961] -> w1902
                                tunnel: w1901 -> [w1946]
                                shift-right: [w1948] -> w1898
                                shift-left: w1896 -> [w1949]
                                tunnel: [w1945] -> w1894
                                shift-right: [w1941] -> w1895
                                shift-left: w1896 -> [w1940]
                                n396 = Number To Fractional String(number=w1956, precision (6)=i16 2) -> (F-format string=w1951:string)  [unwired: 2 in]
                                n397 = for {
                                N: 32 -> [_]
                                shift-right: [w1971] -> w1953
                                shift-left: w1954 -> [w1971]
                                tunnel: w1951 -> [w1970]
                                tunnel: [w1970] -> w1943 mode=indexing
                                tunnel: [w1969] -> w1945 mode=indexing
                                tunnel: w1946 -> [w1969]
                                }
                                n398 = call "Ke2400 Configure Output.vi"("error in (no error)"=w1953, "Output Level (0)"=w1956, "VISA resource name"=w1962) -> ("error out"=w1963:errorcluster, "VISA resource name out"=w1961:refnum<visa-resource-name>)  [unwired: 7 in]
                                n399 = Concatenate Strings("Testing CS " ("string"), w1951) -> (w1955:string)
                                n400 = call <vilib>:"Space Constant.vi"() -> ("String"=w1960:string)
                                n401 = call "WS1021 ADI Read 64 DUT.vi"("FPGA"=w1965, "Error In"=w1963) -> ("Error Out"=w1964:errorcluster, "AD7747 Values"=w1968:string[][])  [unwired: 8 in]
                                n402 = Concatenate Strings(w1955, w1960, w1946) -> (w1959:string)
                                n403 = local write "Status"(w1959) -> ()
                                n404 = Index Array(array=w1968, index (col)=5 ("disabled index (col)")) -> (element=w1950:string[])  [unwired: 1 in]
                                n405 = Index Array(array=w1968, index (col)=2 ("disabled index (col)")) -> (element=w1944:string[])  [unwired: 1 in]
                                n406 = Build Array(w1943, w1950) -> (w1947:string[][])
                                n407 = Build Array(w1943, w1944) -> (w1942:string[][])
                                n408 = Build Array (concatenate)(w1940, w1942) -> (w1941:string[][])
                                n409 = Build Array (concatenate)(w1949, w1947) -> (w1948:string[][])
                              }
                              n410 = call "Ke2400 Configure Output.vi"("error in (no error)"=w1909, "Output Level (0)"=0.0, "VISA resource name"=w1902) -> ("error out"=w1908:errorcluster, "VISA resource name out"=w1906:refnum<visa-resource-name>)  [unwired: 7 in]
                              n411 = Build Array (concatenate)(w1892, w1894, w1895) -> (w1893:string[][])
                              n412 = Build Array (concatenate)(w1900, w1894, w1898) -> (w1899:string[][])
                              n413 = case shown="True" w1889 {
                                tunnel: w1911 -> [w1917 _]
                                tunnel: w1908 -> [w1916 w1925]
                                tunnel: [w1915 w1923] -> w1897
                                tunnel: w1891 -> [w1914 w1921]
                                frame False {
                                n414 = call "WSVCAP SHL Host TL RFFE Write - Multiple DUTs - Common Data.vi"("Data Out"=w1917, "error in"=w1916, "FPGA"=w1914, "Log (T)"=FALSE) -> ("error out"=w1915:errorcluster)  [unwired: 11 in]
                                }
                                frame True {
                                n415 = call "WSVCAP SHL Host TL RFFE Write - Multiple DUTs - Common Data.vi"("Data Out"="074200", "error in"=w1925, "FPGA"=w1921, "Log (T)"=FALSE) -> ("error out"=w1922:errorcluster)  [unwired: 11 in]
                                n416 = call "WSVCAP SHL Host TL RFFE Write - Multiple DUTs - Common Data.vi"("Data Out"="074300", "error in"=w1922, "FPGA"=w1921, "Log (T)"=FALSE) -> ("error out"=w1923:errorcluster)  [unwired: 11 in]
                                }
                              }
                            }
                            n417 = case shown="True" w1858 {
                              tunnel: [w1879 w1888] -> w1842
                              tunnel: w1855 -> [w1881 w1886]
                              tunnel: [w1881 w1885] -> w1853
                              tunnel: w1851 -> [_ w1887]
                              tunnel: [_ w1884] -> w1847
                              tunnel: [_ w1883] -> w1846
                              tunnel: [_ w1882] -> w1844
                              frame False {
                                w1880 = string[][] []
                                n418 = Build Array (concatenate)(w1880, w1880, w1880) -> (w1879:string[][])
                              }
                              frame True {
                                n419 = call "WS1021 CS 3 Voltages Output.vi"("Error In"=w1886, "Data In"=w1887) -> ("Error Out"=w1885:errorcluster, "3V Vcs Data"=w1882:string[][], "0V Vcs Data"=w1884:string[][], "-3V Vcs Data"=w1883:string[][])  [unwired: 5 in, 1 out]
                                n420 = Build Array (concatenate)(w1883, w1884, w1882) -> (w1888:string[][])
                              }
                            }
                            n421 = case shown="True" w1857 {
                              tunnel: [w1869 w1878] -> w1838
                              tunnel: w1855 -> [w1871 w1876]
                              tunnel: [w1871 w1875] -> w1854
                              tunnel: w1850 -> [_ w1877]
                              tunnel: [_ w1874] -> w1841
                              tunnel: [_ w1873] -> w1840
                              tunnel: [_ w1872] -> w1839
                              frame False {
                                w1870 = string[][] []
                                n422 = Build Array (concatenate)(w1870, w1870, w1870) -> (w1869:string[][])
                              }
                              frame True {
                                n423 = call "WS1021 CS 3 Voltages Output.vi"("Error In"=w1876, "Data In"=w1877) -> ("Error Out"=w1875:errorcluster, "3V Vcs Data"=w1872:string[][], "0V Vcs Data"=w1873:string[][], "-3V Vcs Data"=w1874:string[][])  [unwired: 5 in, 1 out]
                                n424 = Build Array (concatenate)(w1874, w1873, w1872) -> (w1878:string[][])
                              }
                            }
                            n425 = Transpose 2D Array(2D array=w1846) -> (transposed array=→"Brd B_CS_V1 (fF)":string[][])
                            n426 = Transpose 2D Array(2D array=w1847) -> (transposed array=→"Brd B_CS_V2 (fF)":string[][])
                            n427 = Transpose 2D Array(2D array=w1844) -> (transposed array=→"Brd B_CS_V3 (fF)":string[][])
                            n428 = Transpose 2D Array(2D array=w1841) -> (transposed array=→"Brd A_CS_V1 (fF)":string[][])
                            n429 = Transpose 2D Array(2D array=w1840) -> (transposed array=→"Brd A_CS_V2 (fF)":string[][])
                            n430 = Transpose 2D Array(2D array=w1839) -> (transposed array=→"Brd A_CS_V3 (fF)":string[][])
                            n431 = Merge Errors(w1853, w1854) -> (w1849:errorcluster)
                          }
                        }
                        n432 = Index Array(array=w1715, index=2) -> (element=w1710:dbl)
                        n433 = case shown="True" w1711 {
                          tunnel: w1721 -> [w1748 w1771]
                          tunnel: [w1747 w1770] -> w1720
                          tunnel: [w1749 w1769] -> w1702
                          tunnel: [w1750 w1768] -> w1714
                          tunnel: w1710 -> [_ w1766]
                          tunnel: [w1750 w1767] -> w1713
                          tunnel: w1710 -> [_ w1765]
                          tunnel: w1705 -> [_ w1764]
                          tunnel: w1704 -> [_ w1763]
                          frame False {
                            n434 = for {
                              N: 14 -> [_]
                              tunnel: [w1757] -> w1750 mode=indexing
                              shift-right: [w1755] -> w1749
                              shift-left: w1748 -> [w1756]
                              shift-right: [w1753] -> w1747
                              shift-left: w1748 -> [w1754]
                              n435 = for {
                                N: 31 -> [_]
                                tunnel: ["na"] -> w1759 mode=indexing
                                shift-right: [w1761] -> w1755
                                shift-left: w1756 -> [w1761]
                                shift-right: [w1760] -> w1753
                                shift-left: w1754 -> [w1760]
                              }
                              n436 = Build Array (concatenate)("na", w1759) -> (w1757:string[])
                            }
                          }
                          frame True {
                            n437 = case shown="True" w1764 {
                              tunnel: w1771 -> [w1782 w1789]
                              tunnel: [w1782 w1788] -> w1770
                              tunnel: [string[][] [] ("VCmin") w1784] -> w1768
                              tunnel: w1766 -> [_ w1783]
                              frame False {
                              }
                              frame True {
                                n438 = local read "Brd B_CS_V1 (fF)"() -> (w1787:string[][])
                                n439 = local read "Brd B_CS_V2 (fF)"() -> (w1786:string[][])
                                n440 = local read "Brd B_CS_V3 (fF)"() -> (w1785:string[][])
                                n441 = call "WS102x_Multi DUT_Calculate VCMIN.vi"("Pos_Voltage(V)"=w1783, "error in (no error)"=w1789, "V3_VCmin"=w1785, "V2_VCmin"=w1786, "V1_VCmin"=w1787) -> ("error out"=w1788:errorcluster, "VCmin"=w1784:string[][])  [unwired: 5 in]
                              }
                            }
                            n442 = case shown="True" w1763 {
                              tunnel: w1771 -> [w1773 w1780]
                              tunnel: [w1773 w1779] -> w1769
                              tunnel: [string[][] [] ("VCmin") w1775] -> w1767
                              tunnel: w1765 -> [_ w1774]
                              frame False {
                              }
                              frame True {
                                n443 = local read "Brd A_CS_V1 (fF)"() -> (w1778:string[][])
                                n444 = local read "Brd A_CS_V2 (fF)"() -> (w1777:string[][])
                                n445 = local read "Brd A_CS_V3 (fF)"() -> (w1776:string[][])
                                n446 = call "WS102x_Multi DUT_Calculate VCMIN.vi"("Pos_Voltage(V)"=w1774, "error in (no error)"=w1780, "V3_VCmin"=w1776, "V2_VCmin"=w1777, "V1_VCmin"=w1778) -> ("error out"=w1779:errorcluster, "VCmin"=w1775:string[][])  [unwired: 5 in]
                              }
                            }
                          }
                        }
                        n447 = case shown="0" w1724 {
                          tunnel: w1702 -> [w1790 w1796]
                          tunnel: [w1790 w1796] -> w1718
                          tunnel: w1714 -> [w1795 w1801]
                          tunnel: w1713 -> [w1793 w1799]
                          tunnel: w1720 -> [w1791 w1797]
                          tunnel: [w1791 w1797] -> w1717
                          frame 0 {
                            n448 = Transpose 2D Array(2D array=w1795) -> (transposed array=→"Brd B_CS VCmin_T0":string[][])
                            n449 = Transpose 2D Array(2D array=w1793) -> (transposed array=→"Brd A_CS VCmin_T0":string[][])
                          }
                          frame 1, Default {
                            n450 = Transpose 2D Array(2D array=w1801) -> (transposed array=→"Brd B_CS VCmin":string[][])
                            n451 = Transpose 2D Array(2D array=w1799) -> (transposed array=→"Brd A_CS VCmin":string[][])
                          }
                        }
                        n452 = Merge Errors(w1717, w1718) -> (w1719:errorcluster)
                        n453 = call "Ke2400 Configure Output.vi"("error in (no error)"=w1719, "Output Level (0)"=0.0, "VISA resource name"=w1737) -> ("error out"=w1738:errorcluster, "VISA resource name out"=w1736:refnum<visa-resource-name>)  [unwired: 7 in]
                        n454 = flat-sequence {
                          tunnel: w1738 -> [w1974]
                          tunnel: [w1973] -> w1745
                          tunnel: [Test_Sequences."Save Data" ("Test Sequences")] -> w1746
                          tunnel: w1734 -> [w1983]
                          tunnel: [w1982] -> w1733
                          tunnel: w1732 -> [w1981]
                          tunnel: [w1980] -> w1731
                          tunnel: w1723 -> [w1979]
                          tunnel: w1722 -> [w1978]
                          tunnel: w1714 -> [w1977]
                          tunnel: w1713 -> [w1976]
                          tunnel: [w1972] -> w1706
                          frame #0 {
                            n455 = case shown="Error" w1974 {
                              selector: w1974 -> [w1985 _]
                              tunnel: [w1985 errorcluster {"status"=FALSE, "code"=0, "source"=""} ("error IO")] -> w1973
                              tunnel: ["0" "4"] -> w1972
                              frame No Error {
                              }
                              frame Error {
                              }
                            }
                            n456 = Build Array (concatenate)(w1981, w1978, w1976) -> (w1980:string[][])
                            n457 = Build Array (concatenate)(w1983, w1979, w1977) -> (w1982:string[][])
                          }
                        }
                      }
                      frame "Save Data" {
                        w2003 = FALSE ("true")
                        n458 = for {
                          N: 32 -> [_]
                          shift-right: [w2036] -> w2019
                          shift-left: w2020 -> [w2036]
                          tunnel: w2017 -> [w2035]
                          tunnel: [w2035] -> w1993 mode=indexing
                          tunnel: w2016 -> [w2034]
                          tunnel: [w2034] -> w2015 mode=indexing
                          tunnel: w2014 -> [w2033]
                          tunnel: [w2033] -> w2013 mode=indexing
                        }
                        n459 = call "WS1021 Multi DUT Generate Header Ver1.5.vi"("Reg 3"=w2008, "VPI Name"=w2006, "Reg 2"=w2007, "Error In"=w2019) -> ("Header"=w2021:string[], "Error Out"=w2025:errorcluster)  [unwired: 10 in]
                        n460 = Build Array (concatenate)(w1994, w1993, w2015) -> (w2010:string[][])
                        n461 = case shown="True" w1991 {
                          tunnel: w2012 -> [_ w2082]
                          tunnel: w2025 -> [w2078 w2083]
                          tunnel: [w2078 w2084] -> w1997
                          tunnel: w2021 -> [_ w2081]
                          tunnel: w2004 -> [_ w2080]
                          tunnel: w2010 -> [_ w2079]
                          tunnel: [string[][] [] w2079] -> w1989
                          frame False {
                          }
                          frame True {
                            # "Save Data Brd B"
                            n462 = call "WS1021_32DUT_Save Data_Ver1.0.vi"("Header"=w2081, "File Name"=w2080, "error in (no error)"=w2083, "base path"=w2082, "Data In"=w2079) -> ("error out"=w2084:errorcluster)  [unwired: 13 in, 1 out]
                          }
                        }
                        "Data Board B" <- w1989
                        n463 = Build Array (concatenate)(w1995, w1993, w2013) -> (w2009:string[][])
                        n464 = case shown="True" w1992 {
                          tunnel: w2011 -> [_ w2074]
                          tunnel: w2025 -> [w2070 w2075]
                          tunnel: [w2070 w2076] -> w2000
                          tunnel: w2021 -> [_ w2073]
                          tunnel: w2005 -> [_ w2072]
                          tunnel: w2009 -> [_ w2071]
                          tunnel: [string[][] [] w2071] -> w1988
                          frame False {
                          }
                          frame True {
                            # "Save Data Brd A"
                            n465 = call "WS1021_32DUT_Save Data_Ver1.0.vi"("Header"=w2073, "File Name"=w2072, "error in (no error)"=w2075, "base path"=w2074, "Data In"=w2071) -> ("error out"=w2076:errorcluster)  [unwired: 13 in, 1 out]
                          }
                        }
                        "Data Board A" <- w1988
                        n466 = local write "Status"("Save Data and Plot" ("Status")) -> ()
                        n467 = call "Time Delay.vi"("Error In"=w2000, "Delay(ms)"=u32 250) -> ("Error Out"=w2001:errorcluster)  [unwired: 9 in]
                        n468 = call "Time Delay.vi"("Error In"=w1997, "Delay(ms)"=u32 250) -> ("Error Out"=w1998:errorcluster)  [unwired: 9 in]
                        n469 = flat-sequence {
                          tunnel: w2001 -> [w2048]
                          tunnel: w1998 -> [w2050]
                          tunnel: [w2049] -> w2024
                          tunnel: [w2047] -> w2023
                          tunnel: w2012 -> [w2045]
                          tunnel: w2011 -> [w2043]
                          tunnel: w2005 -> [w2040]
                          tunnel: w2004 -> [w2039]
                          tunnel: w1992 -> [w2038]
                          tunnel: w1991 -> [w2037]
                          frame #0 {
                            # "Plots"
                            n470 = case shown="False" w2038 {
                              tunnel: w2048 -> [w2052 w2059]
                              tunnel: [w2052 w2058] -> w2047
                              tunnel: "Col CMin" -> [_ w2057]
                              tunnel: "Plot" -> [_ w2056]
                              tunnel: w2043 -> [_ w2055]
                              tunnel: [dbl[][] [] ("Delta COFF Plot (fF)") w2054] -> w2041
                              tunnel: w2040 -> [_ w2053]
                              frame False {
                              }
                              frame True {
                                n471 = call "WS1021 Multi DUT COFF Plots.vi"("Col CMin"=w2057, "File Name"=w2053, "Plot"=w2056, "file path (dialog if empty)"=w2055, "Error In"=w2059) -> ("Delta COFF Plot (fF)"=w2054:dbl[][], "Error Out"=w2058:errorcluster)  [unwired: 9 in]
                              }
                            }
                            n472 = case shown="False" w2037 {
                              tunnel: w2050 -> [w2061 w2068]
                              tunnel: [w2061 w2067] -> w2049
                              tunnel: "Col CMin" -> [_ w2066]
                              tunnel: w2045 -> [_ w2065]
                              tunnel: "Plot" -> [_ w2064]
                              tunnel: [dbl[][] [] ("Delta COFF Plot (fF)") w2063] -> w2042
                              tunnel: w2039 -> [_ w2062]
                              frame False {
                              }
                              frame True {
                                n473 = call "WS1021 Multi DUT COFF Plots.vi"("Col CMin"=w2066, "File Name"=w2062, "Plot"=w2064, "file path (dialog if empty)"=w2065, "Error In"=w2068) -> ("Delta COFF Plot (fF)"=w2063:dbl[][], "Error Out"=w2067:errorcluster)  [unwired: 9 in]
                              }
                            }
                            n474 = local write "Board B"(w2042) -> ()
                            n475 = local write "Board A"(w2041) -> ()
                          }
                        }
                        n476 = Merge Errors(w2024, w2023) -> (w2022:errorcluster)
                        n477 = flat-sequence {
                          tunnel: w2022 -> [w2091]
                          tunnel: [w2091] -> w2032
                          tunnel: [Test_Sequences."Exit" ("Test Sequences")] -> w2031
                          tunnel: [""] -> w1990
                          frame #0 {
                            n478 = Get Date/Time In Seconds() -> (seconds since 1Jan1904=w2090:timestamp)
                            n479 = Get Date/Time String(seconds (now)=w2090, want seconds? (F)=TRUE) -> (date string=→"Last Run Date":string, time string=→"Last Run Time":string)  [unwired: 1 in]
                          }
                        }
                      }
                      frame "Exit", Default {
                        n480 = flat-sequence {
                          tunnel: w2121 -> [w2141]
                          tunnel: "Set TTF" -> [w2143]
                          tunnel: [w2142] -> w2119
                          tunnel: [w2141] -> w2118
                          tunnel: [w2140] -> w2107
                          tunnel: w2119 -> [w2154]
                          tunnel: w2118 -> [w2153]
                          tunnel: [w2152] -> w2104
                          tunnel: [w2151] -> w2117
                          tunnel: w2113 -> [w2150]
                          tunnel: [w2149] -> w2110
                          tunnel: w2112 -> [w2148]
                          tunnel: [w2147] -> w2111
                          tunnel: w2107 -> [w2146]
                          tunnel: [w2146] -> w2106
                          tunnel: [w2145] -> w2100
                          frame #0 {
                            n481 = local read "TTF Completed"() -> (w2140:u64)
                            n482 = Greater Or Equal?(x=w2140, y=w2143) -> (x >= y?=w2142:bool)
                          }
                          frame #1 {
                            n483 = case shown="True" w2154 {
                              tunnel: w2153 -> [w2157 w2166]
                              tunnel: [FALSE ("true") w2164] -> w2152
                              tunnel: [w2157 w2163] -> w2151
                              tunnel: w2150 -> [w2156 w2162]
                              tunnel: [w2156 w2161] -> w2149
                              tunnel: w2148 -> [w2155 w2160]
                              tunnel: [w2155 w2159] -> w2147
                              frame False {
                              }
                              frame True {
                                n484 = flat-sequence {
                                tunnel: w2166 -> [w2176]
                                tunnel: [w2172] -> w2165
                                tunnel: w2162 -> [w2171]
                                tunnel: [w2170] -> w2161
                                tunnel: w2160 -> [w2169]
                                tunnel: [w2168] -> w2159
                                tunnel: w2165 -> [w2182]
                                tunnel: [w2183] -> w2164
                                tunnel: [w2182] -> w2163
                                frame #0 {
                                w2167 = u16 0 items=["Voltage", "Current"] ("Source Mode  (0: Voltage)")
                                w2179 = 0.0 ("Voltage 1")
                                n485 = call "E3631A_Voltage Controller updated.vi"("VISA resource name"=w2169, "I_VDD(A)"=w2179, "Channel Controller"=T14."Voltage 1", "Voltage 1"=w2179, "Voltage 2"=3.3, "error in (no error)"=w2176, "I_3.3V (A)"=0.5) -> ("VISA resource name out"=w2168:refnum<visa-resource-name>, "error out"=w2174:errorcluster)  [unwired: 7 in]
                                n486 = call "Ke2400 Configure Output.vi"("Source Mode  (0: Voltage)"=w2167, "error in (no error)"=w2176, "Output Level (0)"=0.0, "VISA resource name"=w2171) -> ("error out"=w2173:errorcluster, "VISA resource name out"=w2170:refnum<visa-resource-name>)  [unwired: 6 in]
                                n487 = Merge Errors(w2173, w2174) -> (w2172:errorcluster)
                                }
                                frame #1 {
                                w2181 = "Completed!" ("message")
                                n488 = local write "Status"(w2181) -> ()
                                n489 = One Button Dialog(message=w2181) -> (true=w2183:bool)  [unwired: 1 in]
                                }
                                }
                              }
                            }
                            n490 = Number To Fractional String(number=w2146, precision (6)=i16 0) -> (F-format string=w2145:string)  [unwired: 2 in]
                          }
                        }
                        n491 = case shown="True" w2101 {
                          tunnel: w2117 -> [w2131 w2139]
                          tunnel: w2096 -> [_ w2138]
                          tunnel: w2116 -> [_ w2137]
                          tunnel: w2115 -> [_ w2136]
                          tunnel: w2114 -> [_ w2135]
                          tunnel: w2100 -> [_ w2134]
                          tunnel: w2093 -> [_ w2133]
                          tunnel: [w2131 w2132] -> w2099
                          frame False {
                          }
                          frame True {
                            n492 = call "Save Errors Status.vi"("Lot"=w2137, "Stress"=w2134, "Wafer"=w2136, "error in (no error)"=w2139, "File Name"=w2135, "Error Status"=w2133, "base path"=w2138) -> ("error out"=w2132:errorcluster)  [unwired: 4 in]
                          }
                        }
                        n493 = case shown="True" w2097 {
                          tunnel: w2100 -> [_ w2130]
                          tunnel: w2099 -> [w2122 w2129]
                          tunnel: [w2122 w2128] -> w2098
                          tunnel: w2096 -> [_ w2127]
                          tunnel: w2095 -> [_ w2126]
                          tunnel: w2094 -> [_ w2125]
                          tunnel: w2093 -> [_ w2124]
                          tunnel: w2092 -> [_ w2123]
                          frame False {
                          }
                          frame True {
                            n494 = call "Save Errors Status.vi"("Lot"=w2126, "Stress"=w2130, "Wafer"=w2125, "error in (no error)"=w2129, "File Name"=w2123, "Error Status"=w2124, "base path"=w2127) -> ("error out"=w2128:errorcluster)  [unwired: 4 in]
                          }
                        }
                      }
                    }
                    "Test Sequences" <- w309
                    n495 = local write "Data Board A"(w250) -> ()
                    n496 = Concatenate Strings(w245, w247) -> (w246:string)
                    n497 = local write "Data Board B"(w251) -> ()
                    n498 = local write "Error Status"(w246) -> ()
                    n499 = Or(x=w289, y=w290) -> (x .or. y?=w291:bool)
                    n500 = call "Time Delay.vi"("Error In"=w289, "Delay(ms)"=u32 10) -> ("Error Out"=w301:errorcluster)  [unwired: 9 in]
                  }
                  n501 = call "Time Delay.vi"("Error In"=w170, "Delay(ms)"=u32 100) -> ("Error Out"=w173:errorcluster)  [unwired: 9 in]
                  n502 = Compound Arithmetic op=OR(w170, w169, w168) -> (w171:bool)
                }
                "Status" <- "Idle...." ("Status")
              }
              frame True {
              }
            }
            n503 = local write "Abort Stress"(FALSE ("Abort Stress")) -> ()
            n504 = Or(x=w92, y=w91) -> (x .or. y?=w93:bool)
          }
        }
        frame Error {
          n505 = flat-sequence {
            tunnel: w2348 -> [w2350]
            tunnel: [w2350] -> w2347
            tunnel: [w2349] -> _
            frame #0 {
              n506 = One Button Dialog(message="Communication Errors?") -> (true=w2349:bool)  [unwired: 1 in]
            }
          }
        }
      }
    }
    frame #2 {
      n507 = call "TLTSP_Close.vi"("error in (no error)"=w2354, "VISA In"=w2371) -> ("error out"=w2357:errorcluster, "VISA Out"=w2361:refnum<visa-resource-name>)  [unwired: 8 in]
      n508 = call "WSVCAP SHL Host TL Close.vi"("error in"=w2354, "FPGA"=w2353) -> ("error out"=w2352:errorcluster)  [unwired: 13 in]
      n509 = call "Ke2400 Enable.vi"("error in (no error)"=w2354, "ON/OFF"=FALSE, "VISA In"=w2366) -> ("error out"=w2359:errorcluster, "VISA Out"=w2364:refnum<visa-resource-name>)  [unwired: 7 in]
      n510 = call "E3631A_Voltage Controller updated.vi"("VISA resource name"=w2370, "I_VDD(A)"=0.5, "Channel Controller"=T14."Voltage 1", "Voltage 1"=0.0, "error in (no error)"=w2354) -> ("VISA resource name out"=w2362:refnum<visa-resource-name>, "error out"=w2358:errorcluster)  [unwired: 9 in]
      n511 = Build Array(w2364, w2363, w2362, w2361) -> (w2360:refnum<visa-resource-name>[])
      n512 = Merge Errors(w2359, w2358, w2357, w2352) -> (w2356:errorcluster)
      n513 = for {
        tunnel: w2360 -> [w2375] mode=indexing
        tunnel: w2356 -> [w2374]
        tunnel: [w2373] -> w2355
        n514 = VISA Close(VISA resource name=w2375, error in (no error)=w2374) -> (error out=w2373:errorcluster)
        n515 = Wait (ms)(milliseconds to wait=u32 10) -> ()  [unwired: 1 out]
      }
    }
  }
  "Error Out" <- w15
